vi "ER2007 Get Cell Data.vi"() -> ()   [LabVIEW 2013]
uses:
  <vilib>/Platform/TimedLoop/XDataNode/timing_clust.ctl
  <vilib>/Platform/TimedLoop/XDataNode/nitl_modes.ctl
  <vilib>/Platform/TimedLoop/XDataNode/wakeup.ctl
  Controls/Global ER2007.vi
  <vilib>/platform/TimedLoop/XDataNode/XDataNode.xnode
  <vilib>/Platform/TimedLoop/XDataNode/XDNodeRunTimeDep.lvlib
panel:
  in  "Force Recalc":bool
  out "Last Resistor":T1(ring)
  out "Swch Box":bool[](array[boolean])
  out "NAII Live":bool
  out "HP Live":bool
  out "Cell ID":i32
  out "RS Done":bool
  out "NAI Errcnt":i32
  out "ResistParams":T2 {"R13 (k)" format="%.5f"; "R3G (k)" format="%.5f"; "R23 (k)" format="%.5f"; "R12 (k)" format="%.5f"; "R2P (k)" format="%.5f"}
  out "VI Time":dbl format="%.2f"
  out "B 3":bool
  out "B 2":bool
  out "B 1":bool
  out "Errs":bool[](array[boolean])
  out "SecPh":i32
  out "PriPh":i32
  out "Abort Message":string
  out "Test Info Out":T3 {"Cell Data"."Rw Temp" format="%.2f"; "Cell Data"."Rw" format="%.2f"; "Cell Data"."DAQ Units" items=["Mins", "Hrs"]; "Cell Data"."CurData" format="%.3f"; "Cell Data"."Last Pore Vol" format="%.3f"; "Cell Data"."Amplitude" format="%.3f"; "Cell Data"."ElectSpace" format="%.2f"; "Cell Data"."Permeability" format="%.2f"; "Cell Data"."Porosity" format="%.2f"; "Cell Data"."Diameter" format="%.2f"; "Cell Data"."Length" format="%.2f"}
  in  "Test Info In":T3={"CurCell"=0, "Cell Data"=[{"Cell ID"=1, "Cell Status"=enum."Active", "Project"="Project C1", "Sample #"="Sample C1", "Rock Type"="Rock C1", "Fluid Pair"="Fluid Pair C1", "Rw"=0.0, "Rw Temp"=0.0, "Length"=5.08, "Diameter"=2.54, "Porosity"=1.23, "Permeability"=2.34, "4P"=FALSE, "ElectSpace"=2.54, "Frequency"=1000.0, "Amplitude"=1.0, "DAQ Period"=10, "DAQ Units"=0, "Start Time"=0.0, "Next Time"=0.0, "Datafile"=path "C:/ER2006/Data/Dummy Cell 1 Test.dat", "Last Pore Vol"=9.876, "Last Pore Xdcr"=enum."<none>", "Last Resistor"=enum."<none>", "CurData"=[], "Comment"=""}, {"Cell ID"=2, "Cell Status"=enum."Active", "Project"="Project C2", "Sample #"="Sample C2", "Rock Type"="Rock C2", "Fluid Pair"="Fluid Pair C2", "Rw"=0.0, "Rw Temp"=0.0, "Length"=5.08, "Diameter"=2.54, "Porosity"=2.34, "Permeability"=3.45, "4P"=FALSE, "ElectSpace"=2.54, "Frequency"=1000.0, "Amplitude"=1.0, "DAQ Period"=20, "DAQ Units"=0, "Start Time"=0.0, "Next Time"=0.0, "Datafile"=path "C:/ER2006/Data/Dummy Cell 2 Test.dat", "Last Pore Vol"=8.765, "Last Pore Xdcr"=enum."<none>", "Last Resistor"=enum."<none>", "CurData"=[], "Comment"=""}, {"Cell ID"=3, "Cell Status"=enum."Active", "Project"="Project C3", "Sample #"="Sample C3", "Rock Type"="Rock C3", "Fluid Pair"="Fluid Pair C3", "Rw"=0.0, "Rw Temp"=0.0, "Length"=5.0, "Diameter"=3.7, "Porosity"=3.45, "Permeability"=4.56, "4P"=FALSE, "ElectSpace"=2.54, "Frequency"=20000.0, "Amplitude"=1.0, "DAQ Period"=30, "DAQ Units"=0, "Start Time"=0.0, "Next Time"=0.0, "Datafile"=path "C:/ER2006/Data/Dummy Cell 3 Test.dat", "Last Pore Vol"=7.654, "Last Pore Xdcr"=enum."<none>", "Last Resistor"=enum."Resistor 1", "CurData"=[], "Comment"=""}, {"Cell ID"=4, "Cell Status"=enum."Active", "Project"="Project C4", "Sample #"="Sample C4", "Rock Type"="Rock C4", "Fluid Pair"="Fluid Pair C4", "Rw"=0.0, "Rw Temp"=0.0, "Length"=5.08, "Diameter"=2.54, "Porosity"=4.56, "Permeability"=5.67, "4P"=FALSE, "ElectSpace"=2.54, "Frequency"=1000.0, "Amplitude"=1.0, "DAQ Period"=40, "DAQ Units"=0, "Start Time"=0.0, "Next Time"=0.0, "Datafile"=path "C:/ER2006/Data/Dummy Cell 4 Test.dat", "Last Pore Vol"=6.543, "Last Pore Xdcr"=enum."<none>", "Last Resistor"=enum."<none>", "CurData"=[], "Comment"=""}, {"Cell ID"=5, "Cell Status"=enum."Active", "Project"="Project C5", "Sample #"="Sample C5", "Rock Type"="Rock C5", "Fluid Pair"="Fluid Pair C5", "Rw"=0.0, "Rw Temp"=0.0, "Length"=5.08, "Diameter"=2.54, "Porosity"=5.67, "Permeability"=6.78, "4P"=FALSE, "ElectSpace"=2.54, "Frequency"=1000.0, "Amplitude"=1.0, "DAQ Period"=50, "DAQ Units"=0, "Start Time"=0.0, "Next Time"=0.0, "Datafile"=path "C:/ER2006/Data/Dummy Cell 5 Test.dat", "Last Pore Vol"=5.432, "Last Pore Xdcr"=enum."<none>", "Last Resistor"=enum."Resistor 1", "CurData"=[], "Comment"=""}]} {"Cell Data"."Rw Temp" format="%.2f"; "Cell Data"."Rw" format="%.2f"; "Cell Data"."DAQ Units" items=["Mins", "Hrs"]; "Cell Data"."CurData" format="%.3f"; "Cell Data"."Last Pore Vol" format="%.3f"; "Cell Data"."Amplitude" format="%.3f"; "Cell Data"."ElectSpace" format="%.2f"; "Cell Data"."Permeability" format="%.2f"; "Cell Data"."Porosity" format="%.2f"; "Cell Data"."Diameter" format="%.2f"; "Cell Data"."Length" format="%.2f"}
  in  "DataCell":i32=1 min=1 max=5
  in  "Local Test Resistivity Input Data (sim)":dbl[][][](array[numeric])=[[[1.4142, 0.0], [0.5636, -0.41164], [0.4615, -0.53147], [0.1638, -0.11556]], [[1.4071, 0.0], [1.0986, -3.46], [0.7889, -7.95], [0.4213, -10.11]], [[1.4142, 0.0], [1.0607, 0.0], [0.7071, 0.0], [0.3536, 0.0]], [[1.4142, 0.0], [1.0607, -8.1e-05], [0.7778, -0.000127], [0.4243, -0.000189]], [[1.4142, 0.0], [0.1951, -0.00032], [0.1341, -0.0004], [0.0366, -8e-05]], [[1.4142, 0.0], [0.6923, -1.418851], [0.4974, -1.822365], [0.13, 0.58215]], [[1.4142, 0.0], [0.7408, -0.08646], [0.5387, -0.11405], [0.1347, 0.03607]], [[1.4142, 0.0], [0.6852, -0.060094], [0.4884, -0.071822], [0.1604, -0.002912]]] format="%.5f"
  in  "Use Locals":bool
  out "Resistivity Data":dbl[][](array[numeric]) format="%.5f"
  out "Stored State":T4(ring)
  out "State":T4(ring)
  in  "SimOn":bool
  in  "Stop":bool
  in  "Go":bool
  # "Dev 1 Assignments\n DIO             DigInv\n Chl   Chl Desc  Index\n-----  --------  ------\nP0.0   Shunt 1     0\nP0.1   SCL1        1\nP0.2   SCL2        2\nP0.3   Shunt 2     3\nP0.4   AutoEnb     4\nP0.5   RSCL1       5\nP0.6   Shunt 3     6\nP0.7   RSCL2       7\nP0.8   <spare>     -\nP0.17  <spare>     -\nP0.18  Shunt 4    ??\nP0.21  Shunt 5    ??\nP1.0   RSCL3      16\nP1.1   YCL1       17\nP1.2   YCL2       18\nP1.3   YCL3       19\nP1.4   YCL4       20\nP1.5   <spare>     -\nP1.6   Lockout    21\nP1.7   <spare>     -"
  # "See the Background DAQ vi for A/D\nassignments.  See Frame 0:0 of this\nvi for file and local testing info."
  # "AutoMode   Cell Sel   Resist Sel   Signal Sel"
  # "Dout"
  # "Local Test Controls"
  # "Agilent"
  # "Cell #\n\nVselect\n\nV/Phase"
  # "NAII"
  # "Calc-R"
  # "File I/O"
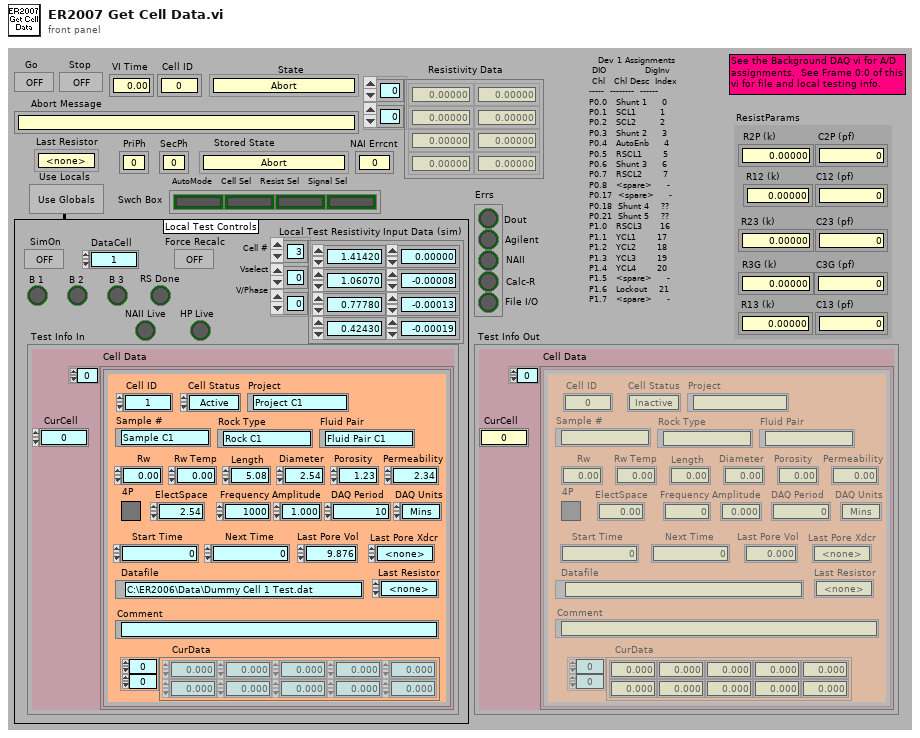
[diagram p1: front panel]
types:
  T1 = enum16{"<none>", "Resistor 1", "Resistor 2", "Resistor 3", "Resistor 4", "Resistor 5", "Resistor 6"}
  T2 = cluster{"R2P (k)":dbl, "C2P (pf)":dbl, "R12 (k)":dbl, "C12 (pf)":dbl, "R23 (k)":dbl, "C23 (pf)":dbl, "R3G (k)":dbl, "C3G (pf)":dbl, "R13 (k)":dbl, "C13 (pf)":dbl}
  T3 = cluster{"CurCell":i32, "Cell Data":cluster{"Cell ID":i32, "Cell Status":enum16{"Inactive", "Setup", "Active", "Done"}, "Project":string, "Sample #":string, "Rock Type":string, "Fluid Pair":string, "Rw":dbl, "Rw Temp":dbl, "Length":dbl, "Diameter":dbl, "Porosity":dbl, "Permeability":dbl, "4P":bool, "ElectSpace":dbl, "Frequency":dbl, "Amplitude":dbl, "DAQ Period":u32, "DAQ Units":u16, "Start Time":dbl, "Next Time":dbl, "Datafile":path, "Last Pore Vol":dbl, "Last Pore Xdcr":enum16{"<none>", "Lo Range", "Hi Range"}, "Last Resistor":enum16{"<none>", "Resistor 1", "Resistor 2", "Resistor 3", "Resistor 4", "Resistor 5", "Resistor 6"}, "CurData":dbl[][], "Comment":string}[]}
  T4 = enum16{"Abort", "Calculate Resistivity Values", "Determine Series Resistor", "Done", "Error Handler", "Final Values", "Generator OFF", "Generator ON", "Get Cell Pressures", "Get Cell Temperatures", "Get Vs & Phase", "Get V1g & Phase", "Get V2g & Phase", "Get V3g & Phase", "Idle", "Initialize", "Main Test Engine", "Reset Auto Mode", "Reset Cell Select Relays", "Reset Resistor Select Relays", "Reset Signal Select Relays", "Set Auto Mode", "Set Cell Select Relays", "Set Freq & Ampltd", "Set Resistor Select Relays", "Set Signal Select Relays", "Stop", "Wait x Secs"}
  T5 = enum16{"<none>", "Signal 1", "Signal 2", "Signal 3"}
  T6 = enum16{"TOTAL", "FUNDAMENTAL", "IN PHASE", "QUADRATURE", "PHASE ANGLE", "THD"}
  T7 = cluster{"Rseries (K)":dbl, "Frequency (Hz)":dbl, "Voltages":dbl[], "Angles":dbl[]}
  T8 = typedef "XDNodeRunTimeDep.lvlib/timing_clust.ctl" = cluster{"Expected End [f-1]":u64, "Actual End [f-1]":u64, "Finished Late? [f-1]":bool, "Expected End [i-1]":u64, "Actual End [i-1]":u64, "Finished Late? [i-1]":bool, "Expected Start [i]":u64, "Actual Start [i]":u64, "Expected Start [f]":u64, "Actual Start [f]":u64, "Source Name":string, "Structure Name":string, "Period":i64, "Deadline":i64, "Offset":i64, "Start":i64, "Priority":i32, "Timeout":i32, "Mode":T9, "Wakeup Reason":T10, "Error":errorcluster, "Source Type":string, "Secondary Source Type":string, "Global End Time":u64, "Global Start Time":u64, "Frame Duration":u64, "Iteration Duration":u64, "Assigned CPU":i32, "I/O Scan Engine Mode":u32}
  T9 = typedef "XDNodeRunTimeDep.lvlib/nitl_modes.ctl" = enum32{"No Change", "Process missed periods, maintain original phase", "Discard missed periods, maintain original phase", "Process missed periods, ignore original phase", "Discard missed periods, ignore original phase"}
  T10 = typedef "XDNodeRunTimeDep.lvlib/wakeup.ctl" = enum32{"Normal", "Aborted", "Asynchronous wakeup", "Timing source error", "Timed loop error", "Timeout"}
  T11 = cluster{"Cell ID":i32, "Cell Status":enum16{"Inactive", "Setup", "Active", "Done"}, "Project":string, "Sample #":string, "Rock Type":string, "Fluid Pair":string, "Rw":dbl, "Rw Temp":dbl, "Length":dbl, "Diameter":dbl, "Porosity":dbl, "Permeability":dbl, "4P":bool, "ElectSpace":dbl, "Frequency":dbl, "Amplitude":dbl, "DAQ Period":u32, "DAQ Units":u16, "Start Time":dbl, "Next Time":dbl, "Datafile":path, "Last Pore Vol":dbl, "Last Pore Xdcr":enum16{"<none>", "Lo Range", "Hi Range"}, "Last Resistor":enum16{"<none>", "Resistor 1", "Resistor 2", "Resistor 3", "Resistor 4", "Resistor 5", "Resistor 6"}, "CurData":dbl[][], "Comment":string}
  T12 = cluster{"Cell ID":i32, "Cell Status":enum16{"Inactive", "Setup", "Active", "Done"}, "Project":string, "Sample #":string, "Rock Type":string, "Fluid Pair":string, "Rw":dbl, "Rw Temp":dbl, "Length":dbl, "Diameter":dbl, "Porosity":dbl, "Permeability":dbl, "4P":bool, "ElectSpace":dbl, "Frequency":dbl, "Amplitude":dbl, "DAQ Period":u32, "DAQ Units":u16, "Start Time":dbl, "Next Time":dbl, "Datafile":path, "Last Pore Vol":dbl, "Last Pore Xdcr":enum16{"<none>", "Lo Range", "Hi Range"}, "Last Resistor":enum16{"<none>", "Resistor 1", "Resistor 2", "Resistor 3", "Resistor 4", "Resistor 5", "Resistor 6"}, "CurData":dbl[][], "Comment":string}[]
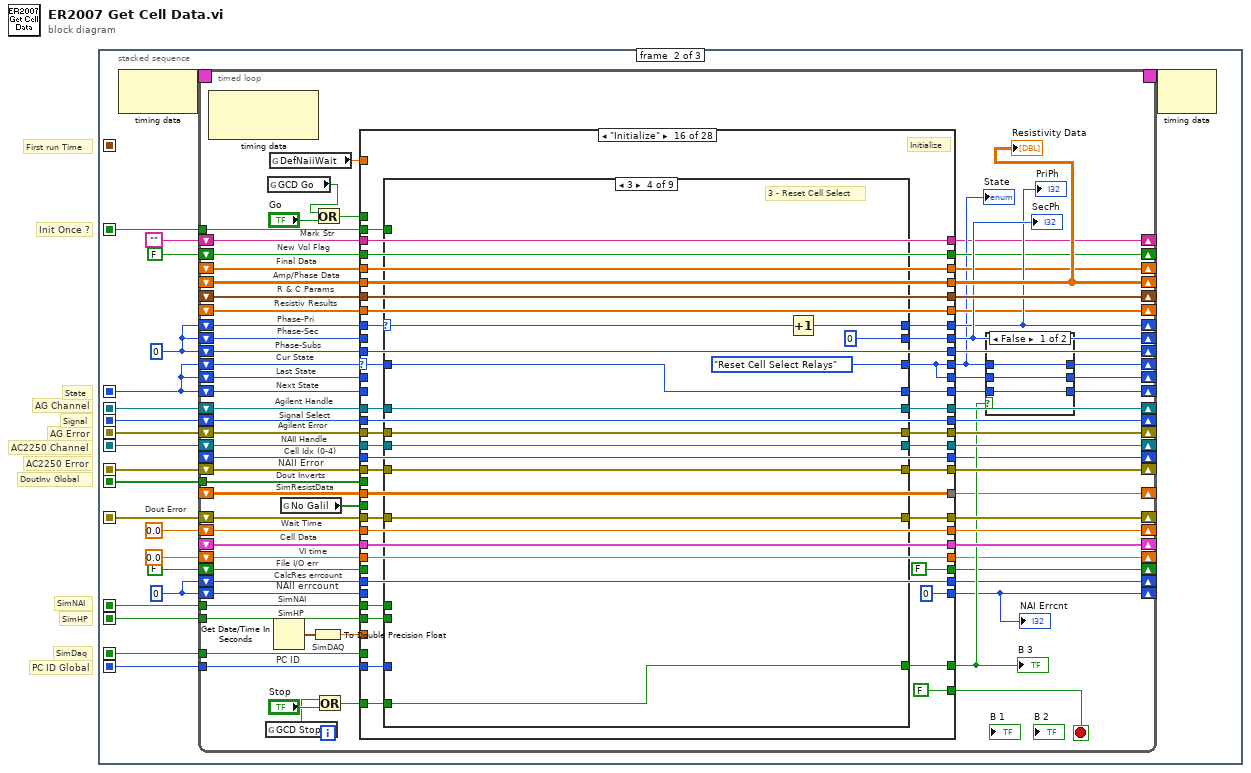
[diagram p0: block diagram]
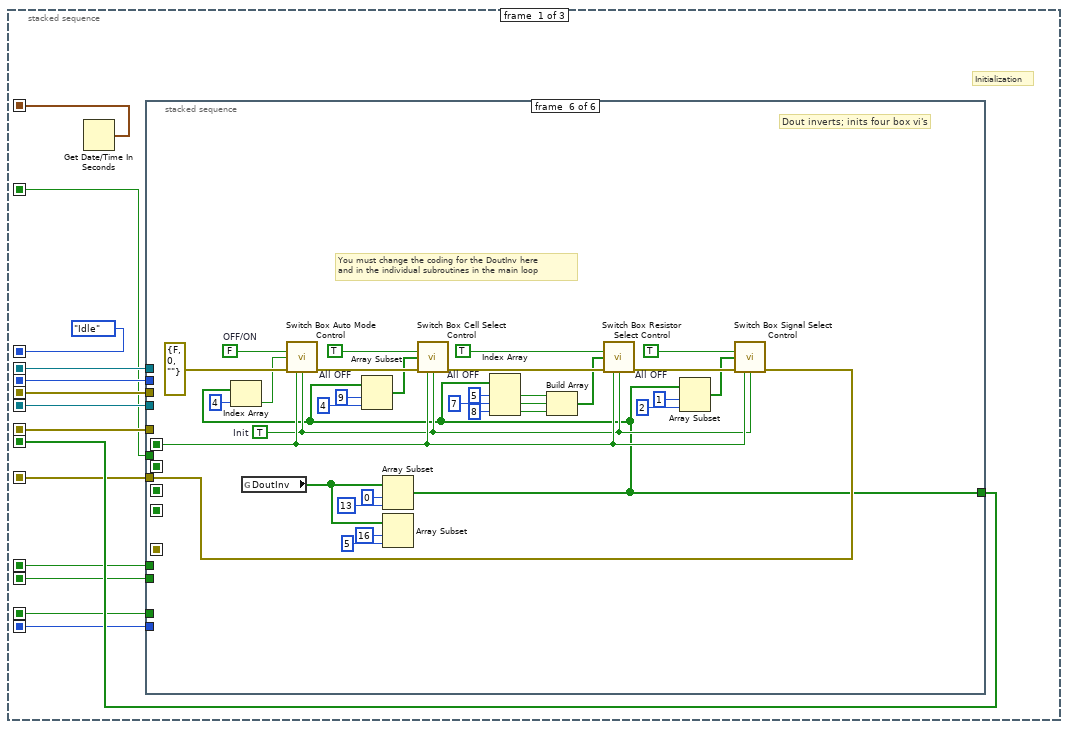
[diagram p2: hidden frame]
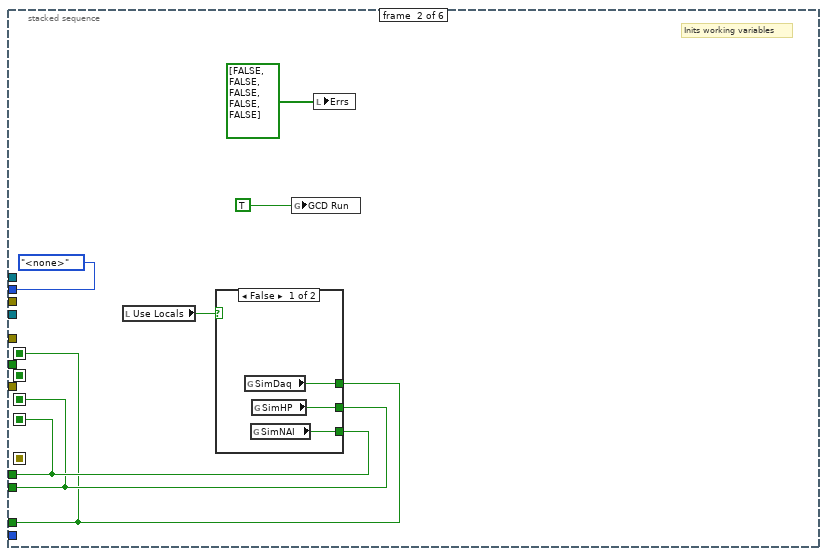
[diagram p4: hidden frame]
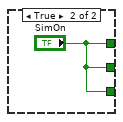
[diagram p5: hidden frame]
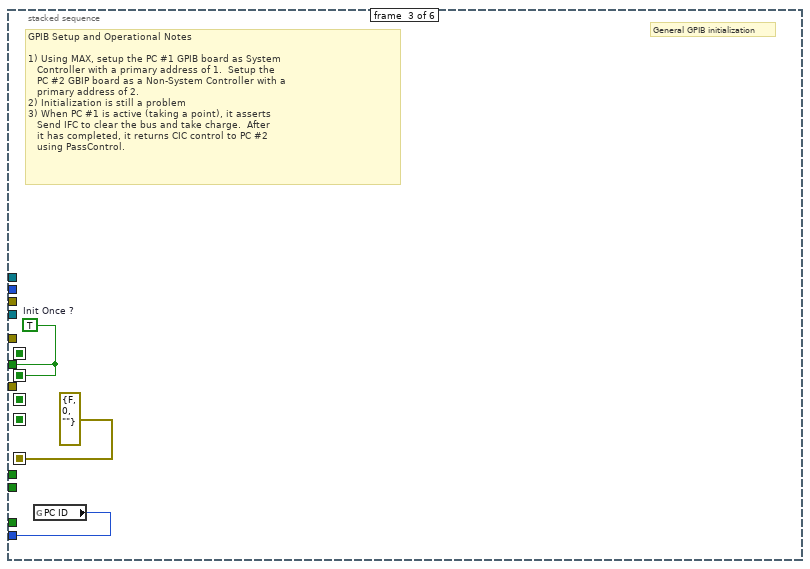
[diagram p6: hidden frame]
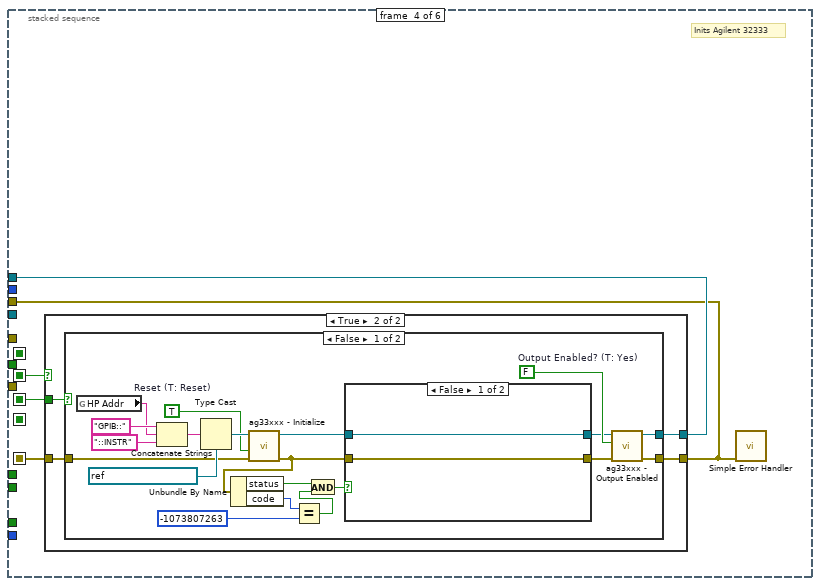
[diagram p7: hidden frame]
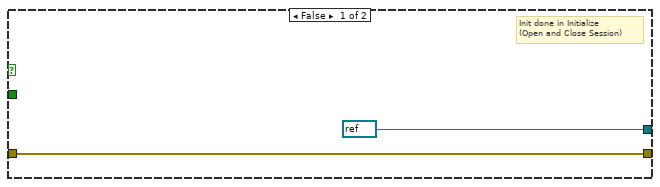
[diagram p8: hidden frame]
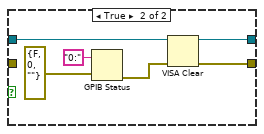
[diagram p9: hidden frame]
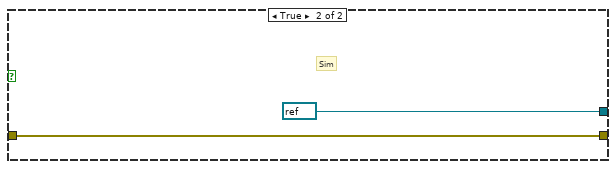
[diagram p10: hidden frame]
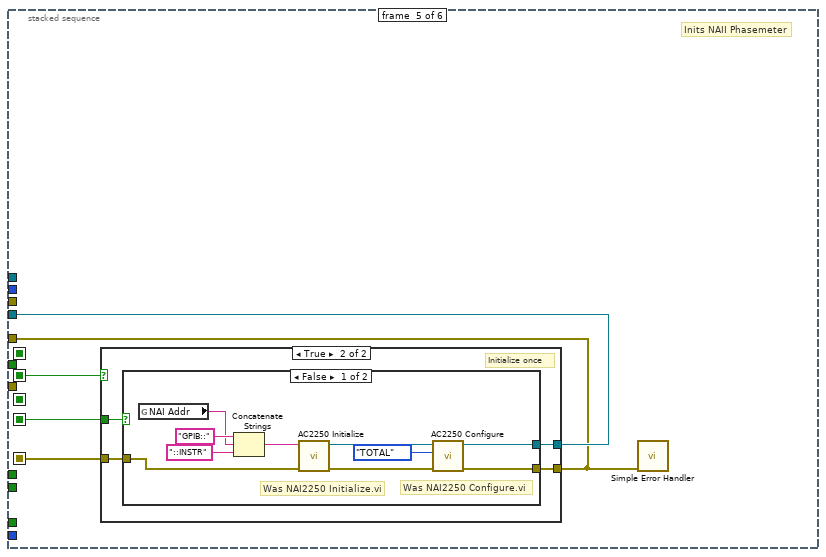
[diagram p11: hidden frame]
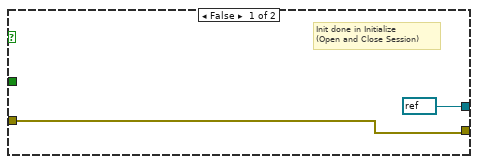
[diagram p12: hidden frame]
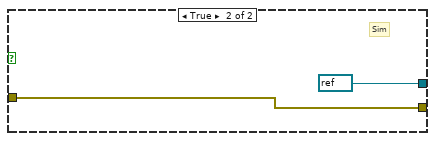
[diagram p13: hidden frame]
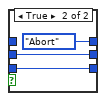
[diagram p14: hidden frame]
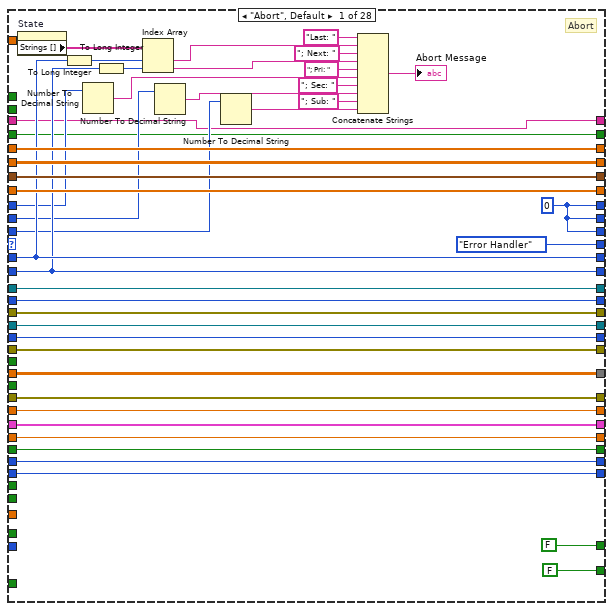
[diagram p15: hidden frame]
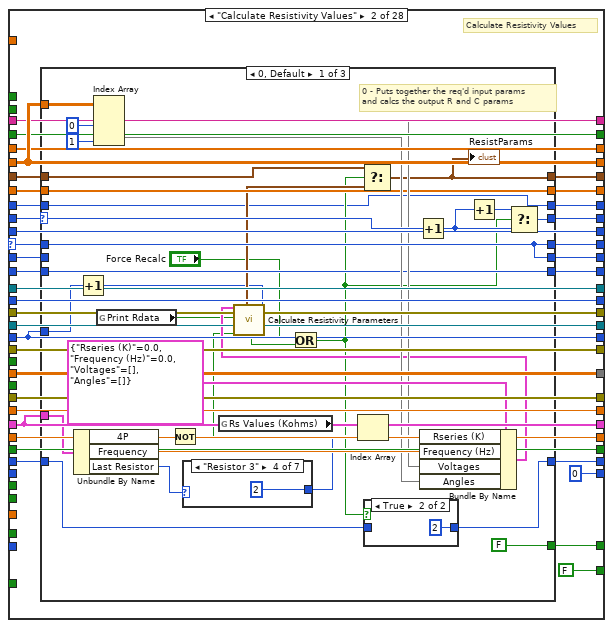
[diagram p16: hidden frame]
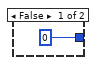
[diagram p17: hidden frame]
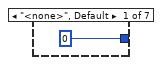
[diagram p18: hidden frame]
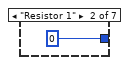
[diagram p19: hidden frame]
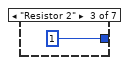
[diagram p20: hidden frame]
diagram:
  # "First run Time"
  # "PC ID Global"
  # "DoutInv Global"
  # "AC2250 Error"
  # "AC2250 Channel"
  # "AG Error"
  # "AG Channel"
  # "Init Once ?"
  # "SimNAI"
  # "SimHP"
  # "SimDaq"
  # "Signal"
  # "State"
  n1 = stacked-sequence {
    seq-local: [w14 _ _] -> [_ w146 _]
    seq-local: [T4."Idle" ("State") _ _] -> [_ w141 _]
    seq-local: [w13 _ _] -> [_ w137 _]
    seq-local: [w12 _ _] -> [_ w144 _]
    seq-local: [w11 _ _] -> [_ w142 w3963]
    seq-local: [w10 _ _] -> [_ _ _]
    seq-local: [w9 _ _] -> [_ w138 w3964]
    seq-local: [w8 _ _] -> [_ w139 _]
    seq-local: [w4 _ _] -> [_ w135 _]
    seq-local: [w5 _ _] -> [_ w136 _]
    seq-local: [w6 _ _] -> [_ w134 _]
    seq-local: [w7 _ _] -> [_ w133 _]
    seq-local: [w2 _ _] -> [_ w130 _]
    seq-local: [w1 _ _] -> [_ w129 _]
    frame #0 {
      # "Initialization"
      n2 = Get Date/Time In Seconds() -> (seconds since 1Jan1904=w10:timestamp)
      n3 = stacked-sequence {
        seq-local: [_ w20 _ _ _ _] -> [_ _ _ _ w73 _]
        seq-local: [_ w19 _ _ _ _] -> [_ _ _ w33 _ _]
        seq-local: [_ w18 _ _ _ _] -> [_ _ _ _ _ w103]
        seq-local: [_ _ errorcluster {"status"=FALSE, "code"=0, "source"=""} ("error out") _ _ _] -> [_ _ _ w30 w71 _]
        seq-local: [_ _ w27 _ _ _] -> [_ _ _ w29 w70 _]
        tunnel: [_ _ _ _ _ w100] -> w14
        tunnel: [_ _ _ w31 _ _] -> w13
        tunnel: [_ T5."<none>" ("Signal") _ _ _ _] -> w12
        tunnel: [_ w20 _ _ _ _] -> w11
        tunnel: [_ w19 _ _ _ _] -> w9
        tunnel: [_ w18 _ _ _ _] -> w8
        tunnel: [_ _ _ w32 _ _] -> w7
        tunnel: [_ _ _ _ w74 _] -> w6
        tunnel: [_ _ _ _ w72 _] -> w5
        tunnel: [_ _ _ _ _ w104] -> w4
        tunnel: [_ _ w27 _ _ _] -> w2
        tunnel: [_ _ w26 _ _ _] -> w1
        frame #0 {
          # "New Data File Format-Data Line\n\n                        Reals\nCol #  Process Variable Col #\n----- ----------------- -----\n  1   Point Flag\n  2   Point Date\n  3   Point Time\n  4   Elapsed Time (hrs)   1\n  5   ER 1-2               2\n  6   ER 1-3               3\n  7   ER 1-4               4\n  8   ER 2-3               5\n  9   F 2-3                6\n 10   T-A                  7\n 11   T-B                  8\n 12   Conf P (ER2005 NOP)  9\n 13   Pore P (ER2005 Pc)  10\n 14   Delta-P             11\n 15   Downstrm P (Pc-d)   12\n 16   Produced Vol        13\n 17   C14                 14\n 18   C23                 15\n 19   Comment"
          # "Simulated Test Data - To use simulated voltage and phase data (Local Test Resistivity Input Data (sim)), press \"Use Locals\"\n                      and the \"SimOn\" buttons, set the \"Data Cell\" index (1 = cell #1), set info in \"Test Info In\", start\n                      the Get Cell Data.vi, and press \"Go\".\n\nCell# Freq Rseries   R12    R23    R3G    C12    C23    C3G    Vs      Ps      V1g    P1g      V2g    P2g      V3g     P3g\n----- ---- ------- ------ ------ ------ ------ ------ ------ ------ -------- ------ -------- ------ -------- ------ --------\n  1   1000    1K   0.1200 0.3500 0.1930   3300   8200   5600 1.4142  0.00000 0.5636 -0.41164 0.4615 -0.53147 0.1638 -0.11556\n  2   1000    1K   1.0050 1.2010 1.4690  10000  22000  47000 1.4071  0.00000 1.0986 -3.46000 0.7889 -7.95000 0.4213 -10.1100\n  3   1000    10   0.0100 0.0100 0.0100      0      0      0 1.4142  0.00000 1.0607  0.00000 0.7071  0.00000 0.3536  0.00000\n  4   1000   100   0.0800 0.1000 0.1200   6800   8200  10000 1.4142  0.00000 1.0607 -0.00008 0.7778 -0.00013 0.4243 -0.00019\n  5   1000    10   0.0005 0.0008 0.0003   1000   2000   1200 1.4142  0.00000 0.1951 -0.00032 0.1341 -0.00040 0.0366 -0.00008\n  6A  1000  100K   27.000 51.000 18.000 180000 220000 120000\n  6B  1000   10K   3.0000 5.0000 2.0000 100000 120000  82000\n  6C  1000   10K   2.7000 4.5000 2.2000  90000 100000  75000"
          # "Old Data File Format - Data Line\n\nCol #  Process Variable\n----- -----------------\n  1   Elapsed Time (hrs)\n  2   ER 1-2\n  3   ER 1-3\n  4   ER 1-4\n  5   ER 2-3\n  6   F 2-3\n  7   T-A\n  8   T-B\n  9   NOP\n 10   Pc\n 11   Displaced Vol\n 12   C14\n 13   C23"
          # "Data File Format - Header\n\n1 - Start Date\n2 - Start Time\n3 - Filename\n4 - Project\n5 - Sample ID\n6 - Rock Type\n7 - Fluid Pair\n8 - Rw\n9 - Rt\n10 - Frequency\n11 - Amplitude\n12 - DAQ Period (mins)\n13 - Length\n14 - Diameter\n15 - Porosity\n16 - Permeability\n17 - Electrode Spacing"
          # "Notes and such"
        }
        frame #1 {
          # "Inits working variables"
          n4 = local read "Use Locals"() -> (w17:bool)
          n5 = case shown="False" w17 {
            tunnel: [w24 "SimOn"] -> w18
            tunnel: [w23 "SimOn"] -> w20
            tunnel: [w22 "SimOn"] -> w19
            frame False {
              n6 = global read "Global ER2007.vi" "SimDaq"() -> (w24:bool)
              n7 = global read "Global ER2007.vi" "SimNAI"() -> (w23:bool)
              n8 = global read "Global ER2007.vi" "SimHP"() -> (w22:bool)
            }
            frame True {
            }
          }
          n9 = global write "Global ER2007.vi" "GCD Run"(TRUE ("GCD Run")) -> ()
          n10 = local write "Errs"(bool[] [FALSE, FALSE, FALSE, FALSE, FALSE] ("Errs")) -> ()
        }
        frame #2 {
          w27 = TRUE  # Init Once ?
          # "General GPIB initialization"
          # "GPIB Setup and Operational Notes\n\n1) Using MAX, setup the PC #1 GPIB board as System\n   Controller with a primary address of 1.  Setup the\n   PC #2 GBIP board as a Non-System Controller with a\n   primary address of 2.\n2) Initialization is still a problem\n3) When PC #1 is active (taking a point), it asserts\n   Send IFC to clear the bus and take charge.  After\n   it has completed, it returns CIC control to PC #2\n   using PassControl."
          n11 = global read "Global ER2007.vi" "PC ID"() -> (w26:i32)
        }
        frame #3 {
          # "Inits Agilent 32333"
          n12 = case shown="True" w29 {
            tunnel: w33 -> [_ w39]
            tunnel: [refnum<visa-resource-name> refnum ("dup VISA session") w38] -> w32
            tunnel: [w34 w37] -> w31
            tunnel: w30 -> [w34 w36]
            frame False {
              # "Init done in Initialize\n(Open and Close Session)"
            }
            frame True {
              n13 = case shown="False" w39 {
                tunnel: [w52 refnum<visa-resource-name> refnum ("dup VISA session")] -> w38
                tunnel: [w51 w68] -> w37
                tunnel: w36 -> [w49 w68]
                frame False {
                  w53 = FALSE  # Output Enabled? (T: Yes)
                  w54 = TRUE  # Reset (T: Reset)
                  n14 = global read "Global ER2007.vi" "HP Addr"() -> (w50:string)
                  n15 = Concatenate Strings("GPIB::" ("string"), w50, "::INSTR" ("string")) -> (w56:string)
                  n16 = Type Cast(type=refnum<visa-resource-name> "GPIB::10::INSTR" ("Instrument Resource Name"), x=w56) -> (*(type *) &x=w55:refnum<visa-resource-name>)
                  n17 = call "ag33xxx - Initialize.vi"("error in (no error)"=w49, "Reset (T: Reset)"=w54, "Instrument Resource Name"=w55) -> ("error out"=w48:errorcluster, "dup VISA session"=w41:refnum<visa-resource-name>)  [unwired: 7 in]
                  n18 = Unbundle By Name(w48) -> ("status"=w44:bool, "code"=w46:i32)
                  n19 = Equal?(x=w46, y=-1073807263) -> (x = y?=w45:bool)
                  n20 = And(x=w44, y=w45) -> (x .and. y?=w43:bool)
                  n21 = case shown="False" w43 {
                    tunnel: w48 -> [w61 _]
                    tunnel: [w61 w65] -> w42
                    tunnel: w41 -> [w60 w62]
                    tunnel: [w60 w64] -> w40
                    frame False {
                    }
                    frame True {
                      n22 = GPIB Status(0:"0:" ("address string"), 1:errorcluster {"status"=FALSE, "code"=0, "source"=""} ("error out")) -> (5:w63:errorcluster)  [unwired: 3 out]
                      n23 = VISA Clear(VISA resource name=w62, error in (no error)=w63) -> (VISA resource name out=w64:refnum<visa-resource-name>, error out=w65:errorcluster)
                    }
                  }
                  n24 = call "ag33xxx - Output Enabled.vi"("error in (no error)"=w42, "Output Enabled? (T: Yes)"=w53, "VISA session"=w40) -> ("error out"=w51:errorcluster, "dup VISA session"=w52:refnum<visa-resource-name>)  [unwired: 7 in]
                }
                frame True {
                  # "Sim"
                }
              }
            }
          }
          n25 = call <vilib>:"Simple Error Handler.vi"("error in (no error)"=w31) -> ()  [unwired: 4 in, 5 out]
        }
        frame #4 {
          # "Inits NAII Phasemeter"
          n26 = case shown="True" w70 {
            tunnel: [refnum<visa-resource-name> refnum ("instrument handle out") w80] -> w74
            tunnel: w73 -> [_ w79]
            tunnel: [w75 w78] -> w72
            tunnel: w71 -> [w75 w77]
            frame False {
              # "Init done in Initialize\n(Open and Close Session)"
            }
            frame True {
              # "Initialize once"
              n27 = case shown="False" w79 {
                tunnel: [w82 refnum<visa-resource-name> refnum ("instrument handle out")] -> w80
                tunnel: [w84 w91] -> w78
                tunnel: w77 -> [w87 w91]
                frame False {
                  # "Was NAI2250 Configure.vi"
                  # "Was NAI2250 Initialize.vi"
                  n28 = global read "Global ER2007.vi" "NAI Addr"() -> (w88:string)
                  n29 = Concatenate Strings("GPIB::" ("string"), w88, "::INSTR" ("string")) -> (w86:string)
                  n30 = call "AC2250 Initialize.vi"("ErrIn"=w87, "VISA Resource Name In"=w86) -> ("ErrOut"=w85:errorcluster, "VISA Resource Name Out"=w83:refnum<visa-resource-name>)  [unwired: 8 in]
                  n31 = call "AC2250 Configure.vi"("ErrIn"=w85, "Measurement Mode"=T6."TOTAL", "VISA Resource Name In"=w83) -> ("ErrOut"=w84:errorcluster, "VISA Resource Name Out"=w82:refnum<visa-resource-name>)  [unwired: 6 in, 1 out]
                }
                frame True {
                  # "Sim"
                }
              }
            }
          }
          n32 = call <vilib>:"Simple Error Handler.vi"("error in (no error)"=w72) -> ()  [unwired: 4 in, 5 out]
        }
        frame #5 {
          w108 = TRUE  # All OFF
          w110 = TRUE  # All OFF
          w113 = TRUE  # All OFF
          w102 = TRUE  # Init
          w118 = FALSE  # OFF/ON
          # "You must change the coding for the DoutInv here\nand in the individual subroutines in the main loop"
          # "Dout inverts; inits four box vi's"
          n33 = global read "Global ER2007.vi" "DoutInv"() -> (w101:bool[])
          n34 = Array Subset(array=w101, index=0, length=13) -> (w100:bool[])
          n35 = Index Array(array=w100, index=4) -> (element=w117:bool)
          n36 = call "Switch Box Auto Mode Control.vi"("OFF/ON"=w118, "Invert"=w117, "ErrIn"=errorcluster {"status"=FALSE, "code"=0, "source"=""}, "SimOn"=w103, "Init"=w102) -> ("ErrOut"=w116:errorcluster)  [unwired: 10 in]
          n37 = Array Subset(array=w100, index=9, length=4) -> (w112:bool[])
          n38 = Array Subset(array=w101, index=16, length=5) -> ()  [unwired: 1 out]
          n39 = call "Switch Box Cell Select Control.vi"("All OFF"=w113, "Dout Inv"=w112, "ErrIn"=w116, "SimOn"=w103, "Init"=w102) -> ("ErrOut"=w111:errorcluster)  [unwired: 10 in]
          n40 = Index Array(array=w100, index #1=5 ("index"), index #2=7 ("index"), index #3=8 ("index")) -> (element #1=w96:bool, element #2=w95:bool, element #3=w94:bool)
          n41 = Build Array(w96, w95, w94) -> (w93:bool[])
          n42 = call "Switch Box Resistor Select Control.vi"("All OFF"=w110, "Dout Inv"=w93, "ErrIn"=w111, "SimOn"=w103, "Init"=w102) -> ("ErrOut"=w109:errorcluster)  [unwired: 10 in]
          n43 = Array Subset(array=w100, index=1, length=2) -> (w105:bool[])
          n44 = call "Switch Box Signal Select Control.vi"("All OFF"=w108, "Dout Inv"=w105, "ErrIn"=w109, "SimOn"=w103, "Init"=w102) -> ("ErrOut"=w104:errorcluster)  [unwired: 10 in]
        }
      }
    }
    frame #1 {
      w127 = 0
      w143 = 0 ("Samps/Chl")
      # "Dout Error"
      n45 = node-c288() -> (w125:T8)  [unwired: 1 in]
      n46 = timed-loop {
        shift-left: "" -> [w148]
        shift-right: [w147] -> _
        tunnel: w129 -> [w149]
        tunnel: w130 -> [w150]
        shift-left: FALSE -> [w156]
        shift-right: [w157] -> _
        shift-left: 0.0 -> [w158]
        shift-right: [w159] -> _
        shift-left: _ -> [w163]
        shift-right: [w162] -> _
        shift-left: _ -> [w160]
        shift-right: [w161] -> _
        tunnel: w138 -> [w166]
        tunnel: w139 -> [w165]
        shift-left: w127 -> [w170]
        shift-right: [w169] -> _
        shift-left: FALSE -> [w168]
        shift-right: [w167] -> _
        shift-left: w127 -> [w171]
        shift-right: [w164] -> _
        tunnel: w142 -> [w175]
        shift-left: _ -> [w180]
        shift-right: [w172] -> _
        shift-left: _ -> [w182]
        shift-right: [w173] -> _
        shift-left: _ -> [w183]
        shift-right: [w184] -> _
        shift-left: _ -> [w185]
        shift-right: [w178] -> _
        shift-left: w143 -> [w187]
        shift-right: [w186] -> _
        shift-left: w144 -> [w191]
        shift-right: [w190] -> _
        shift-left: 0.0 -> [w193]
        shift-right: [w192] -> _
        shift-left: _ -> [w195]
        shift-right: [w194] -> _
        shift-left: w135 -> [w197]
        shift-right: [w196] -> _
        shift-left: w141 -> [w204]
        shift-right: [w201] -> _
        shift-left: w143 -> [w210]
        shift-right: [w176] -> _
        shift-left: w141 -> [w206]
        shift-right: [w203] -> _
        shift-left: w133 -> [w212]
        shift-right: [w211] -> _
        shift-left: w137 -> [w209]
        shift-right: [w213] -> _
        shift-left: w143 -> [w214]
        shift-right: [w177] -> _
        tunnel: w146 -> [w216]
        shift-left: w141 -> [w205]
        shift-right: [w202] -> _
        shift-left: w134 -> [w217]
        shift-right: [w218] -> _
        shift-left: w136 -> [w208]
        shift-right: [w215] -> _
        timing-out: [_] -> w126
        timing: w125 -> [_]
        stop <- w198 stop-if-true
        # "SimResistData"
        # "Mark Str"
        # "PC ID"
        # "New Vol Flag"
        # "VI time"
        # "SimHP"
        # "SimNAI"
        # "CalcRes errcount"
        # "File I/O err"
        # "NAII errcount"
        # "SimDAQ"
        # "Final Data"
        # "Phase-Subs"
        # "Signal Select"
        # "Wait Time"
        # "NAII Error"
        # "Agilent Handle"
        # "Agilent Error"
        # "NAII Handle"
        # "Cell Data"
        # "Cell Idx (0-4)"
        # "Resistiv Results"
        # "R & C Params"
        # "Amp/Phase Data"
        # "Dout Inverts"
        # "Phase-Sec"
        # "Phase-Pri"
        # "Last State"
        # "Next State"
        # "Cur State"
        n47 = node-c288() -> ()  [unwired: 1 in, 2 out]
        n48 = global read "Global ER2007.vi" "GCD Stop"() -> (w152:bool)
        n49 = global read "Global ER2007.vi" "GCD Go"() -> (w154:bool)
        n50 = global read "Global ER2007.vi" "DefNaiiWait"() -> (w153:dbl)
        n51 = Get Date/Time In Seconds() -> (seconds since 1Jan1904=w189:timestamp)
        n52 = global read "Global ER2007.vi" "No Galil"() -> (w151:bool[])
        n53 = To Double Precision Float(number=w189) -> (double precision float=w188:dbl)
        n54 = Or(x=w154, y="Go") -> (x .or. y?=w181:bool)
        n55 = Or(x=w152, y="Stop") -> (x .or. y?=w207:bool)
        n56 = case shown="\"Initialize\"" w206 {
          selector: w206 -> [_ w302 w452 w752 w917 w1177 w1669 w1706 w1741 w1773 w1820 w2006 w2285 w2538 w2794 w2997 w3178 w3439 w3477 w3519 w3557 w3594 w3631 w3662 w3714 w3751 w3779 w3943]
          tunnel: [w267 w293 w445 w748 w915 w1168 w1663 w1700 w1736 w1768 w1811 w1997 w2276 w2529 w2777 w2987 w3193 w3435 w3473 w3515 w3553 w3590 w3627 w3657 w3710 w3747 w3755 w3950] -> w218
          tunnel: w175 -> [_ _ w422 w742 w912 _ _ _ _ _ w1801 w1987 w2266 w2519 _ w2967 _ _ _ _ _ _ _ _ _ _ w3759 _]
          tunnel: w217 -> [w267 w293 w445 w750 w916 w1168 w1663 w1700 w1736 w1768 w1813 w1999 w2278 w2531 w2777 w2988 w3193 w3435 w3473 w3515 w3553 w3590 w3627 w3657 w3710 w3747 w3760 w3950]
          tunnel: w216 -> [_ _ _ _ _ _ _ _ _ _ _ _ _ _ _ _ _ w3432 w3470 w3512 w3550 w3587 w3624 _ w3676 w3744 w3763 _]
          tunnel: w185 -> [w261 w288 w431 w773 w943 w1179 w1656 w1693 w1735 w1767 w1803 w1989 w2268 w2521 w2787 w2980 w3173 w3427 w3464 w3507 w3544 w3582 w3618 w3648 w3704 w3739 w3782 w3935]
          tunnel: [w266 w292 w444 w747 w913 w1167 w1664 w1701 w1744 w1776 w1810 w1996 w2275 w2528 w2774 w2989 w3191 w3434 w3472 w3514 w3552 w3589 w3626 w3656 w3709 w3746 w3772 w3951] -> w215
          tunnel: w214 -> [w242 w305 w455 w768 w940 w1153 w1670 w1707 w1743 w1775 w1825 w2011 w2290 w2543 w2764 _ _ w3440 w3478 w3520 w3558 w3595 w3632 w3649 w3715 w3752 _ w3944]
          tunnel: [w229 w304 w453 w768 w940 w1153 w1670 w1707 w1743 w1775 w1825 w2011 w2290 w2543 w2798 w2991 w3196 w3440 w3478 w3520 w3558 w3595 w3632 w3649 w3715 w3752 w3790 w3944] -> w177
          tunnel: [w268 w294 w446 w744 w909 w1169 w1658 w1695 w1737 w1769 w1814 w2000 w2279 w2532 w2775 w3000 w3192 w3436 w3474 w3516 w3554 w3591 w3628 w3654 w3711 w3748 w3774 w3949] -> w213
          tunnel: w212 -> [w269 w296 w447 w746 w911 w1173 w1660 w1697 w1739 w1771 w1816 w2002 w2281 w2534 w2791 w2985 w3194 w3437 w3475 w3517 w3555 w3592 w3629 w3659 w3712 w3749 w3762 w3948]
          tunnel: [w269 w296 w447 w743 w910 w1173 w1659 w1696 w1739 w1771 w1816 w2002 w2281 w2534 w2791 w2998 w3194 w3437 w3475 w3517 w3555 w3592 w3629 w3658 w3712 w3749 w3756 w3948] -> w211
          tunnel: [w229 w271 w454 w769 w924 w1155 w1671 w1708 w1746 w1779 w1824 w2010 w2289 w2542 w2799 w2992 w3197 w3441 w3479 w3521 w3559 w3596 w3633 w3663 w3716 w3753 w3791 w3945] -> w176
          tunnel: w210 -> [w246 w270 w454 w775 w925 w1154 w1671 w1708 w1746 w1779 w1824 w2010 w2289 w2542 w2796 w3001 w3198 w3441 w3479 w3521 w3559 w3596 w3633 w3663 w3716 w3753 w3792 w3945]
          tunnel: w209 -> [w268 w294 w446 w745 w922 w1169 w1661 w1698 w1737 w1769 w1814 w2000 w2279 w2532 w2775 w2999 w3192 w3436 w3474 w3516 w3554 w3591 w3628 w3660 w3711 w3748 w3774 w3949]
          tunnel: w208 -> [w266 w292 w444 w749 w914 w1167 w1664 w1701 w1744 w1776 w1812 w1998 w2277 w2530 w2774 w2990 w3191 w3434 w3472 w3514 w3552 w3589 w3626 w3656 w3709 w3746 w3772 w3951]
          tunnel: w207 -> [_ _ w438 w754 w919 w1165 _ _ _ _ w1827 w2013 w2292 w2545 w2765 w2994 w3184 _ _ _ _ _ _ _ _ _ _ w3923]
          tunnel: [FALSE w289 w437 w737 FALSE w1164 w1644 w1680 FALSE FALSE w1828 w2014 w2293 w2546 w2766 w2993 w3185 w3410 w3447 w3491 w3527 w3565 w3602 w3635 w3688 w3722 FALSE ("Error") w3922] -> w174
          tunnel: w205 -> [w255 w301 w451 _ w938 w1172 _ _ _ _ w1817 w2003 w2282 w2535 _ _ w3179 _ _ _ _ _ _ _ _ _ _ w3942]
          tunnel: w204 -> [w253 w300 w450 _ w937 w1171 w1668 w1705 w1740 w1772 w1819 w2005 w2284 w2537 _ _ w3180 w3438 w3476 w3518 w3556 w3593 w3630 w3661 w3713 w3750 _ w3924]
          tunnel: [T4."Error Handler" ("State") w297 w449 w753 w918 w1176 w1668 w1705 w1740 w1772 w1822 w2008 w2287 w2540 w2795 w2996 w3183 w3438 w3476 w3518 w3556 w3593 w3630 w3661 w3713 w3750 w3778 w3939] -> w155
          tunnel: [w255 w298 w448 w752 w938 w1175 w1669 w1706 w1741 w1773 w1818 w2004 w2283 w2536 w2793 w2996 w3182 w3439 w3477 w3519 w3557 w3594 w3631 w3662 w3714 w3751 w3776 w3940] -> w199
          tunnel: [w253 w299 w436 w752 w937 w1174 w1668 w1705 w1740 w1772 w1821 w2007 w2286 w2539 w2792 w2995 w3181 w3438 w3476 w3518 w3556 w3593 w3630 w3661 w3713 w3750 w3777 w3941] -> w200
          tunnel: [FALSE FALSE FALSE FALSE ("OK") FALSE w1158 FALSE FALSE FALSE FALSE FALSE FALSE FALSE FALSE w2766 FALSE FALSE FALSE FALSE FALSE FALSE FALSE FALSE FALSE FALSE FALSE w3785 FALSE] -> w198
          tunnel: w197 -> [w265 w291 w443 w751 w923 w1166 w1667 w1704 w1726 w1777 w1809 w1995 w2274 w2527 w2773 w2974 w3190 w3419 w3456 w3499 w3536 w3574 w3609 w3655 w3696 w3729 w3766 w3953]
          tunnel: [w265 w291 w443 w751 w923 w1166 w1667 w1704 w1726 w1777 w1809 w1995 w2274 w2527 w2773 w2973 w3190 w3418 w3455 w3498 w3535 w3573 w3608 w3655 w3695 w3728 w3765 w3953] -> w196
          tunnel: w160 -> [w233 w276 w421 w766 w929 w1147 w1647 w1684 w1721 w1754 w1791 w1972 w2256 w2508 w2776 w2975 w3166 w3413 w3451 w3495 w3531 w3569 w3606 w3639 w3692 w3726 w3773 w3927]
          tunnel: w195 -> [w264 w277 w442 w761 w934 w1161 w1665 w1702 w1720 w1753 w1808 w1994 w2273 w2526 w2771 w2984 w3195 w3431 w3468 w3511 w3548 w3586 w3622 w3653 w3708 w3742 w3770 w3952]
          tunnel: [w264 w277 w439 w761 w934 w1156 w1665 w1702 w1720 w1753 w1807 w1993 w2272 w2525 w2772 w2984 w3187 w3431 w3468 w3511 w3548 w3586 w3622 w3653 w3708 w3742 w3770 w3952] -> w194
          tunnel: w193 -> [w263 w290 w441 w756 w935 w1146 w1666 w1703 w1745 w1778 w1805 w1991 w2270 w2523 w2762 w2983 w3189 w3430 w3467 w3510 w3547 w3585 w3621 w3652 w3707 w3741 w3767 w3947]
          tunnel: [w263 w290 w440 w763 w935 w1145 w1666 w1703 w1745 w1778 w1806 w1992 w2271 w2524 w2761 w2983 w3188 w3430 w3467 w3510 w3547 w3585 w3621 w3652 w3707 w3741 w3769 w3947] -> w192
          tunnel: w191 -> [w262 w295 w434 w767 w936 w1170 w1662 w1699 w1738 w1770 w1815 w2001 w2280 w2533 w2779 w2982 w3175 w3429 w3466 w3509 w3546 w3584 w3620 w3651 w3706 w3731 w3775 w3938]
          tunnel: [w262 w295 w435 w767 w936 w1170 w1662 w1699 w1738 w1770 w1815 w2001 w2280 w2533 w2778 w2982 w3176 w3429 w3466 w3509 w3546 w3584 w3620 w3651 w3706 w3731 w3775 w3938] -> w190
          tunnel: w188 -> [_ _ w433 w764 _ w1157 _ _ _ _ w1804 w1990 w2269 w2522 w2760 _ w3174 _ _ _ _ _ _ _ _ _ w3768 w3937]
          tunnel: w187 -> [w240 w303 w432 w762 w939 w1178 w1657 w1694 w1742 w1774 w1826 w2012 w2291 w2544 w2763 w2981 _ w3428 w3465 w3508 w3545 w3583 w3619 w3650 w3705 w3740 _ w3936]
          tunnel: [w229 w303 w432 w762 w939 w1178 w1657 w1694 w1742 w1774 w1823 w2009 w2288 w2541 w2797 w2981 w3177 w3428 w3465 w3508 w3545 w3583 w3619 w3650 w3705 w3740 w3790 w3936] -> w186
          tunnel: [w261 w288 w431 w773 w943 w1179 w1656 w1693 w1735 w1767 w1802 w1988 w2267 w2520 w2788 w2980 w3173 w3427 w3464 w3507 w3544 w3582 w3618 w3648 w3704 w3739 w3782 w3935] -> w178
          tunnel: [w260 w287 w429 w771 w942 w1159 w1655 w1692 w1748 w1781 w1800 w1986 w2265 w2518 w2786 w2979 w3172 w3426 w3463 w3506 w3543 w3581 w3617 w3647 w3703 w3738 w3781 w3934] -> w184
          tunnel: w183 -> [w260 w286 w429 w771 w942 w1159 w1655 w1692 w1748 w1781 w1800 w1986 w2265 w2518 w2785 w2979 w3172 w3426 w3463 w3506 w3543 w3581 w3617 w3647 w3703 w3738 w3781 w3934]
          tunnel: [w259 w285 w428 w770 w941 w1160 w1654 w1691 w1747 w1780 w1799 w1985 w2264 w2517 w2784 w2978 w3171 w3425 w3462 w3505 w3542 w3580 w3616 w3646 w3702 w3737 w3780 w3933] -> w173
          tunnel: w182 -> [w259 w284 w428 w770 w941 w1160 w1654 w1691 w1747 w1780 w1799 w1985 w2264 w2517 w2783 w2978 w3171 w3425 w3462 w3505 w3542 w3580 w3616 w3646 w3702 w3737 w3780 w3933]
          tunnel: w181 -> [_ _ _ _ _ _ _ _ _ _ _ _ _ _ w2800 _ _ _ _ _ _ _ _ _ _ _ _ _]
          tunnel: w180 -> [w258 w283 w427 w774 w931 w1163 w1653 w1690 w1750 w1784 w1798 w1984 w2263 w2516 w2789 w2977 w3170 w3424 w3461 w3504 w3541 w3579 w3615 w3645 w3701 w3736 w3783 w3932]
          tunnel: [w258 w283 w427 w774 w931 w1162 w1653 w1690 w1751 w1785 w1798 w1984 w2263 w2516 w2790 w2977 w3170 w3424 w3461 w3504 w3541 w3579 w3615 w3645 w3701 w3736 w3783 w3932] -> w172
          tunnel: w171 -> [w234 _ _ w758 _ _ _ _ _ _ w1796 w1980 w2261 w2514 _ _ _ _ _ _ _ _ _ _ _ _ w3789 _]
          tunnel: [w234 0 0 w758 0 0 0 0 0 0 w1795 w1982 w2260 w2513 w2757 0 0 0 0 0 0 0 0 0 0 0 w3789 0] -> w164
          tunnel: w170 -> [w235 w278 w424 w759 w921 w1151 w1650 w1687 w1731 w1764 w1792 w1978 w2257 w2510 _ w2963 w3167 w3421 w3457 w3501 w3538 w3576 w3612 w3642 w3698 w3733 w3788 w3929]
          tunnel: [w235 w280 w424 w759 w921 w1151 w1650 w1687 w1731 w1764 w1792 w1978 w2257 w2510 w2757 w2963 w3167 w3421 w3457 w3501 w3538 w3576 w3612 w3642 w3698 w3733 w3788 w3929] -> w169
          tunnel: w168 -> [w236 w279 w423 w760 w920 w1149 w1649 w1686 w1732 w1763 w1793 w1979 w2258 w2511 _ _ w3168 w3420 w3458 w3500 w3537 w3575 w3611 w3641 w3697 w3732 w3787 w3928]
          tunnel: [w236 w279 w423 w760 w920 w1150 w1649 w1686 w1732 w1763 w1793 w1979 w2258 w2511 w2766 FALSE ("OK") w3168 w3420 w3458 w3500 w3537 w3575 w3611 w3641 w3697 w3732 w3787 w3928] -> w167
          tunnel: w166 -> [_ _ _ w741 w908 _ w1648 w1685 _ _ _ _ _ _ _ w2968 _ _ _ _ _ _ _ w3640 _ _ w3761 _]
          tunnel: w165 -> [_ _ _ _ _ _ _ _ _ _ _ _ _ _ _ _ _ w3417 w3454 w3497 w3534 w3572 w3610 _ w3694 w3730 w3764 _]
          tunnel: w163 -> [w232 w275 w420 w765 w928 w1148 w1646 w1683 w1727 w1762 w1790 w1977 w2255 w2509 w2781 w2971 w3165 w3414 w3450 w3494 w3530 w3568 w3605 w3638 w3691 w3725 w3771 w3926]
          tunnel: [w232 w275 w420 w765 w928 w1148 w1646 w1683 w1727 w1762 w1790 w1977 w2255 w2509 w2782 w2971 w3165 w3414 w3450 w3494 w3530 w3568 w3605 w3638 w3691 w3725 w3771 w3926] -> w162
          tunnel: [w233 w276 w421 w766 w929 w1147 w1647 w1684 w1721 w1754 w1791 w1972 w2256 w2508 w2780 w2975 w3166 w3413 w3451 w3495 w3531 w3569 w3606 w3639 w3692 w3726 w3773 w3927] -> w161
          tunnel: [w231 w274 w419 w755 w927 w1144 w1645 w1682 w1730 w1761 w1789 w1976 w2254 w2507 w2770 w2970 w3164 w3412 w3449 w3493 w3529 w3567 w3604 w3637 w3690 w3724 w3786 w3925] -> w159
          tunnel: w158 -> [w231 w274 w419 w755 w927 w1144 w1645 w1682 w1730 w1761 w1789 w1976 w2254 w2507 w2769 w2970 w3164 w3412 w3449 w3493 w3529 w3567 w3604 w3637 w3690 w3724 w3786 w3925]
          tunnel: [w230 w273 w418 w772 w926 w1143 w1643 w1681 w1729 w1760 w1788 w1975 w2253 w2506 w2768 w2969 w3163 w3411 w3448 w3492 w3528 w3566 w3603 w3636 w3689 w3723 w3758 w3921] -> w157
          tunnel: w156 -> [w230 w273 w418 w772 w926 w1143 w1643 w1681 w1729 w1760 w1788 w1975 w2253 w2506 w2767 w2969 w3163 w3411 w3448 w3492 w3528 w3566 w3603 w3636 w3689 w3723 w3758 w3921]
          tunnel: w153 -> [_ _ _ _ _ _ _ _ _ _ w1787 w1974 w2252 w2505 _ _ _ _ _ _ _ _ _ _ _ _ _ _]
          tunnel: w151 -> [_ _ _ _ _ w1142 _ _ w1723 w1752 _ _ _ _ _ _ _ _ _ _ _ _ _ _ _ _ _ _]
          tunnel: w150 -> [_ _ _ w740 _ _ _ _ _ _ _ _ _ _ _ w2966 _ _ _ _ _ _ _ _ _ _ w3757 _]
          tunnel: w149 -> [_ _ _ w739 _ w1140 _ _ _ _ _ _ _ _ _ w2965 _ _ _ _ _ _ _ _ _ _ _ _]
          tunnel: w148 -> [w227 w272 w417 w738 w906 w1141 w1642 w1679 w1725 w1758 w1786 w1973 w2251 w2504 w2759 w2964 w3162 w3409 w3446 w3490 w3526 w3564 w3601 w3634 w3687 w3721 w3754 w3920]
          tunnel: [w227 w272 w417 w738 w907 w1141 w1642 w1679 w1725 w1758 w1786 w1973 w2251 w2504 w2758 w2964 w3162 w3409 w3446 w3490 w3526 w3564 w3601 w3634 w3687 w3721 w3754 w3920] -> w147
          frame "Abort", Default {
            w229 = 0 ("Samps/Chl")
            # "Abort"
            n57 = property on="State" class="Enum (strict)"() -> ("Strings []"=w256:string[])  [unwired: 2 in, 2 out]
            n58 = To Long Integer(number=w255) -> (32bit integer=w254:i32)
            n59 = Number To Decimal String(number=w246) -> (decimal integer string=w244:string)  [unwired: 1 in]
            n60 = To Long Integer(number=w253) -> (32bit integer=w252:i32)
            n61 = Index Array(array=w256, index #1=w254, index #2=w252) -> (element #1=w251:string, element #2=w247:string)
            n62 = Number To Decimal String(number=w242) -> (decimal integer string=w241:string)  [unwired: 1 in]
            n63 = Number To Decimal String(number=w240) -> (decimal integer string=w238:string)  [unwired: 1 in]
            n64 = Concatenate Strings("Last: " ("string"), w251, "; Next: " ("string"), w247, "; Pri: " ("string"), w244, "; Sec: " ("string"), w241, "; Sub: " ("string"), w238) -> (→"Abort Message":string)
          }
          frame "Calculate Resistivity Values" {
            # "Calculate Resistivity Values"
            n65 = case shown="0, Default" w305 {
              selector: w305 -> [w340 _ _]
              tunnel: [w312 0 w399] -> w304
              tunnel: w302 -> [w339 w368 w401]
              tunnel: w301 -> [_ _ _]
              tunnel: w300 -> [w324 w367 w400]
              tunnel: [w324 w367 w395] -> w299
              tunnel: [w339 w368 w396] -> w298
              tunnel: [w339 w367 w397] -> w297
              tunnel: [FALSE ("ErrOut") FALSE ("ErrOut") FALSE ("ErrOut")] -> w289
              tunnel: w277 -> [w338 w352 _]
              tunnel: w288 -> [w332 _ _]
              tunnel: [w322 w391 w403] -> w287
              tunnel: w286 -> [w326 w391 w403]
              tunnel: [w325 w375 w404] -> w285
              tunnel: w284 -> [w325 _ w402]
              tunnel: w276 -> [w319 _ _]
              tunnel: [w308 w353 w394] -> w280
              tunnel: w278 -> [w309 w353 w392]
              tunnel: [w306 w350 w398] -> w271
              tunnel: w270 -> [w306 w350 _]
              frame 0, Default {
                # "0 - Puts together the req'd input params\nand calcs the output R and C params"
                n66 = Unbundle By Name(w338) -> ("4P"=w317:bool, "Frequency"=w335:dbl, "Last Resistor"=w337:T1)
                n67 = Increment(x=w319) -> (x+1=w318:i32)
                n68 = Index Array(array=w332, index (col) #1=0 ("disabled index (col)"), index (col) #2=1 ("index (col)")) -> (element #1=w329:dbl[], element #2=w328:dbl[])  [unwired: 2 in]
                n69 = global read "Global ER2007.vi" "Print Rdata"() -> (w321:bool)
                n70 = Not(x=w317) -> (.not. x?=w316:bool)
                n71 = case shown="\"Resistor 3\"" w337 {
                  tunnel: [0 ("index") 0 ("index") 1 ("index") 2 ("index") 3 ("index") 4 ("index") 5 ("index")] -> w333
                  frame "<none>", Default {
                  }
                  frame "Resistor 1" {
                  }
                  frame "Resistor 2" {
                  }
                  frame "Resistor 3" {
                  }
                  frame "Resistor 4" {
                  }
                  frame "Resistor 5" {
                  }
                  frame "Resistor 6" {
                  }
                }
                n72 = global read "Global ER2007.vi" "Rs Values (Kohms)"() -> (w320:dbl[])
                n73 = Index Array(array=w320, index=w333) -> (element=w334:dbl)
                n74 = Increment(x=w340) -> (x+1=w311:i32)
                n75 = Bundle By Name(cluster=T7 {"Rseries (K)"=0.0, "Frequency (Hz)"=0.0, "Voltages"=[], "Angles"=[]} ("ResistData"), "Rseries (K)"=w334, "Frequency (Hz)"=w335, "Voltages"=w329, "Angles"=w328) -> (w327:T7)
                n76 = call "Calculate Resistivity Parameters.vi"("ResistData"=w327, "Print"=w321, "2P/4P"=w316, "Cell"=w318) -> ("ResistParams"=w323:T2, "ErrOut"=w315:bool)  [unwired: 1 in, 13 out]
                n77 = Or(x="Force Recalc", y=w315) -> (x .or. y?=w307:bool)
                n78 = Select(t=w326, s=w307, f=w323) -> (s? t:f=w322:T2)
                "ResistParams" <- w322
                n79 = case shown="True" w307 {
                  tunnel: w309 -> [_ _]
                  tunnel: [0 2] -> w308
                  frame False {
                  }
                  frame True {
                  }
                }
                n80 = Increment(x=w311) -> (x+1=w310:i32)
                n81 = Select(t=w310, s=w307, f=w311) -> (s? t:f=w312:i32)
              }
              frame 1 {
                w354 = 1000.0  # To Ohms
                w361 = 100.0  # To Meters
                # "ER 1-3"
                # "ER 2-3"
                # "ER 1-4"
                # "ER 1-2"
                # "dist to encap"
                # "Area"
                # "R = p*L/A\np = R*A/L"
                # "ER 1-2\nER 1-3\nER 1-4\nER 2-3"
                # "1 - computes the resistivity values"
                n82 = Unbundle By Name(w352) -> ("Length"=w365:dbl, "Diameter"=w388:dbl, "ElectSpace"=w362:dbl)
                n83 = Unbundle By Name(w391) -> ("R12 (k)"=w383:dbl, "R13 (k)"=w358:dbl, "R2P (k)"=w356:dbl, "R23 (k)"=w377:dbl)
                n84 = Divide(x=w388, y=w361) -> (x/y=w364:dbl)
                n85 = Divide(x=w362, y=w361) -> (x/y=w363:dbl)
                n86 = Multiply(x=w383, y=w354) -> (x*y=w360:dbl)
                n87 = Divide(x=w365, y=w361) -> (x/y=w366:dbl)
                n88 = Multiply(x=w358, y=w354) -> (x*y=w359:dbl)
                n89 = Multiply(x=w364, y=w364) -> (x*y=w387:dbl)
                n90 = Multiply(x=w356, y=w354) -> (x*y=w357:dbl)
                n91 = Subtract(x=w366, y=w363) -> (x-y=w390:dbl)
                n92 = Multiply(x=w387, y=3.141592653589793) -> (x*y=w385:dbl)
                n93 = Multiply(x=w377, y=w354) -> (x*y=w355:dbl)
                n94 = Divide(x=w390, y=2.0) -> (x/y=w374:dbl)
                n95 = Divide(x=w385, y=4.0) -> (x/y=w371:dbl)
                n96 = Add(x=w374, y=w363) -> (x+y=w370:dbl)
                n97 = Multiply(x=w355, y=w371) -> (x*y=w378:dbl)
                n98 = Multiply(x=w357, y=w371) -> (x*y=w380:dbl)
                n99 = Multiply(x=w359, y=w371) -> (x*y=w373:dbl)
                n100 = Multiply(x=w360, y=w371) -> (x*y=w382:dbl)
                n101 = Divide(x=w378, y=w363) -> (x/y=w376:dbl)
                n102 = Divide(x=w380, y=w366) -> (x/y=w379:dbl)
                n103 = Divide(x=w373, y=w370) -> (x/y=w372:dbl)
                n104 = Divide(x=w382, y=w374) -> (x/y=w381:dbl)
                n105 = Build Array(w381, w372, w379, w376) -> (w375:dbl[])
              }
              frame 2 {
                # "Calculate Resistivity error"
                n106 = case shown="0, Default" w392 {
                  selector: w392 -> [w409 w415]
                  tunnel: w402 -> [w410 _]
                  tunnel: [w410 dbl[] [nan, nan, nan, nan]] -> w404
                  tunnel: [w408 w414] -> w398
                  tunnel: [w406 w412] -> w395
                  tunnel: [w407 w413] -> w396
                  tunnel: [T4."Error Handler" ("State") T4."Error Handler" ("State")] -> w397
                  tunnel: [w408 w414] -> w399
                  tunnel: [w409 w415] -> w394
                  tunnel: w401 -> [w407 w413]
                  tunnel: w400 -> [w406 w412]
                  frame 0, Default {
                    w408 = 0
                    # "Must not be the \"bail\" error count"
                  }
                  frame 2.. {
                    w414 = 0
                    # "Last error count - time to bail"
                  }
                }
              }
            }
          }
          frame "Determine Series Resistor" {
            w430 = 20  # Done
            # "Determine Series Resistor"
            n107 = case shown="2" w455 {
              selector: w455 -> [w467 w475 w488 w504 w512 w522 w530 w540 w549 w557 w562 w586 w612 w620 w628 w636 w646 w654 w664 _ w680 w690 w698 w706 w714 w722 _]
              tunnel: [w466 w476 w487 w505 w513 w523 w531 w541 w550 w558 w565 w581 w613 w621 w629 w637 w647 w655 w665 w672 w681 w691 w699 w707 w715 w723 0] -> w453
              tunnel: w452 -> [w465 w474 w482 w503 w511 w521 w529 w539 w548 w556 w566 w585 w611 w619 w627 w635 w645 w653 w663 w671 w679 w689 w697 w705 w713 w721 w734]
              tunnel: w451 -> [_ _ _ _ _ _ _ _ _ _ _ _ _ _ _ _ _ _ _ _ _ _ _ _ _ _ _]
              tunnel: w450 -> [w468 _ _ _ _ _ _ _ _ _ _ w584 _ _ _ _ _ _ _ w670 _ _ _ _ _ _ w733]
              tunnel: [T4."Generator OFF" ("State") T4."Set Auto Mode" ("State") T4."Set Cell Select Relays" ("State") T4."Set Resistor Select Relays" ("State") T4."Set Signal Select Relays" ("State") T4."Wait x Secs" ("State") T4."Generator ON" ("State") T4."Wait x Secs" ("State") T4."Get Vs & Phase" ("State") T4."Get V1g & Phase" ("State") w566 w585 T4."Generator OFF" ("State") T4."Reset Cell Select Relays" ("State") T4."Set Resistor Select Relays" ("State") T4."Set Cell Select Relays" ("State") T4."Wait x Secs" ("State") T4."Generator ON" ("State") T4."Wait x Secs" ("State") w671 T4."Generator OFF" ("State") T4."Wait x Secs" ("State") T4."Reset Cell Select Relays" ("State") T4."Reset Resistor Select Relays" ("State") T4."Reset Signal Select Relays" ("State") T4."Reset Auto Mode" ("State") w735] -> w449
              tunnel: [w465 w474 w482 w503 w511 w521 w529 w539 w548 w556 w566 w585 w611 w619 w627 w635 w645 w653 w663 w671 w679 w689 w697 w705 w713 w721 w734] -> w448
              tunnel: w442 -> [w462 w472 w483 w501 w509 w520 w527 w538 w543 w554 w576 w590 w609 w617 w625 w633 w644 w651 w662 w667 w677 w688 w695 w703 w711 w719 w725]
              tunnel: w441 -> [w463 w473 w486 w502 w510 _ w528 _ w547 w555 w577 w591 w610 w618 w626 w634 _ w652 _ w668 w678 _ w696 w704 w712 w720 w731]
              tunnel: [w463 w473 w486 w502 w510 w517 w528 w535 w547 w555 w577 w591 w610 w618 w626 w634 w641 w652 w659 w668 w678 w685 w696 w704 w712 w720 w731] -> w440
              tunnel: [w462 w472 w484 w501 w509 w520 w527 w538 w543 w554 w576 w587 w609 w617 w625 w633 w644 w651 w662 w667 w677 w688 w695 w703 w711 w719 w725] -> w439
              tunnel: w438 -> [w461 w471 w485 w500 w508 w519 w526 w537 w546 w553 w575 w582 w608 w616 w624 w632 w643 w650 w661 w666 w676 w687 w694 w702 w710 w718 w730]
              tunnel: [w461 w471 w485 w500 w508 w519 w526 w537 w546 w553 w575 w582 w608 w616 w624 w632 w643 w650 w661 w666 w676 w687 w694 w702 w710 w718 w730] -> w437
              tunnel: [w465 w474 w482 w503 w511 w521 w529 w539 w548 w556 w566 w584 w611 w619 w627 w635 w645 w653 w663 w670 w679 w689 w697 w705 w713 w721 w733] -> w436
              tunnel: [w464 w470 w481 w499 T5."Signal 1" ("Signal") w518 w525 w536 w545 w552 w574 w583 w607 w615 w623 w631 w642 w649 w660 w669 w675 w686 w693 w701 w709 w717 w732] -> w435
              tunnel: w434 -> [w464 w470 w481 w499 _ w518 w525 w536 w545 w552 w574 w583 w607 w615 w623 w631 w642 w649 w660 w669 w675 w686 w693 w701 w709 w717 w732]
              tunnel: w433 -> [_ _ _ _ _ w516 _ w534 _ _ _ _ _ _ _ _ w640 _ w658 _ _ w684 _ _ _ _ _]
              tunnel: w431 -> [_ _ _ _ _ _ _ _ _ _ w573 _ _ _ _ _ _ _ _ _ _ _ _ _ _ _ _]
              tunnel: w430 -> [_ _ _ _ _ _ _ _ _ _ w560 w578 _ _ _ _ _ _ _ _ _ _ _ _ _ _ _]
              tunnel: w422 -> [_ _ w480 _ _ _ _ _ _ _ _ _ _ _ _ _ _ _ _ _ _ _ _ _ _ _ _]
              tunnel: w421 -> [_ _ w478 _ _ _ _ _ _ _ _ _ _ _ _ _ _ _ _ _ _ _ _ _ _ _ _]
              frame 0, Default {
                # "0 - Generator OFF"
                n108 = global read "Global ER2007.vi" "GCD Prog"() -> (w457:bool[])
                n109 = Replace Array Subset(array=w457, new element=TRUE ("new element/subarray"), index=2) -> (w456:bool[])
                n110 = global write "Global ER2007.vi" "GCD Prog"(w456) -> ()
                n111 = Increment(x=w467) -> (x+1=w466:i32)
                "Stored State" <- w468
              }
              frame 1 {
                # "1 - Auto Mode ON"
                n112 = Increment(x=w475) -> (x+1=w476:i32)
              }
              frame 2 {
                # "2 - makes sure a resistor is selected\nand then sets the Cell Select Relays"
                n113 = case shown="True" w480 {
                  tunnel: [T1."Resistor 6" ("Last Resistor") w490] -> w479
                  tunnel: w478 -> [_ w491]
                  frame False {
                  }
                  frame True {
                    n114 = case shown="2" w491 {
                      tunnel: [T1."Resistor 3" ("Last Resistor") T1."Resistor 3" ("Last Resistor") T1."<none>" ("Last Resistor") T1."Resistor 2" ("Last Resistor") T1."<none>" ("Last Resistor") T1."Resistor 4" ("Last Resistor")] -> w490
                      frame 0, Default {
                      }
                      frame 1 {
                      }
                      frame 2 {
                      }
                      frame 3 {
                      }
                      frame 4 {
                      }
                      frame 5..7 {
                      }
                    }
                  }
                }
                n115 = Bundle By Name(cluster=w483, "Last Resistor"=w479) -> (w484:T11)
                n116 = Increment(x=w488) -> (x+1=w487:i32)
              }
              frame 3 {
                # "3 - Sets Resistor Select"
                n117 = Increment(x=w504) -> (x+1=w505:i32)
              }
              frame 4 {
                # "4 - Sets Signal Select"
                n118 = Increment(x=w512) -> (x+1=w513:i32)
              }
              frame 5 {
                w515 = 1.0  # 1-sec
                # "5 - small wait"
                n119 = Add(x=w515, y=w516) -> (x+y=w517:dbl)
                n120 = Increment(x=w522) -> (x+1=w523:i32)
              }
              frame 6 {
                # "6 - Generator ON"
                n121 = Increment(x=w530) -> (x+1=w531:i32)
              }
              frame 7 {
                # "7 - small wait"
                n122 = global read "Global ER2007.vi" "GenOnWait"() -> (w532:dbl)
                n123 = Add(x=w532, y=w534) -> (x+y=w535:dbl)
                n124 = Increment(x=w540) -> (x+1=w541:i32)
              }
              frame 8 {
                # "8 - Get generator voltage (Vs).  Note\nthis phase is a loop back one"
                n125 = Unbundle By Name(w543) -> ("Last Resistor"=w542:T1)
                n126 = local write "Last Resistor"(w542) -> ()
                n127 = Increment(x=w549) -> (x+1=w550:i32)
              }
              frame 9 {
                # "9 - Get signal voltage (V1g)"
                n128 = Increment(x=w557) -> (x+1=w558:i32)
              }
              frame 10 {
                w561 = 0.01  # From %
                w570 = 1  # Row
                w572 = 0  # Row
                w571 = 0  # Col
                # "TRUE if V1g above threshold"
                # "10 - Checks to see if value of V1g is in the\nproper range.  If OK, then done; else goes\nto next phase where the next lower resistor\nvalue is set and the process repeated"
                n129 = global read "Global ER2007.vi" "FindRsLoT/H"() -> (w559:dbl)
                n130 = Index Array(array=w573, index (row) #1=w572, index (col) #1=w571, index (row) #2=w570, index (col) #2=w571) -> (element #1=w569:dbl, element #2=w568:dbl)
                n131 = Compound Arithmetic op=MULTIPLY(w561, w559, w569) -> (w567:dbl)
                n132 = Less?(x=w567, y=w568) -> (x < y?=w564:bool)
                n133 = Increment(x=w562) -> (x+1=w563:i32)
                n134 = Select(t=w560, s=w564, f=w563) -> (s? t:f=w565:i32)
              }
              frame 11 {
                # "11 - Test failed, lower resistor value"
                n135 = Unbundle By Name(w590) -> ("Last Resistor"=w589:T1)
                n136 = case shown="\"Resistor 1\"" w589 {
                  tunnel: [T1."Resistor 6" ("Last Resistor") T1."Resistor 1" ("Last Resistor") T1."Resistor 1" ("Last Resistor") T1."Resistor 2" ("Last Resistor") T1."Resistor 3" ("Last Resistor") T1."Resistor 4" ("Last Resistor") T1."Resistor 5" ("Last Resistor")] -> w588
                  tunnel: [w592 w594 w596 w598 w600 w602 w604] -> w579
                  frame "<none>", Default {
                    w592 = FALSE  # Done
                  }
                  frame "Resistor 1" {
                    w594 = TRUE  # Done
                  }
                  frame "Resistor 2" {
                    w596 = FALSE  # Done
                  }
                  frame "Resistor 3" {
                    w598 = FALSE  # Done
                  }
                  frame "Resistor 4" {
                    w600 = FALSE  # Done
                  }
                  frame "Resistor 5" {
                    w602 = FALSE  # Done
                  }
                  frame "Resistor 6" {
                    w604 = FALSE  # Done
                  }
                }
                n137 = Increment(x=w586) -> (x+1=w580:i32)
                n138 = Bundle By Name(cluster=w590, "Last Resistor"=w588) -> (w587:T11)
                n139 = Select(t=w578, s=w579, f=w580) -> (s? t:f=w581:i32)
              }
              frame 12 {
                # "12 - Generator OFF"
                n140 = Increment(x=w612) -> (x+1=w613:i32)
              }
              frame 13 {
                # "13 - Cell Select Relays OFF"
                n141 = Increment(x=w620) -> (x+1=w621:i32)
              }
              frame 14 {
                # "14 - Sets Resistor Select"
                n142 = Increment(x=w628) -> (x+1=w629:i32)
              }
              frame 15 {
                # "15 - Reselect cell"
                n143 = Increment(x=w636) -> (x+1=w637:i32)
              }
              frame 16 {
                w639 = 1.0  # 1-sec
                # "16 - small wait"
                n144 = Add(x=w639, y=w640) -> (x+y=w641:dbl)
                n145 = Increment(x=w646) -> (x+1=w647:i32)
              }
              frame 17 {
                # "17 - Generator ON"
                n146 = Increment(x=w654) -> (x+1=w655:i32)
              }
              frame 18 {
                # "18 - small wait"
                n147 = global read "Global ER2007.vi" "GenOnWait"() -> (w656:dbl)
                n148 = Add(x=w656, y=w658) -> (x+y=w659:dbl)
                n149 = Increment(x=w664) -> (x+1=w665:i32)
              }
              frame 19 {
                w672 = 8  # Repeat @ this phase
                # "19 - Loops back to try again"
              }
              frame 20 {
                # "20 - Done - turn generator OFF"
                n150 = local write "RS Done"(TRUE ("RS Done")) -> ()
                n151 = Increment(x=w680) -> (x+1=w681:i32)
              }
              frame 21 {
                w683 = 1.0  # 1-sec
                # "21 - small wait"
                n152 = Add(x=w683, y=w684) -> (x+y=w685:dbl)
                n153 = Increment(x=w690) -> (x+1=w691:i32)
              }
              frame 22 {
                # "22 - reset cell select relays"
                n154 = Increment(x=w698) -> (x+1=w699:i32)
              }
              frame 23 {
                # "23 - reset resistor select relays"
                n155 = Increment(x=w706) -> (x+1=w707:i32)
              }
              frame 24 {
                # "24 - reset signal select relays"
                n156 = Increment(x=w714) -> (x+1=w715:i32)
              }
              frame 25 {
                # "25 - Auto Mode OFF"
                n157 = Increment(x=w722) -> (x+1=w723:i32)
              }
              frame 26 {
                # "26 - Done, set final values"
                n158 = global read "Global ER2007.vi" "GCD Prog"() -> (w727:bool[])
                n159 = Unbundle By Name(w725) -> ("Last Resistor"=w724:T1)
                n160 = local write "Last Resistor"(w724) -> ()
                n161 = Replace Array Subset(array=w727, new element=FALSE ("new element/subarray"), index=2) -> (w726:bool[])
                n162 = global write "Global ER2007.vi" "GCD Prog"(w726) -> ()
                n163 = local read "Stored State"() -> (w735:T4)
              }
            }
          }
          frame "Done" {
            # "Init GPIB once?"
            # "Done - sets final flags"
            n164 = case shown="0, Default" w775 {
              selector: w775 -> [w782 w801 w814 w827 w841 w853 w873 _]
              tunnel: [w781 w800 w813 w826 w838 w851 w871 0] -> w769
              tunnel: [w776 w796 w810 w823 w836 w852 w872 w897] -> w753
              tunnel: w764 -> [_ _ _ _ _ _ _ _]
              tunnel: [w788 w799 w812 w825 w840 w850 w870 w902] -> w763
              tunnel: w752 -> [w778 w794 w811 w824 w837 w852 w872 _]
              tunnel: w756 -> [w788 w799 w812 w825 w840 w850 w870 w902]
              tunnel: w755 -> [_ _ _ _ _ _ _ w898]
              tunnel: w754 -> [_ _ _ _ _ _ _ w896]
              tunnel: w751 -> [_ w798 w808 w821 w834 _ _ _]
              tunnel: w750 -> [w787 w791 w804 w817 w830 w849 w867 w892]
              tunnel: w749 -> [w786 w790 w803 w816 w829 _ w866 w891]
              tunnel: [w787 w791 w804 w817 w830 w843 w867 w892] -> w748
              tunnel: [w786 w790 w803 w816 w829 errorcluster {"status"=FALSE, "code"=0, "source"=""} ("error IO") w866 w891] -> w747
              tunnel: w746 -> [w785 w793 w806 w819 w832 w847 w869 w894]
              tunnel: w745 -> [w780 w792 w805 w818 w831 w844 w863 w893]
              tunnel: [w780 w792 w805 w818 w831 w844 errorcluster {"status"=FALSE, "code"=0, "source"=""} ("error out") w893] -> w744
              tunnel: [w785 w793 w806 w819 w832 w847 w861 w894] -> w743
              tunnel: w742 -> [_ _ _ _ _ w846 _ _]
              tunnel: w741 -> [_ _ _ _ _ _ w868 _]
              tunnel: w740 -> [_ _ _ _ _ w845 w864 _]
              tunnel: w739 -> [_ _ _ _ _ _ w862 _]
              tunnel: [FALSE FALSE FALSE FALSE FALSE FALSE FALSE FALSE] -> w737
              frame 0, Default {
                # "Agilent error - don't try\nany more Agilent I/O"
                # "0 - Generator OFF; set New Data flag"
                n165 = Unbundle By Name(w780) -> ("status"=w779:bool)
                n166 = global write "Global ER2007.vi" "New Data"(TRUE ("New Data")) -> ()
                n167 = Increment(x=w782) -> (x+1=w781:i32)
                n168 = Select(t=w778, s=w779, f=T4."Generator OFF" ("State")) -> (s? t:f=w776:T4)
              }
              frame 1 {
                # "1 - Reset Cell Select Relays"
                n169 = Unbundle By Name(w798) -> ("status"=w797:bool)
                n170 = Increment(x=w801) -> (x+1=w800:i32)
                n171 = Select(t=w794, s=w797, f=T4."Reset Cell Select Relays" ("State")) -> (s? t:f=w796:T4)
              }
              frame 2 {
                # "2 - Reset Resistor Select Relays"
                n172 = Unbundle By Name(w808) -> ("status"=w807:bool)
                n173 = Increment(x=w814) -> (x+1=w813:i32)
                n174 = Select(t=w811, s=w807, f=T4."Reset Resistor Select Relays" ("State")) -> (s? t:f=w810:T4)
              }
              frame 3 {
                # "3 - Reset Signal Select Relays"
                n175 = Unbundle By Name(w821) -> ("status"=w820:bool)
                n176 = Increment(x=w827) -> (x+1=w826:i32)
                n177 = Select(t=w824, s=w820, f=T4."Reset Signal Select Relays" ("State")) -> (s? t:f=w823:T4)
              }
              frame 4 {
                # "4 - Reset Auto Mode"
                n178 = Unbundle By Name(w834) -> ("status"=w833:bool)
                n179 = global write "Global ER2007.vi" "GCD Reset"(TRUE ("A/D Stop")) -> ()
                n180 = Increment(x=w841) -> (x+1=w838:i32)
                n181 = Select(t=w837, s=w833, f=T4."Reset Auto Mode" ("State")) -> (s? t:f=w836:T4)
              }
              frame 5 {
                # "Phase 5 - delay to let GCD Reset\npropagate; closes NAII session"
                n182 = case shown="False" w845 {
                  tunnel: w849 -> [w856 w859]
                  tunnel: w846 -> [w855 _]
                  tunnel: [refnum<visa-resource-name> refnum ("instrument handle out") w859] -> w843
                  frame False {
                    # "GPIB session is opened & closed each sample"
                    n183 = case shown="False" w855 {
                      tunnel: w856 -> [w858 _]
                      frame False {
                        n184 = VISA Close(VISA resource name=w858) -> ()  [unwired: 1 in, 1 out]
                        n185 = local write "NAII Live"(FALSE ("NAII Live")) -> ()
                      }
                      frame True {
                        # "Sim"
                      }
                    }
                  }
                  frame True {
                    # "Session remains open so long as\nMain program is running.  Close\nis done in Stop"
                  }
                }
                n186 = Increment(x=w853) -> (x+1=w851:i32)
              }
              frame 6 {
                # "Phase 6 - delay to let GCD Reset\npropagate; closes Agilent session.\nIf PC ID=1, passes control to #2;\nno error trapping."
                n187 = case shown="True" w864 {
                  tunnel: w869 -> [w876 w880]
                  tunnel: w868 -> [w875 w879]
                  tunnel: w863 -> [_ w882]
                  tunnel: w862 -> [_ w881]
                  tunnel: [refnum<visa-resource-name> refnum ("dup VISA session") w880] -> w861
                  frame False {
                    # "GPIB session is opened & closed each sample"
                    n188 = case shown="False" w875 {
                      tunnel: w876 -> [w877 _]
                      frame False {
                        n189 = call "ag33xxx - Close.vi"("VISA session"=w877) -> ()  [unwired: 10 in, 1 out]
                        n190 = local write "HP Live"(FALSE ("HP Live")) -> ()
                      }
                      frame True {
                        # "Sim"
                      }
                    }
                  }
                  frame True {
                    # "Session remains open so long as Main program\nis running.  Close is done in Stop"
                    n191 = case shown="1, Default" w881 {
                      tunnel: w882 -> [w884 _]
                      tunnel: w879 -> [w883 _]
                      frame 1, Default {
                        n192 = case shown="False" w883 {
                          tunnel: w884 -> [w888 w889]
                          tunnel: [w885 w889] -> _
                          frame False {
                            # "IF PC #1, PassControl back to 2"
                            n193 = PassControl(2:w888, 3:i16 2 ("address"), 4:0 ("bus")) -> (0:w885:errorcluster)  [unwired: 1 out]
                          }
                          frame True {
                            # "SimHP"
                          }
                        }
                      }
                      frame 2 {
                      }
                    }
                  }
                }
                n194 = Increment(x=w873) -> (x+1=w871:i32)
              }
              frame 7 {
                # "7 - Done, reset busy flag"
                n195 = Get Date/Time In Seconds() -> (seconds since 1Jan1904=w900:timestamp)
                n196 = To Double Precision Float(number=w900) -> (double precision float=w899:dbl)
                n197 = Subtract(x=w899, y=w898) -> (x-y=→"VI Time":dbl)
                n198 = global write "Global ER2007.vi" "GCD Busy"(FALSE ("A/D Stop")) -> ()
                n199 = case shown="False" w896 {
                  tunnel: [T4."Stop" ("State") T4."Idle" ("State")] -> w897
                  frame True {
                  }
                  frame False {
                  }
                }
              }
            }
          }
          frame "Error Handler" {
            # "Error Handler"
            n200 = case shown="0, Default" w925 {
              selector: w925 -> [w954 w1002 w1037 w1069 w1087 _]
              tunnel: [w953 w1001 w1039 w1068 w1086 0] -> w924
              tunnel: w923 -> [w947 w989 _ _ _ _]
              tunnel: w922 -> [w949 w991 w1035 w1066 w1089 w1134]
              tunnel: w921 -> [w945 w987 _ _ _ _]
              tunnel: w920 -> [w946 w996 _ _ _ _]
              tunnel: w919 -> [_ _ _ _ _ _]
              tunnel: [w950 w1003 w1038 w1070 w1095 T4."Done" ("State")] -> w918
              tunnel: w917 -> [w944 w1003 w1036 w1070 w1095 _]
              tunnel: w916 -> [w952 w1000 w1041 _ w1093 w1137]
              tunnel: [w952 w1000 w1040 w1072 w1093 w1137] -> w915
              tunnel: w914 -> [w948 w990 w1043 _ w1094 w1136]
              tunnel: [w948 w990 w1042 w1073 w1094 w1136] -> w913
              tunnel: w912 -> [_ _ _ w1071 _ _]
              tunnel: w911 -> [w951 w998 w1034 w1067 w1090 w1135]
              tunnel: [w951 w998 w1034 w1067 w1092 w1135] -> w910
              tunnel: [w949 w991 w1033 w1066 w1091 w1134] -> w909
              tunnel: w908 -> [_ _ _ _ w1088 _]
              tunnel: [w956 w988 w1032 w1065 w1085 w1133] -> w907
              tunnel: w906 -> [w955 w988 w1032 w1065 w1085 w1133]
              frame 0, Default {
                # "Handles Calculate Resistivity errrors only"
                n201 = case shown="2.." w945 {
                  tunnel: w954 -> [w961 _ _]
                  tunnel: [w960 0 w982] -> w953
                  tunnel: w944 -> [w958 _ _]
                  tunnel: [w958 T4."Initialize" ("State") T4."Final Values" ("State")] -> w950
                  tunnel: w955 -> [w957 w963 _]
                  tunnel: [w957 w963 "   F   "] -> w956
                  tunnel: w947 -> [_ _ w976]
                  tunnel: w949 -> [_ _ w974]
                  tunnel: w948 -> [_ _ w973]
                  tunnel: w946 -> [_ _ w970]
                  frame 0, Default {
                    # "No Calculate Resistivity error"
                    n202 = Add(x=w961, y=1) -> (x+y=w960:i32)
                  }
                  frame 1 {
                    # "One error - try again"
                  }
                  frame 2.. {
                    w967 = TRUE ("element")
                    w979 = -23039  # Parameter Problem
                    w982 = 2  # Continue "Final Values"
                    # "Calc Resistivity\nParameters error"
                    # "Too many errors - write NaN's"
                    n203 = Unbundle By Name(w973) -> ("status"=w971:bool)
                    n204 = Unbundle By Name(w974) -> ("status"=w972:bool)
                    n205 = Unbundle By Name(w976) -> ("status"=w975:bool)
                    n206 = Build Array(w975, w972, w971, w967, w970) -> (w966:bool[])
                    n207 = global write "Global ER2007.vi" "GCD Err"(w967) -> ()
                    n208 = local write "Errs"(w966) -> ()
                    n209 = Bundle By Name(cluster=errorcluster {"status"=FALSE, "code"=0, "source"=""} ("error out"), "status"=TRUE, "code"=w979, "source"="Calculate Resistivity Parameters.vi") -> (w978:errorcluster)
                    n210 = global read "Global ER2007.vi" "LogGcdErrs"() -> (w965:bool)
                    n211 = case shown="True" w965 {
                      tunnel: w978 -> [w983 w984]
                      tunnel: [w983 w985] -> _
                      frame False {
                      }
                      frame True {
                        n212 = call "Write GCD Error Log File.vi"("Error In"=w984) -> ("Error Out"=w985:errorcluster)  [unwired: 7 in, 3 out]
                      }
                    }
                  }
                }
              }
              frame 1 {
                # "1 - Sets error flag"
                n213 = Unbundle By Name(w989) -> ("status"=w995:bool)
                n214 = Unbundle By Name(w991) -> ("status"=w994:bool)
                n215 = Unbundle By Name(w990) -> ("status"=w993:bool)
                n216 = Greater Than 0?(x=w987) -> (x > 0?=w986:bool)
                n217 = Build Array(w995, w994, w993, w986, w996) -> (w1004:bool[])
                "Errs" <- w1004
                n218 = case shown="False" w996 {
                  tunnel: w995 -> [w1011 _]
                  tunnel: w994 -> [w1010 _]
                  tunnel: w993 -> [w1009 _]
                  tunnel: [w1008 w1027] -> w992
                  tunnel: w991 -> [w1007 _]
                  tunnel: w990 -> [w1006 _]
                  tunnel: w989 -> [w1005 w1028]
                  frame False {
                    n219 = case shown="False" w1011 {
                      tunnel: w1010 -> [w1016 _]
                      tunnel: w1009 -> [w1015 _]
                      tunnel: [w1014 w1023] -> w1008
                      tunnel: w1007 -> [w1013 _]
                      tunnel: w1006 -> [w1012 _]
                      tunnel: w1005 -> [_ w1023]
                      frame False {
                        n220 = case shown="False" w1016 {
                          tunnel: w1015 -> [w1019 _]
                          tunnel: [w1018 w1022] -> w1014
                          tunnel: w1013 -> [_ w1022]
                          tunnel: w1012 -> [w1017 _]
                          frame False {
                            n221 = case shown="False" w1019 {
                              tunnel: [errorcluster {"status"=FALSE, "code"=0, "source"=""} ("Error In") w1021] -> w1018
                              tunnel: w1017 -> [_ w1021]
                              frame False {
                                # "No err"
                              }
                              frame True {
                                # "NAII Error"
                              }
                            }
                          }
                          frame True {
                            # "Agilent error"
                          }
                        }
                      }
                      frame True {
                        # "DOUT\nerror"
                      }
                    }
                  }
                  frame True {
                    w1025 = 6  # Generic File Err
                    # "File I/O"
                    n222 = Bundle By Name(cluster=w1028, "status"=TRUE, "code"=w1025, "source"="Write ER2007 Data File.vi") -> (w1027:errorcluster)
                  }
                }
                n223 = Or Array Elements(Boolean array=w1004) -> (logical OR=w999:bool)
                n224 = global write "Global ER2007.vi" "GCD Err"(w999) -> ()
                n225 = global read "Global ER2007.vi" "LogGcdErrs"() -> (w997:bool)
                n226 = Increment(x=w1002) -> (x+1=w1001:i32)
                n227 = case shown="True" w997 {
                  tunnel: w992 -> [w1029 w1030]
                  tunnel: [w1029 w1031] -> _
                  frame False {
                  }
                  frame True {
                    n228 = call "Write GCD Error Log File.vi"("Error In"=w1030) -> ("Error Out"=w1031:errorcluster)  [unwired: 7 in, 3 out]
                  }
                }
              }
              frame 2 {
                # "2 - Checks for NAII & Agilent Errors"
                n229 = case shown="No Error" w1043 {
                  selector: w1043 -> [w1051 _]
                  tunnel: [w1051 errorcluster {"status"=FALSE, "code"=0, "source"=""} ("error IO")] -> w1042
                  tunnel: w1041 -> [w1050 w1059]
                  tunnel: [w1050 refnum<visa-resource-name> refnum ("instrument handle out")] -> w1040
                  tunnel: [w1048 w1060] -> w1039
                  tunnel: [w1047 w1063] -> w1038
                  tunnel: w1037 -> [w1044 w1064]
                  tunnel: w1036 -> [w1046 w1063]
                  tunnel: w1035 -> [w1045 w1058]
                  tunnel: [w1045 w1058] -> w1033
                  frame No Error {
                    n230 = Unbundle By Name(w1045) -> ("status"=w1049:bool)
                    n231 = case shown="True" w1049 {
                      tunnel: [0 w1056] -> w1048
                      tunnel: [T4."Done" ("State") w1057] -> w1047
                      tunnel: w1046 -> [_ w1057]
                      tunnel: w1044 -> [_ w1055]
                      frame False {
                        # "No Agilent Error"
                      }
                      frame True {
                        # "Agilent Error"
                        n232 = Add(x=w1055, y=2) -> (x+y=w1056:i32)
                      }
                    }
                  }
                  frame Error {
                    # "NAII error"
                    n233 = VISA Close(VISA resource name=w1059) -> ()  [unwired: 1 in, 1 out]
                    n234 = Increment(x=w1064) -> (x+1=w1060:i32)
                  }
                }
              }
              frame 3 {
                # "3 - Restarts the NAII"
                n235 = case shown="False" w1071 {
                  tunnel: [w1077 refnum<visa-resource-name> refnum ("instrument handle out")] -> w1072
                  tunnel: [w1075 errorcluster {"status"=FALSE, "code"=0, "source"=""} ("error out")] -> w1073
                  frame False {
                    # "Was NAI2250 Configure.vi"
                    # "Was NAI2250 Initialize.vi"
                    n236 = global read "Global ER2007.vi" "NAI Addr"() -> (w1080:string)
                    n237 = Concatenate Strings("GPIB::" ("string"), w1080, "::INSTR" ("string")) -> (w1079:string)
                    n238 = call "AC2250 Initialize.vi"("VISA Resource Name In"=w1079) -> ("ErrOut"=w1076:errorcluster, "VISA Resource Name Out"=w1078:refnum<visa-resource-name>)  [unwired: 9 in]
                    n239 = call "AC2250 Configure.vi"("ErrIn"=w1076, "Measurement Mode"=T6."TOTAL", "VISA Resource Name In"=w1078) -> ("ErrOut"=w1075:errorcluster, "VISA Resource Name Out"=w1077:refnum<visa-resource-name>)  [unwired: 6 in, 1 out]
                  }
                  frame True {
                    # "Sim"
                  }
                }
                n240 = Increment(x=w1069) -> (x+1=w1068:i32)
              }
              frame 4 {
                # "4 - Tries to re-init Agilent if error"
                n241 = case shown="Error" w1089 {
                  selector: w1089 -> [w1098 w1103]
                  tunnel: [w1099 w1106] -> w1092
                  tunnel: [w1098 w1105] -> w1091
                  tunnel: w1090 -> [w1099 w1104]
                  tunnel: w1088 -> [_ w1102]
                  tunnel: w1087 -> [w1097 w1101]
                  tunnel: [w1096 w1100] -> w1086
                  frame No Error {
                    n242 = Increment(x=w1097) -> (x+1=w1096:i32)
                  }
                  frame Error {
                    n243 = case shown="False" w1102 {
                      tunnel: [w1107 refnum<visa-resource-name> refnum ("dup VISA session")] -> w1106
                      tunnel: [w1108 w1131] -> w1105
                      tunnel: w1103 -> [_ w1131]
                      tunnel: w1104 -> [_ _]
                      frame False {
                        w1117 = TRUE  # Reset (T: Reset)
                        n244 = global read "Global ER2007.vi" "HP Addr"() -> (w1116:string)
                        n245 = Concatenate Strings("GPIB::" ("string"), w1116, "::INSTR" ("string")) -> (w1119:string)
                        n246 = Type Cast(type=refnum<visa-resource-name> "GPIB::10::INSTR" ("Instrument Resource Name"), x=w1119) -> (*(type *) &x=w1118:refnum<visa-resource-name>)
                        n247 = call "ag33xxx - Initialize.vi"("Reset (T: Reset)"=w1117, "Instrument Resource Name"=w1118) -> ("error out"=w1115:errorcluster, "dup VISA session"=w1109:refnum<visa-resource-name>)  [unwired: 8 in]
                        n248 = Unbundle By Name(w1115) -> ("status"=w1111:bool, "code"=w1113:i32)
                        n249 = Equal?(x=w1113, y=-1073807263) -> (x = y?=w1112:bool)
                        n250 = And(x=w1111, y=w1112) -> (x .and. y?=w1110:bool)
                        n251 = case shown="False" w1110 {
                          tunnel: w1115 -> [w1124 _]
                          tunnel: [w1124 w1128] -> w1108
                          tunnel: w1109 -> [w1123 w1125]
                          tunnel: [w1123 w1127] -> w1107
                          frame False {
                          }
                          frame True {
                            n252 = GPIB Status(0:"0:" ("address string"), 1:errorcluster {"status"=FALSE, "code"=0, "source"=""} ("error out")) -> (5:w1126:errorcluster)  [unwired: 3 out]
                            n253 = VISA Clear(VISA resource name=w1125, error in (no error)=w1126) -> (VISA resource name out=w1127:refnum<visa-resource-name>, error out=w1128:errorcluster)
                          }
                        }
                      }
                      frame True {
                        # "Sim"
                      }
                    }
                    n254 = Increment(x=w1101) -> (x+1=w1100:i32)
                  }
                }
              }
              frame 5 {
                # "5 - go to Done"
              }
            }
          }
          frame "Final Values" {
            # "Final Values"
            n255 = case shown="9" w1154 {
              selector: w1154 -> [w1193 w1205 w1216 w1228 w1256 w1268 w1281 w1304 w1315 w1331 w1619 _]
              tunnel: [w1192 w1204 w1215 w1226 w1255 w1266 w1280 w1302 w1314 w1335 w1618 0 ("Samps/Chl")] -> w1155
              tunnel: w1177 -> [w1191 w1200 w1217 w1227 w1257 w1267 w1282 w1303 w1323 w1337 w1617 w1640]
              tunnel: [w1191 T4."Calculate Resistivity Values" ("State") w1217 T4."Get Cell Temperatures" ("State") w1257 T4."Get Cell Pressures" ("State") w1282 w1303 w1323 w1337 w1617 T4."Done" ("State")] -> w1176
              tunnel: [w1191 w1200 w1217 w1227 w1257 w1267 w1282 w1303 w1323 w1337 w1617 w1640] -> w1175
              tunnel: [w1191 w1200 w1217 w1227 w1257 w1267 w1282 w1303 w1323 w1337 w1617 w1640] -> w1174
              tunnel: w1172 -> [_ _ _ _ _ _ _ _ _ _ _ _]
              tunnel: w1171 -> [_ _ _ _ _ _ _ _ _ _ _ _]
              tunnel: w1165 -> [w1190 w1202 w1218 w1225 w1258 w1265 w1283 w1301 w1322 _ _ _]
              tunnel: [w1190 w1202 w1218 w1225 w1258 w1265 w1283 w1301 w1322 w1333 FALSE ("OK") w1637] -> w1164
              tunnel: w1163 -> [w1196 w1206 w1213 w1224 w1250 w1264 w1285 w1310 w1317 w1334 w1620 w1641]
              tunnel: [w1195 w1206 w1214 w1224 w1254 w1264 w1284 w1311 w1317 w1334 w1620 w1641] -> w1162
              tunnel: w1161 -> [w1183 w1203 w1209 w1222 w1240 w1262 w1274 w1299 w1320 w1329 w1616 w1639]
              tunnel: w1160 -> [_ _ w1212 _ w1252 _ _ _ _ _ _ _]
              tunnel: w1159 -> [_ _ _ _ _ _ _ w1309 _ _ _ _]
              tunnel: [FALSE FALSE FALSE FALSE FALSE FALSE FALSE FALSE FALSE FALSE FALSE w1637] -> w1158
              tunnel: w1157 -> [w1184 _ _ _ _ _ _ _ _ _ _ _]
              tunnel: [w1183 w1203 w1209 w1222 w1240 w1262 w1276 w1299 w1319 w1328 w1616 w1639] -> w1156
              tunnel: [w1182 w1199 w1208 w1221 w1234 w1261 w1277 w1298 w1313 w1333 w1615 w1638] -> w1150
              tunnel: w1149 -> [w1182 w1199 w1208 w1221 w1234 w1261 w1277 w1298 w1313 _ w1615 w1638]
              tunnel: w1147 -> [_ _ _ _ _ _ w1271 _ _ w1326 w1621 _]
              tunnel: w1146 -> [w1181 w1198 w1207 w1220 w1233 w1260 w1273 w1297 w1312 w1332 w1612 w1635]
              tunnel: [w1181 w1198 w1207 w1220 w1233 w1260 w1273 w1297 w1312 w1332 w1612 w1635] -> w1145
              tunnel: w1143 -> [_ _ _ _ _ _ _ _ _ w1330 _ _]
              tunnel: w1142 -> [_ _ _ _ _ _ w1272 _ _ w1325 _ _]
              tunnel: w1141 -> [_ _ _ _ _ _ _ _ _ w1327 _ _]
              tunnel: w1140 -> [_ _ _ _ _ _ _ _ _ w1324 _ _]
              frame 0, Default {
                w1187 = 3600.0  # Secs to Hrs
                w1194 = 0  # Col 1
                # "0 - stores Elapsed Time"
                n256 = Unbundle By Name(w1183) -> ("Start Time"=w1189:dbl)
                n257 = Subtract(x=w1184, y=w1189) -> (x-y=w1188:dbl)
                n258 = Divide(x=w1188, y=w1187) -> (x/y=w1186:dbl)
                n259 = global write "Global ER2007.vi" "GCD Prog"(bool[] [FALSE, FALSE, FALSE, TRUE, FALSE, FALSE] ("GCD Prog")) -> ()
                n260 = Replace Array Subset(array=w1196, new element=w1186, index=w1194) -> (w1195:dbl[])
                n261 = Increment(x=w1193) -> (x+1=w1192:i32)
              }
              frame 1 {
                # "1 - calculates resistivity results"
                n262 = Increment(x=w1205) -> (x+1=w1204:i32)
              }
              frame 2 {
                w1211 = 1  # ER's
                # "2 - stores the four resistivity values"
                n263 = Replace Array Subset(array=w1213, new element=w1212, index=w1211) -> (w1214:dbl[])
                n264 = Increment(x=w1216) -> (x+1=w1215:i32)
              }
              frame 3 {
                # "3 - Get Cell Temperatures ( inserted into\nthe Final Data automatically by subroutine)"
                n265 = Increment(x=w1228) -> (x+1=w1226:i32)
              }
              frame 4 {
                w1230 = 2  # 2P=ER 1-4
                w1246 = 21.5 ("y")
                w1231 = 3  # 4P=ER 2-3
                w1253 = 5  # F 2-3
                # "Denominator"
                # "Numerator"
                # "T- A"
                # "F 2-3 = (ER 2-3)/[ {Rw * (RwTemp + 21.5)}/{T-A + 21.5} ]"
                # "4 - Calculates & stores the\nformation factor F 2-3"
                n266 = Unbundle By Name(w1240) -> ("4P"=w1232:bool, "Rw"=w1239:dbl, "Rw Temp"=w1248:dbl)
                n267 = Select(t=w1231, s=w1232, f=w1230) -> (s? t:f=w1229:i32)
                n268 = Index Array(array=w1250, index=7) -> (element=w1247:dbl)
                n269 = Index Array(array=w1252, index=w1229) -> (element=w1251:dbl)
                n270 = Add(x=w1248, y=w1246) -> (x+y=w1244:dbl)
                n271 = Add(x=w1247, y=w1246) -> (x+y=w1245:dbl)
                n272 = Divide(x=w1244, y=w1245) -> (x/y=w1243:dbl)
                n273 = Multiply(x=w1243, y=w1239) -> (x*y=w1242:dbl)
                n274 = Not Equal To 0?(x=w1239) -> (x != 0?=w1238:bool)
                n275 = Divide(x=w1251, y=w1242) -> (x/y=w1237:dbl)
                n276 = Select(t=w1237, s=w1238, f=0.0) -> (s? t:f=w1236:dbl)
                n277 = Replace Array Subset(array=w1250, new element=w1236, index=w1253) -> (w1254:dbl[])
                n278 = Increment(x=w1256) -> (x+1=w1255:i32)
              }
              frame 5 {
                # "5 - Get Cell Pressures ( inserted into\nthe Final Data automatically by subroutine)"
                n279 = Increment(x=w1268) -> (x+1=w1266:i32)
              }
              frame 6 {
                w1279 = 12  # Pore Vol
                # "6 - Stuffs latest Pore Volume"
                n280 = Increment(x=w1271) -> (x+1=w1270:i32)
                n281 = Index Array(array=w1272, index=w1270) -> (element=w1269:bool)
                n282 = case shown="False" w1269 {
                  tunnel: w1271 -> [w1289 _]
                  tunnel: [w1286 w1295] -> w1275
                  tunnel: w1274 -> [_ w1296]
                  frame False {
                    n283 = case shown="4" w1289 {
                      tunnel: [w1290 w1291 w1292 w1293 w1294] -> w1287
                      frame 0, Default {
                        w1290 = 36  # Pvol1
                      }
                      frame 1 {
                        w1291 = 38  # Pvol2
                      }
                      frame 2 {
                        w1292 = 40  # Pvol3
                      }
                      frame 3 {
                        w1293 = 42  # Pvol4
                      }
                      frame 4 {
                        w1294 = 44  # Pvol5
                      }
                    }
                    n284 = global read "Global ER2007.vi" "A/D EUs"() -> (w1288:dbl[])
                    n285 = Index Array(array=w1288, index=w1287) -> (element=w1286:dbl)
                  }
                  frame True {
                    # "No Galil"
                    n286 = Unbundle By Name(w1296) -> ("Last Pore Vol"=w1295:dbl)
                  }
                }
                n287 = Bundle By Name(cluster=w1274, "Last Pore Vol"=w1275) -> (w1276:T11)
                n288 = Replace Array Subset(array=w1285, new element=w1275, index=w1279) -> (w1284:dbl[])
                n289 = Increment(x=w1281) -> (x+1=w1280:i32)
              }
              frame 7 {
                w1305 = 13  # C14 & C23
                # "New Data File Format-Data Line\n\n                        Reals\nCol #  Process Variable Col #\n----- ----------------- -----\n  1   Point Flag\n  2   Point Date\n  3   Point Time\n  4   Elapsed Time (hrs)  1\n  5   ER 1-2              2\n  6   ER 1-3              3\n  7   ER 1-4              4\n  8   ER 2-3              5\n  9   F 2-3               6\n 10   T-A                 7\n 11   T-B                 8\n 12   NOP                 9\n 13   Pc                 10\n 14   Delta-P            11\n 15   Pc-d               12\n 16   Displaced Vol      13\n 17   C14                14\n 18   C23                15\n 19   Comment"
                # "7 - adds C14 and C23 to final data"
                n290 = Unbundle By Name(w1309) -> ("C2P (pf)"=w1307:dbl, "C23 (pf)"=w1308:dbl)
                n291 = Build Array(w1307, w1308) -> (w1306:dbl[])
                n292 = Replace Array Subset(array=w1310, new element=w1306, index=w1305) -> (w1311:dbl[])
                n293 = Increment(x=w1304) -> (x+1=w1302:i32)
              }
              frame 8 {
                # "8 - Stuff in Cell cluster"
                n294 = Unbundle By Name(w1320) -> ("CurData"=w1318:dbl[][])
                n295 = Build Array (concatenate)(w1318, w1317) -> (w1316:dbl[][])
                n296 = Bundle By Name(cluster=w1320, "CurData"=w1316) -> (w1319:T11)
                n297 = Increment(x=w1315) -> (x+1=w1314:i32)
              }
              frame 9 {
                # "9 - Write the data to file"
                n298 = stacked-sequence {
                  seq-local: [w1345 _ _ _] -> [_ w1357 w1555 w1575]
                  seq-local: [w1344 _ _ _] -> [_ _ _ w1578]
                  seq-local: [_ w1356 _ _] -> [_ _ _ w1577]
                  seq-local: [w1341 _ _ _] -> [_ w1355 _ w1576]
                  seq-local: [w1340 _ _ _] -> [_ _ _ w1573]
                  seq-local: [w1339 _ _ _] -> [_ _ _ w1572]
                  seq-local: [_ _ w1551 _] -> [_ _ _ w1568]
                  tunnel: [_ _ _ w1570] -> w1335
                  tunnel: w1334 -> [_ _ w1552 _]
                  tunnel: [_ _ _ w1574] -> w1333
                  tunnel: w1331 -> [_ _ _ w1571]
                  tunnel: w1330 -> [_ _ _ w1569]
                  tunnel: w1329 -> [w1338 w1351 w1554 w1566]
                  tunnel: [_ _ w1553 _] -> w1328
                  tunnel: w1327 -> [_ _ _ w1567]
                  tunnel: w1326 -> [_ w1354 _ _]
                  tunnel: w1325 -> [_ w1353 _ _]
                  tunnel: w1324 -> [_ w1352 _ _]
                  frame #0 {
                    w1342 = TRUE  # Auto Append
                    # "TRUE if file open error"
                    # "TRUE if cell is not active"
                    # "Force error"
                    # "TRUE if error or cell not active"
                    # "TRUE if file is new"
                    # "Checks to see if the file already exists"
                    n299 = Unbundle By Name(w1338) -> ("Datafile"=w1348:path, "Cell Status"=w1343:enum16{"Inactive", "Setup", "Active", "Done"})
                    n300 = case shown="\"Active\"" w1343 {
                      tunnel: [TRUE FALSE] -> w1340
                      frame "Inactive", Default {
                      }
                      frame "Active" {
                      }
                    }
                    n301 = Strip Path(path=w1348) -> (stripped path=w1347:path, name=w1346:string)
                    n302 = call "File Open Logic.vi"("PathIn"=w1347, "Filename"=w1346, "Auto Append"=w1342) -> ("FullPathOut"=w1344:path, "NewOut"=w1345:bool, "ErrOut"=w1339:bool)  [unwired: 11 in, 3 out]
                    n303 = Or(x=w1339, y=w1340) -> (x .or. y?=w1341:bool)
                  }
                  frame #1 {
                    # "Does Header if req'd"
                    n304 = case shown="False" w1355 {
                      tunnel: w1357 -> [w1363 _]
                      tunnel: w1351 -> [w1362 _]
                      tunnel: [w1361 string[] []] -> w1356
                      tunnel: w1354 -> [w1360 _]
                      tunnel: w1353 -> [w1359 _]
                      tunnel: w1352 -> [w1358 _]
                      frame False {
                        # "No error so far"
                        n305 = case shown="True" w1363 {
                          tunnel: w1362 -> [_ w1371]
                          tunnel: [string[] [] w1370] -> w1361
                          tunnel: w1360 -> [_ w1368]
                          tunnel: w1359 -> [_ w1367]
                          tunnel: w1358 -> [_ w1365]
                          frame False {
                            # "File already exists - no header"
                          }
                          frame True {
                            w1369 = "\t"  # Tab
                            # "File is new - do header"
                            n306 = Increment(x=w1368) -> (x+1=w1366:i32)
                            n307 = Initialize Array("") -> (w1373:string[])  [unwired: 1 in]
                            n308 = for {
                              N: 19 -> [_]
                              shift-right: [w1380] -> w1370
                              shift-left: w1373 -> [w1379]
                              tunnel: w1371 -> [w1381]
                              tunnel: w1369 -> [w1378]
                              tunnel: w1366 -> [w1377]
                              tunnel: w1367 -> [w1376]
                              tunnel: w1365 -> [w1375]
                              i -> [w1382]
                              n309 = case shown="17" w1382 {
                                tunnel: w1381 -> [_ _ w1398 w1405 w1412 w1419 w1426 w1435 w1444 w1453 w1462 w1472 w1485 w1494 w1503 w1512 w1522 _ _]
                                tunnel: [w1388 w1394 w1402 w1409 w1416 w1423 w1430 w1439 w1448 w1457 w1466 w1476 w1489 w1498 w1507 w1516 w1525 w1533 w1548] -> w1380
                                tunnel: w1379 -> [w1387 w1393 w1401 w1408 w1415 w1422 w1429 w1438 w1447 w1456 w1465 w1475 w1488 w1497 w1506 w1515 w1524 w1534 w1549]
                                tunnel: w1378 -> [w1383 w1389 w1395 w1403 w1410 w1417 w1424 w1431 w1440 w1449 w1458 w1467 w1481 w1490 w1499 w1508 w1517 w1531 w1546]
                                tunnel: w1377 -> [_ _ _ _ _ _ _ _ _ _ _ _ _ _ _ _ _ w1528 w1543]
                                tunnel: w1376 -> [_ _ _ _ _ _ _ _ _ _ _ _ _ _ _ _ _ _ w1544]
                                tunnel: w1375 -> [_ _ _ _ _ _ _ _ _ _ _ _ _ _ _ _ _ w1529 _]
                                frame 0, Default {
                                # "Date"
                                n310 = Get Date/Time String() -> (date string=w1384:string)  [unwired: 3 in, 1 out]
                                n311 = Concatenate Strings("Date: " ("string"), w1383, w1384) -> (w1385:string)
                                n312 = Build Array (concatenate)(w1387, w1385) -> (w1388:string[])
                                }
                                frame 1 {
                                # "Time"
                                n313 = Get Date/Time String() -> (time string=w1390:string)  [unwired: 3 in, 1 out]
                                n314 = Concatenate Strings("Time: " ("string"), w1389, w1390) -> (w1391:string)
                                n315 = Build Array (concatenate)(w1393, w1391) -> (w1394:string[])
                                }
                                frame 2 {
                                # "Filename"
                                n316 = Unbundle By Name(w1398) -> ("Datafile"=w1397:path)
                                n317 = Path To String(path=w1397) -> (string=w1396:string)
                                n318 = Concatenate Strings("Filename: " ("string"), w1395, w1396) -> (w1399:string)
                                n319 = Build Array (concatenate)(w1401, w1399) -> (w1402:string[])
                                }
                                frame 3 {
                                # "Project"
                                n320 = Unbundle By Name(w1405) -> ("Project"=w1404:string)
                                n321 = Concatenate Strings("Project: " ("string"), w1403, w1404) -> (w1406:string)
                                n322 = Build Array (concatenate)(w1408, w1406) -> (w1409:string[])
                                }
                                frame 4 {
                                # "Sample ID"
                                n323 = Unbundle By Name(w1412) -> ("Sample #"=w1411:string)
                                n324 = Concatenate Strings("Sample ID: " ("string"), w1410, w1411) -> (w1413:string)
                                n325 = Build Array (concatenate)(w1415, w1413) -> (w1416:string[])
                                }
                                frame 5 {
                                # "Rock Type"
                                n326 = Unbundle By Name(w1419) -> ("Rock Type"=w1418:string)
                                n327 = Concatenate Strings("Rock Type: " ("string"), w1417, w1418) -> (w1420:string)
                                n328 = Build Array (concatenate)(w1422, w1420) -> (w1423:string[])
                                }
                                frame 6 {
                                # "Fluid Pair"
                                n329 = Unbundle By Name(w1426) -> ("Fluid Pair"=w1425:string)
                                n330 = Concatenate Strings("Fluid Pair: " ("string"), w1424, w1425) -> (w1427:string)
                                n331 = Build Array (concatenate)(w1429, w1427) -> (w1430:string[])
                                }
                                frame 7 {
                                # "RW"
                                n332 = Unbundle By Name(w1435) -> ("Rw"=w1434:dbl)
                                n333 = Number To Fractional String(number=w1434, precision (6)=i16 3) -> (F-format string=w1432:string)  [unwired: 2 in]
                                n334 = Concatenate Strings("RW: " ("string"), w1431, w1432) -> (w1436:string)
                                n335 = Build Array (concatenate)(w1438, w1436) -> (w1439:string[])
                                }
                                frame 8 {
                                # "RW Temp"
                                n336 = Unbundle By Name(w1444) -> ("Rw Temp"=w1443:dbl)
                                n337 = Number To Fractional String(number=w1443, precision (6)=i16 1) -> (F-format string=w1441:string)  [unwired: 2 in]
                                n338 = Concatenate Strings("RW Temp: " ("string"), w1440, w1441) -> (w1445:string)
                                n339 = Build Array (concatenate)(w1447, w1445) -> (w1448:string[])
                                }
                                frame 9 {
                                # "Frequency"
                                n340 = Unbundle By Name(w1453) -> ("Frequency"=w1452:dbl)
                                n341 = Number To Fractional String(number=w1452, precision (6)=i16 0) -> (F-format string=w1450:string)  [unwired: 2 in]
                                n342 = Concatenate Strings("Frequency: " ("string"), w1449, w1450) -> (w1454:string)
                                n343 = Build Array (concatenate)(w1456, w1454) -> (w1457:string[])
                                }
                                frame 10 {
                                # "Amplitude"
                                n344 = Unbundle By Name(w1462) -> ("Amplitude"=w1461:dbl)
                                n345 = Number To Fractional String(number=w1461, precision (6)=i16 0) -> (F-format string=w1459:string)  [unwired: 2 in]
                                n346 = Concatenate Strings("Amplitude: " ("string"), w1458, w1459) -> (w1463:string)
                                n347 = Build Array (concatenate)(w1465, w1463) -> (w1466:string[])
                                }
                                frame 11 {
                                # "DAQ Period"
                                n348 = Unbundle By Name(w1472) -> ("DAQ Period"=w1469:u32, "DAQ Units"=w1470:u16)
                                n349 = case shown="1" w1470 {
                                tunnel: w1469 -> [w1477 w1480]
                                tunnel: [w1477 w1479] -> w1468
                                frame 0, Default {
                                }
                                frame 1 {
                                # "Hours"
                                n350 = Multiply(x=w1480, y=u32 60) -> (x*y=w1479:u32)
                                }
                                }
                                n351 = Number To Decimal String(number=w1468) -> (decimal integer string=w1471:string)  [unwired: 1 in]
                                n352 = Concatenate Strings("DAQ Period (mins): " ("string"), w1467, w1471) -> (w1473:string)
                                n353 = Build Array (concatenate)(w1475, w1473) -> (w1476:string[])
                                }
                                frame 12 {
                                # "Length"
                                n354 = Unbundle By Name(w1485) -> ("Length"=w1484:dbl)
                                n355 = Number To Fractional String(number=w1484, precision (6)=i16 4) -> (F-format string=w1482:string)  [unwired: 2 in]
                                n356 = Concatenate Strings("Length: " ("string"), w1481, w1482) -> (w1486:string)
                                n357 = Build Array (concatenate)(w1488, w1486) -> (w1489:string[])
                                }
                                frame 13 {
                                # "Diameter"
                                n358 = Unbundle By Name(w1494) -> ("Diameter"=w1493:dbl)
                                n359 = Number To Fractional String(number=w1493, precision (6)=i16 4) -> (F-format string=w1491:string)  [unwired: 2 in]
                                n360 = Concatenate Strings("Diameter: " ("string"), w1490, w1491) -> (w1495:string)
                                n361 = Build Array (concatenate)(w1497, w1495) -> (w1498:string[])
                                }
                                frame 14 {
                                # "Porosity"
                                n362 = Unbundle By Name(w1503) -> ("Porosity"=w1502:dbl)
                                n363 = Number To Fractional String(number=w1502, precision (6)=i16 2) -> (F-format string=w1500:string)  [unwired: 2 in]
                                n364 = Concatenate Strings("Porosity: " ("string"), w1499, w1500) -> (w1504:string)
                                n365 = Build Array (concatenate)(w1506, w1504) -> (w1507:string[])
                                }
                                frame 15 {
                                # "Permeability"
                                n366 = Unbundle By Name(w1512) -> ("Permeability"=w1511:dbl)
                                n367 = Number To Fractional String(number=w1511, precision (6)=i16 2) -> (F-format string=w1509:string)  [unwired: 2 in]
                                n368 = Concatenate Strings("Permeability: " ("string"), w1508, w1509) -> (w1513:string)
                                n369 = Build Array (concatenate)(w1515, w1513) -> (w1516:string[])
                                }
                                frame 16 {
                                # "Spacing"
                                n370 = Unbundle By Name(w1522) -> ("ElectSpace"=w1521:dbl)
                                n371 = Number To Fractional String(number=w1521, precision (6)=i16 2) -> (F-format string=w1519:string)  [unwired: 2 in]
                                n372 = Concatenate Strings("Elect Spacing: " ("string"), w1517, w1519) -> (w1518:string)
                                n373 = Build Array (concatenate)(w1524, w1518) -> (w1525:string[])
                                }
                                frame 17 {
                                # "Cell #"
                                n374 = case shown="2" w1529 {
                                tunnel: w1528 -> [w1535 w1538]
                                tunnel: [w1535 w1537] -> w1527
                                frame 1, Default {
                                }
                                frame 2 {
                                n375 = Add(x=w1538, y=5) -> (x+y=w1537:i32)
                                }
                                }
                                n376 = Number To Decimal String(number=w1527) -> (decimal integer string=w1526:string)  [unwired: 1 in]
                                n377 = Concatenate Strings("Cell No: " ("string"), w1531, w1526) -> (w1530:string)
                                n378 = Build Array (concatenate)(w1534, w1530) -> (w1533:string[])
                                }
                                frame 18 {
                                # "Galil mode"
                                n379 = Index Array(array=w1544, index=w1543) -> (element=w1542:bool)
                                n380 = Select(t="Manual", s=w1542, f="VPA") -> (s? t:f=w1539:string)
                                n381 = Concatenate Strings("Prod Vol Meas: " ("string"), w1546, w1539) -> (w1545:string)
                                n382 = Build Array (concatenate)(w1549, w1545) -> (w1548:string[])
                                }
                              }
                            }
                          }
                        }
                      }
                      frame True {
                        # "Previous error or inactive cell"
                      }
                    }
                  }
                  frame #2 {
                    # "Fixes start and elapsed times if new"
                    n383 = case shown="True" w1555 {
                      tunnel: w1554 -> [w1557 w1565]
                      tunnel: [w1557 w1564] -> w1553
                      tunnel: w1552 -> [w1556 w1561]
                      tunnel: [w1556 w1558] -> w1551
                      frame False {
                        # "File is not new"
                      }
                      frame True {
                        w1560 = 0  # Col 1
                        # "New file - redo start\nand elapsed times"
                        n384 = Get Date/Time In Seconds() -> (seconds since 1Jan1904=w1563:timestamp)
                        n385 = Replace Array Subset(array=w1561, new element=0.0, index=w1560) -> (w1558:dbl[])
                        n386 = To Double Precision Float(number=w1563) -> (double precision float=w1562:dbl)
                        n387 = Bundle By Name(cluster=w1565, "Start Time"=w1562) -> (w1564:T11)
                      }
                    }
                  }
                  frame #3 {
                    # "Writes the file"
                    n388 = case shown="False" w1576 {
                      tunnel: w1578 -> [w1596 _]
                      tunnel: w1577 -> [w1593 _]
                      tunnel: w1568 -> [w1592 _]
                      tunnel: w1575 -> [w1591 _]
                      tunnel: [w1587 w1611] -> w1574
                      tunnel: w1573 -> [_ w1610]
                      tunnel: w1572 -> [_ w1609]
                      tunnel: w1569 -> [w1581 _]
                      tunnel: w1567 -> [w1579 _]
                      tunnel: w1566 -> [w1585 _]
                      frame False {
                        w1583 = "   F   "  # ResCalcFail
                        # "No errors"
                        n389 = Strip Path(path=w1596) -> (stripped path=w1595:path, name=w1594:string)
                        n390 = Unbundle By Name(w1585) -> ("Comment"=w1584:string)
                        n391 = Equal?(x=w1579, y=w1583) -> (x = y?=w1582:bool)
                        n392 = global read "Global ER2007.vi" "No File"() -> (w1586:bool)
                        n393 = Select(t=enum16{"Do Nothing", "Header", "Data"}."Header" ("Function"), s=w1591, f=enum16{"Do Nothing", "Header", "Data"}."Data" ("Function")) -> (s? t:f=w1588:enum16{"Do Nothing", "Header", "Data"})
                        n394 = Or(x=w1581, y=w1582) -> (x .or. y?=w1580:bool)
                        n395 = case shown="False" w1586 {
                          tunnel: w1595 -> [w1606 _]
                          tunnel: w1594 -> [w1605 _]
                          tunnel: w1593 -> [w1604 _]
                          tunnel: w1592 -> [w1603 _]
                          tunnel: w1588 -> [w1602 _]
                          tunnel: [w1600 FALSE ("OK")] -> w1587
                          tunnel: w1580 -> [w1599 _]
                          tunnel: w1579 -> [w1598 _]
                          tunnel: w1584 -> [w1597 _]
                          frame False {
                            n396 = call "Write ER2007 Data File.vi"("PathIn"=w1606, "Filename"=w1605, "Header"=w1604, "DataIn"=w1603, "Comment"=w1597, "Function"=w1602, "Mark Line"=w1599, "Mark String"=w1598) -> ("OK"=w1601:bool)  [unwired: 10 in, 1 out]
                            n397 = Not(x=w1601) -> (.not. x?=w1600:bool)
                          }
                          frame True {
                          }
                        }
                      }
                      frame True {
                        # "TRUE if cell is active and a file open error"
                        # "Previous error or\ninactive cell"
                        n398 = Not(x=w1610) -> (.not. x?=w1608:bool)
                        n399 = And(x=w1608, y=w1609) -> (x .and. y?=w1611:bool)
                      }
                    }
                    n400 = Increment(x=w1571) -> (x+1=w1570:i32)
                  }
                }
              }
              frame 10 {
                # "10 - Updates the Cell data"
                n401 = stacked-sequence {
                  tunnel: w1616 -> [w1623 _ _]
                  tunnel: w1621 -> [w1626 _ _]
                  frame #0 {
                    # "Updates the TestInfo cluster; clears Comment"
                    n402 = global read "Global ER2007.vi" "Test Info"() -> (w1628:T3)
                    n403 = Increment(x=w1626) -> (x+1=w1625:i32)
                    n404 = Bundle By Name(cluster=w1623, "Comment"="") -> (w1622:T11)
                    n405 = global write "Global ER2007.vi" "GCDStatusCell"(w1625) -> ()
                    n406 = Unbundle By Name(w1628) -> ("Cell Data"=w1631:T12)
                    n407 = Replace Array Subset(array=w1631, new element=w1622, index=w1626) -> (w1630:T12)
                    n408 = Bundle By Name(cluster=w1628, "Cell Data"=w1630) -> (w1627:T3)
                    "Test Info Out" <- w1627
                    n409 = global write "Global ER2007.vi" "Test Info"(w1627) -> ()
                    n410 = local write "Errs"(bool[] [FALSE, FALSE, FALSE, FALSE, FALSE] ("Errs")) -> ()
                  }
                  frame #1 {
                    n411 = Wait (ms)(milliseconds to wait=u32 1000) -> ()  [unwired: 1 out]
                  }
                  frame #2 {
                    n412 = global write "Global ER2007.vi" "New GCD Status"(TRUE ("New GCD Status")) -> ()
                  }
                }
                n413 = Increment(x=w1619) -> (x+1=w1618:i32)
              }
              frame 11 {
                w1637 = FALSE ("OK")
                # "11 - go to Done"
              }
            }
          }
          frame "Generator OFF" {
            # "Turns Generator OFF"
            n414 = case shown="False" w1648 {
              tunnel: w1661 -> [w1676 w1677]
              tunnel: w1660 -> [w1675 w1678]
              tunnel: [w1674 w1678] -> w1659
              tunnel: [w1672 w1677] -> w1658
              frame False {
                w1673 = FALSE  # OFF
                n415 = call "ag33xxx - Output Enabled.vi"("error in (no error)"=w1676, "Output Enabled? (T: Yes)"=w1673, "VISA session"=w1675) -> ("error out"=w1672:errorcluster, "dup VISA session"=w1674:refnum<visa-resource-name>)  [unwired: 7 in]
              }
              frame True {
                # "Sim"
              }
            }
            n416 = Unbundle By Name(w1658) -> ("status"=w1644:bool)
          }
          frame "Generator ON" {
            # "Turns Generator ON"
            n417 = case shown="False" w1685 {
              tunnel: w1698 -> [w1713 w1714]
              tunnel: w1697 -> [w1712 w1715]
              tunnel: [w1711 w1715] -> w1696
              tunnel: [w1709 w1714] -> w1695
              frame False {
                w1710 = TRUE  # ON
                n418 = call "ag33xxx - Output Enabled.vi"("error in (no error)"=w1713, "Output Enabled? (T: Yes)"=w1710, "VISA session"=w1712) -> ("error out"=w1709:errorcluster, "dup VISA session"=w1711:refnum<visa-resource-name>)  [unwired: 7 in]
              }
              frame True {
                # "Sim"
              }
            }
            n419 = Unbundle By Name(w1695) -> ("status"=w1680:bool)
          }
          frame "Get Cell Pressures" {
            w1749 = 8  # Conf & Pore & Pdp & Pdn
            # "Get Cell Pressures"
            n420 = global read "Global ER2007.vi" "A/D EUs"() -> (w1722:dbl[])
            n421 = call "Get Cell Pressures and Temperatures.vi"("EUs"=w1722, "Cell #"=w1721, "Cell x Data"=w1720, "No Galil"=w1723) -> ("NOP"=w1719:dbl, "Pc"=w1718:dbl, "Delta-P"=w1717:dbl, "DwnStrm-P"=w1716:dbl)  [unwired: 10 in, 2 out]
            n422 = Build Array(w1719, w1718, w1717, w1716) -> (w1724:dbl[])
            n423 = Replace Array Subset(array=w1750, new element=w1724, index=w1749) -> (w1751:dbl[])
          }
          frame "Get Cell Temperatures" {
            w1782 = 6  # Two Temperatures
            # "Get Cell Temperatures"
            n424 = global read "Global ER2007.vi" "A/D EUs"() -> (w1757:dbl[])
            n425 = call "Get Cell Pressures and Temperatures.vi"("EUs"=w1757, "Cell #"=w1754, "Cell x Data"=w1753, "No Galil"=w1752) -> ("T-A"=w1756:dbl, "T-B"=w1755:dbl)  [unwired: 10 in, 4 out]
            n426 = Build Array(w1756, w1755) -> (w1783:dbl[])
            n427 = Replace Array Subset(array=w1784, new element=w1783, index=w1782) -> (w1785:dbl[])
          }
          frame "Get Vs & Phase" {
            # "Get Vs and Phase"
            n428 = case shown="0, Default" w1826 {
              selector: w1826 -> [w1846 w1866 w1883 w1935]
              tunnel: [w1844 w1867 w1882 w1934] -> w1823
              tunnel: [w1843 w1861 w1881 w1933] -> w1822
              tunnel: [w1845 w1860 w1887 w1931] -> w1821
              tunnel: w1820 -> [w1843 w1861 w1881 w1929]
              tunnel: w1819 -> [w1845 w1860 w1887 w1930]
              tunnel: [w1843 w1861 w1881 w1932] -> w1818
              tunnel: w1817 -> [_ _ _ _]
              tunnel: w1813 -> [w1841 w1868 w1899 w1928]
              tunnel: w1812 -> [w1842 w1869 w1900 w1921]
              tunnel: [w1839 w1868 w1898 w1928] -> w1811
              tunnel: [w1840 w1869 w1884 w1925] -> w1810
              tunnel: w1808 -> [w1838 w1870 w1878 w1926]
              tunnel: [w1838 w1870 w1878 w1926] -> w1807
              tunnel: [w1837 w1863 w1894 w1927] -> w1806
              tunnel: w1805 -> [_ w1863 w1894 w1927]
              tunnel: w1804 -> [w1836 w1864 _ _]
              tunnel: w1803 -> [w1835 w1859 w1885 w1937]
              tunnel: [w1835 w1859 w1891 w1937] -> w1802
              tunnel: w1801 -> [w1834 _ w1886 _]
              tunnel: w1796 -> [w1831 w1858 w1880 w1922]
              tunnel: [w1831 w1858 w1880 w1923] -> w1795
              tunnel: [FALSE FALSE w1875 w1920] -> w1794
              tunnel: w1790 -> [_ _ w1879 _]
              tunnel: w1787 -> [w1829 _ _ _]
              frame 0, Default {
                # "0 - Requests Reference voltage"
                n429 = case shown="False" w1834 {
                  tunnel: w1842 -> [w1850 w1855]
                  tunnel: w1841 -> [w1849 w1856]
                  tunnel: [w1853 w1855] -> w1840
                  tunnel: [w1852 w1856] -> w1839
                  frame False {
                    w1854 = TRUE  # Ref
                    n430 = call "AC2250 Measurement Mode.vi"("ErrIn"=w1850, "Measurement Mode"=T6."TOTAL", "VISA Resource Name In"=w1849) -> ("ErrOut"=w1847:errorcluster, "VISA Resource Name Out"=w1848:refnum<visa-resource-name>)  [unwired: 6 in, 1 out]
                    n431 = call "AC2250 Measurement Channel.vi"("ErrIn"=w1847, "Reference"=w1854, "VISA Resource Name In"=w1848) -> ("ErrOut"=w1853:errorcluster, "VISA Resource Name Out"=w1852:refnum<visa-resource-name>)  [unwired: 6 in, 1 out]
                  }
                  frame True {
                    # "Sim"
                  }
                }
                n432 = Multiply(x=1.0, y=w1829) -> (x*y=w1830:dbl)
                n433 = Increment(x=w1846) -> (x+1=w1844:i32)
                n434 = Add(x=w1830, y=w1836) -> (x+y=w1837:dbl)
              }
              frame 1 {
                # "1 - Waits awhile"
                n435 = Greater Or Equal?(x=w1864, y=w1863) -> (x >= y?=w1862:bool)
                n436 = Increment(x=w1866) -> (x+1=w1865:i32)
                n437 = Select(t=w1865, s=w1862, f=w1866) -> (s? t:f=w1867:i32)
              }
              frame 2 {
                w1888 = 0.0  # Phase
                w1893 = 1.41421  # To peak V
                w1871 = TRUE  # Vs check enabled = T
                w1890 = 0  # Row
                w1889 = 1  # Col
                w1896 = 0  # Row
                w1897 = 0  # Col
                # "2 - Gets reference voltage and saves it"
                n438 = case shown="False" w1886 {
                  tunnel: w1900 -> [w1903 w1918]
                  tunnel: w1899 -> [w1905 w1919]
                  tunnel: [w1904 w1919] -> w1898
                  tunnel: [w1902 w1918] -> w1884
                  tunnel: [w1901 w1910] -> w1873
                  tunnel: w1879 -> [_ w1913]
                  frame False {
                    n439 = call "AC2250 Measure (Main).vi"("ErrIn"=w1903, "VISA Resource Name In"=w1905) -> ("ErrOut"=w1902:errorcluster, "Value"=w1901:dbl, "VISA Resource Name Out"=w1904:refnum<visa-resource-name>)  [unwired: 5 in, 2 out]
                  }
                  frame True {
                    w1906 = 0.0  # NoNoise
                    w1914 = 1.41421  # From peak V
                    w1917 = 0  # Row
                    w1916 = 0  # Col
                    # "Sim"
                    n440 = Index Array(array=w1913, index (row)=w1917, index (col)=w1916) -> (element=w1915:dbl)
                    n441 = Random Number (0-1)() -> (number: 0 to 1=w1912:dbl)
                    n442 = Divide(x=w1915, y=w1914) -> (x/y=w1909:dbl)
                    n443 = Subtract(x=w1912, y=0.5) -> (x-y=w1908:dbl)
                    n444 = Multiply(x=w1908, y=0.01) -> ()  [unwired: 1 out]
                    n445 = Add(x=w1906, y=w1909) -> (x+y=w1910:dbl)
                  }
                }
                n446 = Unbundle By Name(w1878) -> ("Amplitude"=w1877:dbl)
                n447 = Multiply(x=w1893, y=w1873) -> (x*y=w1895:dbl)
                n448 = Divide(x=w1877, y=2.0) -> (x/y=w1874:dbl)
                n449 = Replace Array Subset(array=w1885, new element=w1895, index (row)=w1896, index (col)=w1897) -> (w1892:dbl[][])
                n450 = Less?(x=w1873, y=w1874) -> (x < y?=w1872:bool)
                n451 = Replace Array Subset(array=w1892, new element=w1888, index (row)=w1890, index (col)=w1889) -> (w1891:dbl[][])
                n452 = Increment(x=w1883) -> (x+1=w1882:i32)
                n453 = And(x=w1872, y=w1871) -> (x .and. y?=w1875:bool)
              }
              frame 3 {
                # "3 - Checks for errors and repeats as req'd"
                n454 = Unbundle By Name(w1921) -> ("status"=w1936:bool, "code"=w1924:i32)
                n455 = case shown="True" w1936 {
                  tunnel: w1935 -> [_ _]
                  tunnel: [0 ("Samps/Chl") w1952] -> w1934
                  tunnel: [w1943 w1950] -> w1933
                  tunnel: [w1941 w1949] -> w1932
                  tunnel: [w1943 w1948] -> w1931
                  tunnel: w1930 -> [w1943 w1947]
                  tunnel: w1929 -> [w1941 w1951]
                  tunnel: [errorcluster {"status"=FALSE, "code"=0, "source"=""} ("error out") w1953] -> w1925
                  tunnel: w1924 -> [_ w1958]
                  tunnel: [0 w1954] -> w1923
                  tunnel: w1922 -> [_ w1946]
                  tunnel: w1921 -> [_ w1945]
                  tunnel: [FALSE w1944] -> w1920
                  frame False {
                    # "No error - done"
                  }
                  frame True {
                    w1956 = 3  # Max Tries
                    w1957 = -1074118636  # Out-of-lock freq cond.
                    # "Error - is error a T/O"
                    n456 = Greater Or Equal?(x=w1946, y=w1956) -> (x >= y?=w1955:bool)
                    n457 = Equal?(x=w1957, y=w1958) -> ()  [unwired: 1 out]
                    n458 = case shown="False" w1955 {
                      tunnel: [w1960 0] -> w1954
                      tunnel: [errorcluster {"status"=FALSE, "code"=0, "source"=""} ("error out") w1966] -> w1953
                      tunnel: [0 ("Samps/Chl") 0 ("Samps/Chl")] -> w1952
                      tunnel: w1951 -> [w1963 w1968]
                      tunnel: [w1963 w1968] -> w1950
                      tunnel: [w1963 w1968] -> w1949
                      tunnel: [w1962 w1967] -> w1948
                      tunnel: w1947 -> [w1962 w1967]
                      tunnel: w1946 -> [w1961 _]
                      tunnel: w1945 -> [_ w1966]
                      tunnel: [FALSE TRUE] -> w1944
                      frame False {
                        # "Clears error and tries againg"
                        n459 = Increment(x=w1961) -> (x+1=w1960:i32)
                      }
                      frame True {
                        # "Time to give up - too many errors"
                      }
                    }
                  }
                }
              }
            }
            n460 = Or(x=w1794, y=w1827) -> (x .or. y?=w1828:bool)
          }
          frame "Get V1g & Phase" {
            # "Get V1g and Phase"
            n461 = case shown="2" w2012 {
              selector: w2012 -> [w2030 w2050 w2072 w2136 w2156 _ _]
              tunnel: [w2028 w2051 w2071 w2134 w2157 0 ("Samps/Chl") w2216] -> w2009
              tunnel: [w2027 w2045 w2070 w2133 w2151 w2167 w2214] -> w2008
              tunnel: [w2029 w2044 w2069 w2135 w2150 w2167 w2212] -> w2007
              tunnel: w2006 -> [w2027 w2045 w2070 w2133 w2151 w2180 w2211]
              tunnel: w2005 -> [w2029 w2044 w2069 w2135 w2150 w2167 w2210]
              tunnel: [w2027 w2045 w2070 w2133 w2151 w2180 w2213] -> w2004
              tunnel: w2003 -> [_ _ _ _ _ _ _]
              tunnel: w1999 -> [w2019 w2052 w2075 w2125 w2158 w2171 w2208]
              tunnel: w1998 -> [w2022 w2053 w2076 w2128 w2159 w2173 w2201]
              tunnel: [w2020 w2052 w2074 w2127 w2158 w2170 w2208] -> w1997
              tunnel: [w2021 w2053 w2073 w2126 w2159 w2172 w2209] -> w1996
              tunnel: w1994 -> [w2026 w2054 w2056 w2132 w2160 w2175 w2204]
              tunnel: [w2026 w2054 w2056 w2132 w2160 w2175 w2204] -> w1993
              tunnel: [w2025 w2047 w2065 w2131 w2153 w2176 w2205] -> w1992
              tunnel: w1991 -> [_ w2047 w2065 _ w2153 w2176 w2205]
              tunnel: w1990 -> [w2024 w2048 _ w2130 w2154 _ _]
              tunnel: w1989 -> [w2023 w2043 w2060 w2129 w2149 w2165 w2215]
              tunnel: [w2023 w2043 w2063 w2129 w2149 w2174 w2215] -> w1988
              tunnel: w1974 -> [w2015 _ _ w2121 _ _ _]
              tunnel: w1987 -> [w2018 _ w2061 w2124 _ w2166 _]
              tunnel: [w2017 w2042 w2059 w2123 w2148 w2163 w2207] -> w1982
              tunnel: [FALSE FALSE FALSE FALSE FALSE FALSE w2206] -> w1981
              tunnel: w1980 -> [w2017 w2042 w2059 w2123 w2148 w2163 w2200]
              tunnel: w1977 -> [_ _ w2057 _ _ w2161 _]
              tunnel: w1972 -> [_ _ w2055 _ _ _ _]
              frame 0, Default {
                # "0 - Requests Signal voltage"
                n462 = case shown="False" w2018 {
                  tunnel: w2022 -> [w2033 w2039]
                  tunnel: [w2037 w2039] -> w2021
                  tunnel: [w2038 w2040] -> w2020
                  tunnel: w2019 -> [w2034 w2040]
                  frame False {
                    w2036 = FALSE  # Ref
                    n463 = call "AC2250 Measurement Mode.vi"("ErrIn"=w2033, "Measurement Mode"=T6."TOTAL", "VISA Resource Name In"=w2034) -> ("ErrOut"=w2031:errorcluster, "VISA Resource Name Out"=w2032:refnum<visa-resource-name>)  [unwired: 6 in, 1 out]
                    n464 = call "AC2250 Measurement Channel.vi"("ErrIn"=w2031, "Reference"=w2036, "VISA Resource Name In"=w2032) -> ("ErrOut"=w2037:errorcluster, "VISA Resource Name Out"=w2038:refnum<visa-resource-name>)  [unwired: 6 in, 1 out]
                  }
                  frame True {
                    # "Sim"
                  }
                }
                n465 = Increment(x=w2030) -> (x+1=w2028:i32)
                n466 = Add(x=w2015, y=w2024) -> (x+y=w2025:dbl)
              }
              frame 1 {
                # "1 - Waits awhile"
                n467 = Greater Or Equal?(x=w2048, y=w2047) -> (x >= y?=w2046:bool)
                n468 = Increment(x=w2050) -> (x+1=w2049:i32)
                n469 = Select(t=w2049, s=w2046, f=w2050) -> (s? t:f=w2051:i32)
              }
              frame 2 {
                w2064 = 1.41421  # To peak V
                w2067 = 1  # Row
                w2068 = 0  # Col
                # "2 - Gets signal voltage and saves it"
                n470 = case shown="False" w2061 {
                  tunnel: w2076 -> [w2080 w2095]
                  tunnel: w2075 -> [w2081 w2096]
                  tunnel: [w2078 w2096] -> w2074
                  tunnel: [w2077 w2095] -> w2073
                  tunnel: [w2079 w2089] -> w2062
                  tunnel: w2057 -> [_ w2094]
                  tunnel: w2056 -> [_ w2086]
                  tunnel: w2055 -> [_ w2087]
                  frame False {
                    n471 = call "AC2250 Measure (Main).vi"("ErrIn"=w2080, "VISA Resource Name In"=w2081) -> ("ErrOut"=w2077:errorcluster, "Value"=w2079:dbl, "VISA Resource Name Out"=w2078:refnum<visa-resource-name>)  [unwired: 5 in, 2 out]
                  }
                  frame True {
                    w2088 = 0.0  # NoNoise
                    w2097 = 1.41421  # From peak V
                    w2100 = 1  # Row
                    w2099 = 0  # Col
                    # "Sim"
                    n472 = case shown="3" w2087 {
                      tunnel: w2086 -> [w2104 w2108 w2112 w2116 w2120]
                      tunnel: [w2101 w2105 w2109 w2113 w2117] -> w2082
                      frame 0, Default {
                        # "Cell 1 Sim"
                        n473 = Unbundle By Name(w2104) -> ("Last Resistor"=w2102:T1)
                        n474 = Equal?(x=T1."Resistor 3" ("Last Resistor"), y=w2102) -> (x = y?=w2101:bool)
                      }
                      frame 1 {
                        # "Cell 2 Sim"
                        n475 = Unbundle By Name(w2108) -> ("Last Resistor"=w2106:T1)
                        n476 = Equal?(x=T1."Resistor 3" ("Last Resistor"), y=w2106) -> (x = y?=w2105:bool)
                      }
                      frame 2 {
                        # "Cell 3 Sim"
                        n477 = Unbundle By Name(w2112) -> ("Last Resistor"=w2110:T1)
                        n478 = Equal?(x=T1."Resistor 1" ("Last Resistor"), y=w2110) -> (x = y?=w2109:bool)
                      }
                      frame 3 {
                        # "Cell 4 Sim"
                        n479 = Unbundle By Name(w2116) -> ("Last Resistor"=w2114:T1)
                        n480 = Equal?(x=T1."Resistor 2" ("Last Resistor"), y=w2114) -> (x = y?=w2113:bool)
                      }
                      frame 4 {
                        # "Cell 5 Sim"
                        n481 = Unbundle By Name(w2120) -> ("Last Resistor"=w2118:T1)
                        n482 = Equal?(x=T1."Resistor 1" ("Last Resistor"), y=w2118) -> (x = y?=w2117:bool)
                      }
                    }
                    n483 = Index Array(array=w2094, index (row)=w2100, index (col)=w2099) -> (element=w2098:dbl)
                    n484 = Random Number (0-1)() -> (number: 0 to 1=w2093:dbl)
                    n485 = Divide(x=w2098, y=w2097) -> (x/y=w2085:dbl)
                    n486 = Subtract(x=w2093, y=0.5) -> (x-y=w2091:dbl)
                    n487 = Multiply(x=w2091, y=0.01) -> ()  [unwired: 1 out]
                    n488 = Select(t=w2085, s=w2082, f=0.75) -> (s? t:f=w2084:dbl)
                    n489 = Add(x=w2088, y=w2084) -> (x+y=w2089:dbl)
                  }
                }
                n490 = Multiply(x=w2064, y=w2062) -> (x*y=w2066:dbl)
                n491 = Replace Array Subset(array=w2060, new element=w2066, index (row)=w2067, index (col)=w2068) -> (w2063:dbl[][])
                n492 = Increment(x=w2072) -> (x+1=w2071:i32)
              }
              frame 3 {
                # "3 - Requests Signal phase angle"
                n493 = case shown="False" w2124 {
                  tunnel: w2128 -> [w2139 w2145]
                  tunnel: [w2142 w2146] -> w2127
                  tunnel: [w2144 w2145] -> w2126
                  tunnel: w2125 -> [w2140 w2146]
                  frame False {
                    w2143 = FALSE  # Ref
                    n494 = call "AC2250 Measurement Mode.vi"("ErrIn"=w2139, "Measurement Mode"=T6."PHASE ANGLE", "VISA Resource Name In"=w2140) -> ("ErrOut"=w2137:errorcluster, "VISA Resource Name Out"=w2138:refnum<visa-resource-name>)  [unwired: 6 in, 1 out]
                    n495 = call "AC2250 Measurement Channel.vi"("ErrIn"=w2137, "Reference"=w2143, "VISA Resource Name In"=w2138) -> ("ErrOut"=w2144:errorcluster, "VISA Resource Name Out"=w2142:refnum<visa-resource-name>)  [unwired: 6 in, 1 out]
                  }
                  frame True {
                    # "Sim"
                  }
                }
                n496 = Increment(x=w2136) -> (x+1=w2134:i32)
                n497 = Add(x=w2121, y=w2130) -> (x+y=w2131:dbl)
              }
              frame 4 {
                # "4 - Waits awhile"
                n498 = Greater Or Equal?(x=w2154, y=w2153) -> (x >= y?=w2152:bool)
                n499 = Increment(x=w2156) -> (x+1=w2155:i32)
                n500 = Select(t=w2155, s=w2152, f=w2156) -> (s? t:f=w2157:i32)
              }
              frame 5 {
                w2169 = 360.0  # Minus
                w2178 = 1  # Row
                w2179 = 1  # Col
                # "5 - Gets phase angle and saves it"
                n501 = case shown="False" w2166 {
                  tunnel: w2173 -> [w2184 w2195]
                  tunnel: [w2181 w2195] -> w2172
                  tunnel: w2171 -> [w2185 w2194]
                  tunnel: [w2183 w2194] -> w2170
                  tunnel: [w2182 w2192] -> w2164
                  tunnel: w2161 -> [_ w2193]
                  frame False {
                    n502 = call "AC2250 Measure (Main).vi"("ErrIn"=w2184, "VISA Resource Name In"=w2185) -> ("ErrOut"=w2181:errorcluster, "Value"=w2182:dbl, "VISA Resource Name Out"=w2183:refnum<visa-resource-name>)  [unwired: 5 in, 2 out]
                  }
                  frame True {
                    w2186 = 0.0  # NoNoise
                    w2196 = 360.0  # Plus
                    w2199 = 1  # Row
                    w2198 = 1  # Col
                    # "Sim"
                    n503 = Index Array(array=w2193, index (row)=w2199, index (col)=w2198) -> (element=w2197:dbl)
                    n504 = Random Number (0-1)() -> (number: 0 to 1=w2187:dbl)
                    n505 = Add(x=w2197, y=w2196) -> (x+y=w2191:dbl)
                    n506 = Subtract(x=w2187, y=0.5) -> (x-y=w2189:dbl)
                    n507 = Multiply(x=w2189, y=0.01) -> ()  [unwired: 1 out]
                    n508 = Add(x=w2186, y=w2191) -> (x+y=w2192:dbl)
                  }
                }
                n509 = Subtract(x=w2164, y=w2169) -> (x-y=w2177:dbl)
                n510 = Replace Array Subset(array=w2165, new element=w2177, index (row)=w2178, index (col)=w2179) -> (w2174:dbl[][])
              }
              frame 6 {
                # "6 - Checks for errors and repeats as req'd"
                n511 = Unbundle By Name(w2201) -> ("status"=w2203:bool, "code"=w2202:i32)
                n512 = case shown="True" w2203 {
                  tunnel: [0 ("Samps/Chl") w2231] -> w2216
                  tunnel: [w2222 w2229] -> w2214
                  tunnel: [w2220 w2228] -> w2213
                  tunnel: [w2222 w2227] -> w2212
                  tunnel: w2210 -> [w2222 w2226]
                  tunnel: w2211 -> [w2220 w2230]
                  tunnel: [errorcluster {"status"=FALSE, "code"=0, "source"=""} ("error out") w2232] -> w2209
                  tunnel: w2202 -> [_ w2237]
                  tunnel: [0 w2233] -> w2207
                  tunnel: w2200 -> [_ w2225]
                  tunnel: w2201 -> [_ w2224]
                  tunnel: [FALSE w2223] -> w2206
                  frame False {
                    # "No error - done"
                  }
                  frame True {
                    w2235 = 3  # Max Tries
                    w2236 = -1074118636  # Out-of-lock freq cond.
                    # "Error - is error a T/O"
                    n513 = Greater Or Equal?(x=w2225, y=w2235) -> (x >= y?=w2234:bool)
                    n514 = Equal?(x=w2236, y=w2237) -> ()  [unwired: 1 out]
                    n515 = case shown="True" w2234 {
                      tunnel: [w2239 w2245] -> w2233
                      tunnel: [errorcluster {"status"=FALSE, "code"=0, "source"=""} ("error out") w2246] -> w2232
                      tunnel: [0 ("Samps/Chl") 0 ("Samps/Chl")] -> w2231
                      tunnel: w2230 -> [w2242 w2248]
                      tunnel: [w2242 w2248] -> w2229
                      tunnel: [w2242 w2248] -> w2228
                      tunnel: [w2241 w2247] -> w2227
                      tunnel: w2226 -> [w2241 w2247]
                      tunnel: w2225 -> [w2240 w2245]
                      tunnel: w2224 -> [_ w2246]
                      tunnel: [FALSE TRUE] -> w2223
                      frame False {
                        # "Clears error and tries againg"
                        n516 = Increment(x=w2240) -> (x+1=w2239:i32)
                      }
                      frame True {
                        # "Time to give up - too many errors"
                      }
                    }
                  }
                }
              }
            }
            n517 = Or(x=w1981, y=w2013) -> (x .or. y?=w2014:bool)
          }
          frame "Get V2g & Phase" {
            # "Get V2g and Phase"
            n518 = case shown="5" w2291 {
              selector: w2291 -> [w2309 w2329 w2350 w2389 w2409 _ _]
              tunnel: [w2307 w2330 w2349 w2387 w2410 0 ("Samps/Chl") w2466] -> w2288
              tunnel: [w2306 w2324 w2348 w2386 w2404 w2420 w2465] -> w2287
              tunnel: [w2308 w2323 w2347 w2388 w2403 w2420 w2463] -> w2286
              tunnel: w2285 -> [w2306 w2324 w2348 w2386 w2404 w2433 w2462]
              tunnel: w2284 -> [w2308 w2323 w2347 w2388 w2403 w2420 w2461]
              tunnel: [w2306 w2324 w2348 w2386 w2404 w2433 w2464] -> w2283
              tunnel: w2282 -> [_ _ _ _ _ _ _]
              tunnel: w2278 -> [w2298 w2331 w2353 w2377 w2411 w2424 w2468]
              tunnel: w2277 -> [w2301 w2332 w2354 w2381 w2412 w2426 w2455]
              tunnel: [w2299 w2331 w2352 w2380 w2411 w2423 w2468] -> w2276
              tunnel: [w2300 w2332 w2351 w2379 w2412 w2425 w2469] -> w2275
              tunnel: w2273 -> [w2305 w2333 w2342 w2385 w2413 w2428 w2460]
              tunnel: [w2305 w2333 w2342 w2385 w2413 w2428 w2460] -> w2272
              tunnel: [w2304 w2326 w2343 w2384 w2406 w2429 w2459] -> w2271
              tunnel: w2270 -> [_ w2326 w2343 _ w2406 w2429 w2459]
              tunnel: w2269 -> [w2303 w2327 _ w2383 w2407 _ _]
              tunnel: w2268 -> [w2302 w2322 w2339 w2382 w2402 w2418 w2467]
              tunnel: [w2302 w2322 w2340 w2382 w2402 w2427 w2467] -> w2267
              tunnel: w2252 -> [w2294 _ _ w2374 _ _ _]
              tunnel: w2266 -> [w2297 _ w2338 w2378 _ w2419 _]
              tunnel: w2261 -> [w2296 w2321 w2336 w2376 w2401 w2416 w2458]
              tunnel: [w2296 w2321 w2336 w2376 w2401 w2416 w2457] -> w2260
              tunnel: [FALSE FALSE FALSE FALSE FALSE FALSE w2456] -> w2259
              tunnel: w2255 -> [_ _ w2334 _ _ w2414 _]
              frame 0, Default {
                # "0 - Requests Signal voltage"
                n519 = case shown="False" w2297 {
                  tunnel: w2301 -> [w2312 w2318]
                  tunnel: [w2316 w2318] -> w2300
                  tunnel: [w2317 w2319] -> w2299
                  tunnel: w2298 -> [w2313 w2319]
                  frame False {
                    w2315 = FALSE  # Ref
                    n520 = call "AC2250 Measurement Mode.vi"("ErrIn"=w2312, "Measurement Mode"=T6."TOTAL", "VISA Resource Name In"=w2313) -> ("ErrOut"=w2310:errorcluster, "VISA Resource Name Out"=w2311:refnum<visa-resource-name>)  [unwired: 6 in, 1 out]
                    n521 = call "AC2250 Measurement Channel.vi"("ErrIn"=w2310, "Reference"=w2315, "VISA Resource Name In"=w2311) -> ("ErrOut"=w2316:errorcluster, "VISA Resource Name Out"=w2317:refnum<visa-resource-name>)  [unwired: 6 in, 1 out]
                  }
                  frame True {
                    # "Sim"
                  }
                }
                n522 = Increment(x=w2309) -> (x+1=w2307:i32)
                n523 = Add(x=w2294, y=w2303) -> (x+y=w2304:dbl)
              }
              frame 1 {
                # "1 - Waits awhile"
                n524 = Greater Or Equal?(x=w2327, y=w2326) -> (x >= y?=w2325:bool)
                n525 = Increment(x=w2329) -> (x+1=w2328:i32)
                n526 = Select(t=w2328, s=w2325, f=w2329) -> (s? t:f=w2330:i32)
              }
              frame 2 {
                w2341 = 1.41421  # To peak V
                w2345 = 2  # Row
                w2346 = 0  # Col
                # "2 - Gets signal voltage and saves it"
                n527 = case shown="False" w2338 {
                  tunnel: w2354 -> [w2357 w2369]
                  tunnel: w2353 -> [w2359 w2362]
                  tunnel: [w2358 w2362] -> w2352
                  tunnel: [w2355 w2369] -> w2351
                  tunnel: [w2356 w2367] -> w2337
                  tunnel: w2334 -> [_ w2368]
                  frame False {
                    n528 = call "AC2250 Measure (Main).vi"("ErrIn"=w2357, "VISA Resource Name In"=w2359) -> ("ErrOut"=w2355:errorcluster, "Value"=w2356:dbl, "VISA Resource Name Out"=w2358:refnum<visa-resource-name>)  [unwired: 5 in, 2 out]
                  }
                  frame True {
                    w2360 = 0.0  # NoNoise
                    w2370 = 1.41421  # From peak V
                    w2373 = 2  # Row
                    w2372 = 0  # Col
                    # "Sim"
                    n529 = Index Array(array=w2368, index (row)=w2373, index (col)=w2372) -> (element=w2371:dbl)
                    n530 = Random Number (0-1)() -> (number: 0 to 1=w2363:dbl)
                    n531 = Divide(x=w2371, y=w2370) -> (x/y=w2361:dbl)
                    n532 = Subtract(x=w2363, y=0.5) -> (x-y=w2365:dbl)
                    n533 = Multiply(x=w2365, y=0.01) -> ()  [unwired: 1 out]
                    n534 = Add(x=w2360, y=w2361) -> (x+y=w2367:dbl)
                  }
                }
                n535 = Multiply(x=w2341, y=w2337) -> (x*y=w2344:dbl)
                n536 = Replace Array Subset(array=w2339, new element=w2344, index (row)=w2345, index (col)=w2346) -> (w2340:dbl[][])
                n537 = Increment(x=w2350) -> (x+1=w2349:i32)
              }
              frame 3 {
                # "3 - Requests Signal phase angle"
                n538 = case shown="False" w2378 {
                  tunnel: w2381 -> [w2395 w2398]
                  tunnel: [w2394 w2399] -> w2380
                  tunnel: [w2393 w2398] -> w2379
                  tunnel: w2377 -> [w2396 w2399]
                  frame False {
                    w2390 = FALSE  # Ref
                    n539 = call "AC2250 Measurement Mode.vi"("ErrIn"=w2395, "Measurement Mode"=T6."PHASE ANGLE", "VISA Resource Name In"=w2396) -> ("ErrOut"=w2391:errorcluster, "VISA Resource Name Out"=w2392:refnum<visa-resource-name>)  [unwired: 6 in, 1 out]
                    n540 = call "AC2250 Measurement Channel.vi"("ErrIn"=w2391, "Reference"=w2390, "VISA Resource Name In"=w2392) -> ("ErrOut"=w2393:errorcluster, "VISA Resource Name Out"=w2394:refnum<visa-resource-name>)  [unwired: 6 in, 1 out]
                  }
                  frame True {
                    # "Sim"
                  }
                }
                n541 = Increment(x=w2389) -> (x+1=w2387:i32)
                n542 = Add(x=w2374, y=w2383) -> (x+y=w2384:dbl)
              }
              frame 4 {
                # "4 - Waits awhile"
                n543 = Greater Or Equal?(x=w2407, y=w2406) -> (x >= y?=w2405:bool)
                n544 = Increment(x=w2409) -> (x+1=w2408:i32)
                n545 = Select(t=w2408, s=w2405, f=w2409) -> (s? t:f=w2410:i32)
              }
              frame 5 {
                w2422 = 360.0  # Minus
                w2431 = 2  # Row
                w2432 = 1  # Col
                # "5 - Gets phase angle and saves it"
                n546 = case shown="False" w2419 {
                  tunnel: w2426 -> [w2437 w2448]
                  tunnel: [w2436 w2448] -> w2425
                  tunnel: w2424 -> [w2438 w2447]
                  tunnel: [w2434 w2447] -> w2423
                  tunnel: [w2435 w2445] -> w2417
                  tunnel: w2414 -> [_ w2446]
                  frame False {
                    n547 = call "AC2250 Measure (Main).vi"("ErrIn"=w2437, "VISA Resource Name In"=w2438) -> ("ErrOut"=w2436:errorcluster, "Value"=w2435:dbl, "VISA Resource Name Out"=w2434:refnum<visa-resource-name>)  [unwired: 5 in, 2 out]
                  }
                  frame True {
                    w2439 = 0.0  # NoNoise
                    w2449 = 360.0  # Plus
                    w2452 = 2  # Row
                    w2451 = 1  # Col
                    # "Sim"
                    n548 = Index Array(array=w2446, index (row)=w2452, index (col)=w2451) -> (element=w2450:dbl)
                    n549 = Random Number (0-1)() -> (number: 0 to 1=w2443:dbl)
                    n550 = Add(x=w2450, y=w2449) -> (x+y=w2444:dbl)
                    n551 = Subtract(x=w2443, y=0.5) -> (x-y=w2441:dbl)
                    n552 = Multiply(x=w2441, y=0.01) -> ()  [unwired: 1 out]
                    n553 = Add(x=w2439, y=w2444) -> (x+y=w2445:dbl)
                  }
                }
                n554 = Subtract(x=w2417, y=w2422) -> (x-y=w2430:dbl)
                n555 = Replace Array Subset(array=w2418, new element=w2430, index (row)=w2431, index (col)=w2432) -> (w2427:dbl[][])
              }
              frame 6 {
                # "6 - Checks for errors and repeats as req'd"
                n556 = Unbundle By Name(w2455) -> ("status"=w2454:bool, "code"=w2453:i32)
                n557 = case shown="False" w2454 {
                  tunnel: [0 ("Samps/Chl") w2484] -> w2466
                  tunnel: [w2475 w2482] -> w2465
                  tunnel: [w2473 w2481] -> w2464
                  tunnel: [w2475 w2480] -> w2463
                  tunnel: w2461 -> [w2475 w2479]
                  tunnel: w2462 -> [w2473 w2483]
                  tunnel: [errorcluster {"status"=FALSE, "code"=0, "source"=""} ("error out") w2485] -> w2469
                  tunnel: w2453 -> [_ w2490]
                  tunnel: [0 w2486] -> w2457
                  tunnel: w2458 -> [_ w2478]
                  tunnel: w2455 -> [_ w2477]
                  tunnel: [FALSE w2476] -> w2456
                  frame False {
                    # "No error - done"
                  }
                  frame True {
                    w2488 = 3  # Max Tries
                    w2489 = -1074118636  # Out-of-lock freq cond.
                    # "Error - is error a T/O"
                    n558 = Greater Or Equal?(x=w2478, y=w2488) -> (x >= y?=w2487:bool)
                    n559 = Equal?(x=w2489, y=w2490) -> ()  [unwired: 1 out]
                    n560 = case shown="True" w2487 {
                      tunnel: [w2492 0] -> w2486
                      tunnel: [errorcluster {"status"=FALSE, "code"=0, "source"=""} ("error out") w2498] -> w2485
                      tunnel: [0 ("Samps/Chl") 0 ("Samps/Chl")] -> w2484
                      tunnel: w2483 -> [w2495 w2500]
                      tunnel: [w2495 w2500] -> w2482
                      tunnel: [w2495 w2500] -> w2481
                      tunnel: [w2494 w2499] -> w2480
                      tunnel: w2479 -> [w2494 w2499]
                      tunnel: w2478 -> [w2493 _]
                      tunnel: w2477 -> [_ w2498]
                      tunnel: [FALSE TRUE] -> w2476
                      frame False {
                        # "Clears error and tries againg"
                        n561 = Increment(x=w2493) -> (x+1=w2492:i32)
                      }
                      frame True {
                        # "Time to give up - too many errors"
                      }
                    }
                  }
                }
              }
            }
            n562 = Or(x=w2259, y=w2292) -> (x .or. y?=w2293:bool)
          }
          frame "Get V3g & Phase" {
            # "Get V3g and Phase"
            n563 = case shown="0, Default" w2544 {
              selector: w2544 -> [w2562 w2582 w2603 w2642 w2662 _ _]
              tunnel: [w2560 w2583 w2602 w2640 w2663 0 ("Samps/Chl") w2718] -> w2541
              tunnel: [w2559 w2577 w2601 w2639 w2657 w2673 w2717] -> w2540
              tunnel: [w2561 w2576 w2600 w2641 w2656 w2673 w2721] -> w2539
              tunnel: w2538 -> [w2559 w2577 w2601 w2639 w2657 w2686 w2720]
              tunnel: w2537 -> [w2561 w2576 w2600 w2641 w2656 w2673 w2719]
              tunnel: [w2559 w2577 w2601 w2639 w2657 w2686 w2716] -> w2536
              tunnel: w2535 -> [_ _ _ _ _ _ _]
              tunnel: w2531 -> [w2551 w2584 w2606 w2630 w2664 w2677 w2715]
              tunnel: w2530 -> [w2554 w2585 w2607 w2634 w2665 w2679 w2708]
              tunnel: [w2552 w2584 w2605 w2633 w2664 w2676 w2715] -> w2529
              tunnel: [w2553 w2585 w2604 w2632 w2665 w2678 w2722] -> w2528
              tunnel: w2526 -> [w2558 w2586 w2595 w2638 w2666 w2681 w2713]
              tunnel: [w2558 w2586 w2595 w2638 w2666 w2681 w2713] -> w2525
              tunnel: [w2557 w2579 w2596 w2637 w2659 w2682 w2714] -> w2524
              tunnel: w2523 -> [_ w2579 w2596 _ w2659 w2682 w2714]
              tunnel: w2522 -> [w2556 w2580 _ w2636 w2660 _ _]
              tunnel: w2521 -> [w2555 w2575 w2592 w2635 w2655 w2671 w2712]
              tunnel: [w2555 w2575 w2593 w2635 w2655 w2680 w2712] -> w2520
              tunnel: w2505 -> [w2547 _ _ w2627 _ _ _]
              tunnel: w2519 -> [w2550 _ w2591 w2631 _ w2672 _]
              tunnel: w2514 -> [w2549 w2574 w2589 w2629 w2654 w2669 w2711]
              tunnel: [w2549 w2574 w2589 w2629 w2654 w2669 w2710] -> w2513
              tunnel: [FALSE FALSE FALSE FALSE FALSE FALSE w2709] -> w2512
              tunnel: w2509 -> [_ _ w2587 _ _ w2667 _]
              frame 0, Default {
                # "0 - Requests Signal voltage"
                n564 = case shown="False" w2550 {
                  tunnel: w2554 -> [w2568 w2571]
                  tunnel: [w2566 w2571] -> w2553
                  tunnel: [w2567 w2572] -> w2552
                  tunnel: w2551 -> [w2569 w2572]
                  frame False {
                    w2565 = FALSE  # Ref
                    n565 = call "AC2250 Measurement Mode.vi"("ErrIn"=w2568, "Measurement Mode"=T6."TOTAL", "VISA Resource Name In"=w2569) -> ("ErrOut"=w2564:errorcluster, "VISA Resource Name Out"=w2563:refnum<visa-resource-name>)  [unwired: 6 in, 1 out]
                    n566 = call "AC2250 Measurement Channel.vi"("ErrIn"=w2564, "Reference"=w2565, "VISA Resource Name In"=w2563) -> ("ErrOut"=w2566:errorcluster, "VISA Resource Name Out"=w2567:refnum<visa-resource-name>)  [unwired: 6 in, 1 out]
                  }
                  frame True {
                    # "Sim"
                  }
                }
                n567 = Add(x=w2547, y=w2556) -> (x+y=w2557:dbl)
                n568 = Increment(x=w2562) -> (x+1=w2560:i32)
              }
              frame 1 {
                # "1 - Waits awhile"
                n569 = Greater Or Equal?(x=w2580, y=w2579) -> (x >= y?=w2578:bool)
                n570 = Increment(x=w2582) -> (x+1=w2581:i32)
                n571 = Select(t=w2581, s=w2578, f=w2582) -> (s? t:f=w2583:i32)
              }
              frame 2 {
                w2594 = 1.41421  # To peak V
                w2598 = 3  # Row
                w2599 = 0  # Col
                # "2 - Gets signal voltage and saves it"
                n572 = case shown="False" w2591 {
                  tunnel: w2607 -> [w2611 w2622]
                  tunnel: w2606 -> [w2612 w2621]
                  tunnel: [w2610 w2621] -> w2605
                  tunnel: [w2608 w2622] -> w2604
                  tunnel: [w2609 w2619] -> w2590
                  tunnel: w2587 -> [_ w2620]
                  frame False {
                    n573 = call "AC2250 Measure (Main).vi"("ErrIn"=w2611, "VISA Resource Name In"=w2612) -> ("ErrOut"=w2608:errorcluster, "Value"=w2609:dbl, "VISA Resource Name Out"=w2610:refnum<visa-resource-name>)  [unwired: 5 in, 2 out]
                  }
                  frame True {
                    w2613 = 0.0  # NoNoise
                    w2623 = 1.41421  # From peak V
                    w2626 = 3  # Row
                    w2625 = 0  # Col
                    # "Sim"
                    n574 = Index Array(array=w2620, index (row)=w2626, index (col)=w2625) -> (element=w2624:dbl)
                    n575 = Random Number (0-1)() -> (number: 0 to 1=w2617:dbl)
                    n576 = Divide(x=w2624, y=w2623) -> (x/y=w2618:dbl)
                    n577 = Subtract(x=w2617, y=0.5) -> (x-y=w2615:dbl)
                    n578 = Multiply(x=w2615, y=0.01) -> ()  [unwired: 1 out]
                    n579 = Add(x=w2613, y=w2618) -> (x+y=w2619:dbl)
                  }
                }
                n580 = Multiply(x=w2594, y=w2590) -> (x*y=w2597:dbl)
                n581 = Replace Array Subset(array=w2592, new element=w2597, index (row)=w2598, index (col)=w2599) -> (w2593:dbl[][])
                n582 = Increment(x=w2603) -> (x+1=w2602:i32)
              }
              frame 3 {
                # "3 - Requests Signal phase angle"
                n583 = case shown="False" w2631 {
                  tunnel: w2634 -> [w2648 w2651]
                  tunnel: [w2647 w2652] -> w2633
                  tunnel: [w2646 w2651] -> w2632
                  tunnel: w2630 -> [w2649 w2652]
                  frame False {
                    w2643 = FALSE  # Ref
                    n584 = call "AC2250 Measurement Mode.vi"("ErrIn"=w2648, "Measurement Mode"=T6."PHASE ANGLE", "VISA Resource Name In"=w2649) -> ("ErrOut"=w2644:errorcluster, "VISA Resource Name Out"=w2645:refnum<visa-resource-name>)  [unwired: 6 in, 1 out]
                    n585 = call "AC2250 Measurement Channel.vi"("ErrIn"=w2644, "Reference"=w2643, "VISA Resource Name In"=w2645) -> ("ErrOut"=w2646:errorcluster, "VISA Resource Name Out"=w2647:refnum<visa-resource-name>)  [unwired: 6 in, 1 out]
                  }
                  frame True {
                    # "Sim"
                  }
                }
                n586 = Increment(x=w2642) -> (x+1=w2640:i32)
                n587 = Add(x=w2627, y=w2636) -> (x+y=w2637:dbl)
              }
              frame 4 {
                # "4 - Waits awhile"
                n588 = Greater Or Equal?(x=w2660, y=w2659) -> (x >= y?=w2658:bool)
                n589 = Increment(x=w2662) -> (x+1=w2661:i32)
                n590 = Select(t=w2661, s=w2658, f=w2662) -> (s? t:f=w2663:i32)
              }
              frame 5 {
                w2675 = 360.0  # Minus
                w2684 = 3  # Row
                w2685 = 1  # Col
                # "5 - Gets phase angle and saves it"
                n591 = case shown="False" w2672 {
                  tunnel: w2679 -> [w2687 w2701]
                  tunnel: [w2688 w2701] -> w2678
                  tunnel: w2677 -> [w2691 w2700]
                  tunnel: [w2690 w2700] -> w2676
                  tunnel: [w2689 w2698] -> w2670
                  tunnel: w2667 -> [_ w2699]
                  frame False {
                    n592 = call "AC2250 Measure (Main).vi"("ErrIn"=w2687, "VISA Resource Name In"=w2691) -> ("ErrOut"=w2688:errorcluster, "Value"=w2689:dbl, "VISA Resource Name Out"=w2690:refnum<visa-resource-name>)  [unwired: 5 in, 2 out]
                  }
                  frame True {
                    w2692 = 0.0  # NoNoise
                    w2702 = 360.0  # Plus
                    w2705 = 3  # Row
                    w2704 = 1  # Col
                    # "Sim"
                    n593 = Index Array(array=w2699, index (row)=w2705, index (col)=w2704) -> (element=w2703:dbl)
                    n594 = Random Number (0-1)() -> (number: 0 to 1=w2696:dbl)
                    n595 = Add(x=w2703, y=w2702) -> (x+y=w2697:dbl)
                    n596 = Subtract(x=w2696, y=0.5) -> (x-y=w2694:dbl)
                    n597 = Multiply(x=w2694, y=0.01) -> ()  [unwired: 1 out]
                    n598 = Add(x=w2692, y=w2697) -> (x+y=w2698:dbl)
                  }
                }
                n599 = Subtract(x=w2670, y=w2675) -> (x-y=w2683:dbl)
                n600 = Replace Array Subset(array=w2671, new element=w2683, index (row)=w2684, index (col)=w2685) -> (w2680:dbl[][])
              }
              frame 6 {
                # "6 - Checks for errors and repeats as req'd"
                n601 = Unbundle By Name(w2708) -> ("status"=w2707:bool, "code"=w2706:i32)
                n602 = case shown="False" w2707 {
                  tunnel: [0 ("Samps/Chl") w2737] -> w2718
                  tunnel: [w2728 w2735] -> w2717
                  tunnel: [w2726 w2734] -> w2716
                  tunnel: [w2728 w2733] -> w2721
                  tunnel: w2719 -> [w2728 w2732]
                  tunnel: w2720 -> [w2726 w2736]
                  tunnel: [errorcluster {"status"=FALSE, "code"=0, "source"=""} ("error out") w2738] -> w2722
                  tunnel: w2706 -> [_ w2743]
                  tunnel: [0 w2739] -> w2710
                  tunnel: w2711 -> [_ w2731]
                  tunnel: w2708 -> [_ w2730]
                  tunnel: [FALSE w2729] -> w2709
                  frame False {
                    # "No error - done"
                  }
                  frame True {
                    w2741 = 3  # Max Tries
                    w2742 = -1074118636  # Out-of-lock freq cond.
                    # "Error - is error a T/O"
                    n603 = Greater Or Equal?(x=w2731, y=w2741) -> (x >= y?=w2740:bool)
                    n604 = Equal?(x=w2742, y=w2743) -> ()  [unwired: 1 out]
                    n605 = case shown="True" w2740 {
                      tunnel: [w2745 0] -> w2739
                      tunnel: [errorcluster {"status"=FALSE, "code"=0, "source"=""} ("error out") w2751] -> w2738
                      tunnel: [0 ("Samps/Chl") 0 ("Samps/Chl")] -> w2737
                      tunnel: w2736 -> [w2748 w2753]
                      tunnel: [w2748 w2753] -> w2735
                      tunnel: [w2748 w2753] -> w2734
                      tunnel: [w2747 w2752] -> w2733
                      tunnel: w2732 -> [w2747 w2752]
                      tunnel: w2731 -> [w2746 _]
                      tunnel: w2730 -> [_ w2751]
                      tunnel: [FALSE TRUE] -> w2729
                      frame False {
                        # "Clears error and tries againg"
                        n606 = Increment(x=w2746) -> (x+1=w2745:i32)
                      }
                      frame True {
                        # "Time to give up - too many errors"
                      }
                    }
                  }
                }
              }
            }
            n607 = Or(x=w2512, y=w2545) -> (x .or. y?=w2546:bool)
          }
          frame "Idle" {
            w2757 = 0
            w2766 = FALSE
            # "Idle - waits for a GO"
            n608 = case shown="5" w2796 {
              selector: w2796 -> [w2811 w2841 w2899 w2918 w2931 _]
              tunnel: w2800 -> [_ w2843 _ _ _ _]
              tunnel: [w2810 w2842 w2898 w2917 w2930 w2958] -> w2799
              tunnel: [w2815 w2829 w2897 w2916 w2943 w2958] -> w2798
              tunnel: [w2815 w2828 w2897 w2916 w2943 w2958] -> w2797
              tunnel: [w2809 w2827 w2896 w2915 T4."Wait x Secs" ("State") w2950] -> w2795
              tunnel: w2794 -> [w2809 w2830 w2896 w2915 w2932 w2957]
              tunnel: [w2809 w2827 w2896 w2915 w2932 w2957] -> w2793
              tunnel: [w2809 w2827 w2896 w2915 w2932 w2950] -> w2792
              tunnel: [w2816 w2840 w2894 w2919 w2947 w2962] -> w2790
              tunnel: w2789 -> [w2816 w2840 w2894 _ w2947 w2962]
              tunnel: [w2814 w2839 w2893 w2921 w2946 w2961] -> w2788
              tunnel: w2787 -> [w2814 w2839 w2893 _ w2946 w2961]
              tunnel: [w2813 w2838 w2895 w2920 w2945 w2960] -> w2786
              tunnel: w2785 -> [w2813 w2838 w2895 _ w2945 w2960]
              tunnel: [w2812 w2837 w2892 w2922 w2944 w2959] -> w2784
              tunnel: w2783 -> [w2812 w2837 w2892 _ w2944 w2959]
              tunnel: [w2806 w2818 w2884 w2912 w2940 w2954] -> w2782
              tunnel: w2781 -> [w2806 w2819 w2884 w2912 w2940 w2954]
              tunnel: [w2807 w2822 w2883 w2913 w2941 w2955] -> w2780
              tunnel: w2779 -> [w2808 w2836 w2891 _ w2942 w2956]
              tunnel: [w2808 w2836 w2891 T5."<none>" ("Signal") w2942 w2956] -> w2778
              tunnel: w2776 -> [w2807 w2823 w2883 w2913 w2941 w2955]
              tunnel: [w2805 w2820 w2881 w2911 w2939 w2953] -> w2772
              tunnel: w2771 -> [w2805 w2821 w2881 w2911 w2939 w2953]
              tunnel: [w2804 w2834 w2890 w2910 w2938 w2952] -> w2770
              tunnel: w2769 -> [w2804 w2835 w2890 w2910 w2938 w2952]
              tunnel: [w2817 w2832 w2888 w2909 w2937 w2951] -> w2768
              tunnel: w2767 -> [w2817 w2833 w2888 w2909 w2937 w2951]
              tunnel: w2765 -> [_ w2831 _ _ _ _]
              tunnel: w2764 -> [_ w2829 _ _ _ _]
              tunnel: w2763 -> [_ w2828 _ _ _ _]
              tunnel: w2762 -> [w2802 w2826 w2886 w2908 _ w2949]
              tunnel: [w2802 w2826 w2886 w2908 w2935 w2949] -> w2761
              tunnel: w2760 -> [_ _ _ _ w2934 _]
              tunnel: w2759 -> [w2801 w2824 w2885 w2907 w2929 w2948]
              tunnel: [w2801 w2825 w2885 w2907 w2929 w2948] -> w2758
              frame 0, Default {
                w2815 = 0
                # "0 - resets things as req'd"
                n609 = global write "Global ER2007.vi" "GCD Prog"(bool[] [FALSE, FALSE, FALSE, FALSE, FALSE, FALSE] ("GCD Prog")) -> ()
                n610 = Increment(x=w2811) -> (x+1=w2810:i32)
              }
              frame 1 {
                # "1 - waiting for a GO or STOP"
                n611 = case shown="True" w2843 {
                  tunnel: [w2848 w2872] -> w2842
                  tunnel: w2841 -> [w2848 w2873]
                  tunnel: w2835 -> [w2854 _]
                  tunnel: [w2854 w2870] -> w2834
                  tunnel: w2833 -> [w2853 _]
                  tunnel: [w2853 w2864] -> w2832
                  tunnel: [w2850 w2869] -> w2827
                  tunnel: w2830 -> [w2851 w2869]
                  tunnel: w2831 -> [w2852 _]
                  tunnel: [w2847 w2866] -> w2825
                  tunnel: w2824 -> [w2847 _]
                  tunnel: w2823 -> [w2845 _]
                  tunnel: [w2845 w2855] -> w2822
                  tunnel: w2821 -> [w2844 w2861]
                  tunnel: [w2844 w2860] -> w2820
                  tunnel: w2819 -> [w2846 _]
                  tunnel: [w2846 w2856] -> w2818
                  frame False {
                    n612 = Select(t=T4."Stop" ("State"), s=w2852, f=w2851) -> (s? t:f=w2850:T4)
                  }
                  frame True {
                    # "GO - grabs input vars"
                    # "Grabs current\n\"New Vol\" flag"
                    n613 = global read "Global ER2007.vi" "New Vol"() -> (w2865:bool[])
                    n614 = case shown="False" "Use Locals" {
                      tunnel: [w2875 "DataCell"] -> w2862
                      tunnel: w2861 -> [_ _]
                      tunnel: [w2874 w2876] -> w2859
                      frame False {
                        n615 = global read "Global ER2007.vi" "Test Info"() -> (w2874:T3)
                        n616 = global read "Global ER2007.vi" "DataCell"() -> (w2875:i32)
                        n617 = local write "Test Info In"(w2874) -> ()
                      }
                      frame True {
                        n618 = local read "Test Info In"() -> (w2876:T3)
                      }
                    }
                    "Cell ID" <- w2862
                    n619 = global write "Global ER2007.vi" "GCD Err"(FALSE ("GCD Err")) -> ()
                    n620 = global read "Global ER2007.vi" "Mark String"() -> (w2867:string[])
                    n621 = Unbundle By Name(w2859) -> ("Cell Data"=w2858:T12)
                    n622 = Decrement(x=w2862) -> (x-1=w2855:i32)
                    n623 = Index Array(array=w2865, index=w2855) -> (element=w2864:bool)
                    n624 = Get Date/Time In Seconds() -> (seconds since 1Jan1904=w2871:timestamp)
                    n625 = Index Array(array=w2858, index=w2855) -> (element=w2860:T11)
                    n626 = To Double Precision Float(number=w2871) -> (double precision float=w2870:dbl)
                    n627 = Index Array(array=w2867, index=w2855) -> (element=w2866:string)
                    n628 = Index Array(array="Local Test Resistivity Input Data (sim)", index (dim 0)=w2855) -> (element=w2856:dbl[][])  [unwired: 2 in]
                    n629 = Increment(x=w2873) -> (x+1=w2872:i32)
                  }
                }
              }
              frame 2 {
                w2897 = 0
                # "2 - gets input data; resets flags"
                n630 = case shown="True" w2888 {
                  tunnel: w2883 -> [_ w2906]
                  frame False {
                  }
                  frame True {
                    # "Reset flags"
                    n631 = global read "Global ER2007.vi" "Mark String"() -> (w2905:string[])
                    n632 = global read "Global ER2007.vi" "New Vol"() -> (w2902:bool[])
                    n633 = Replace Array Subset(array=w2905, new element="", index=w2906) -> (w2903:string[])
                    n634 = Replace Array Subset(array=w2902, new element=FALSE ("New Vol"), index=w2906) -> (w2900:bool[])
                    n635 = global write "Global ER2007.vi" "Mark String"(w2903) -> ()
                    n636 = global write "Global ER2007.vi" "New Vol"(w2900) -> ()
                  }
                }
                n637 = local write "Abort Message"("") -> ()
                n638 = Unbundle By Name(w2881) -> ("Last Resistor"=→"Last Resistor":T1)
                n639 = local write "Errs"(bool[] [FALSE, FALSE, FALSE, FALSE, FALSE] ("Errs")) -> ()
                n640 = global write "Global ER2007.vi" "GCD Go"(FALSE ("GCD Go")) -> ()
                n641 = Increment(x=w2899) -> (x+1=w2898:i32)
                "RS Done" <- FALSE ("RS Done")
                "Swch Box" <- bool[] [FALSE, FALSE, FALSE, FALSE] ("Swch Box")
              }
              frame 3 {
                w2916 = 0
                w2920 = T2 {"R2P (k)"=0.0, "C2P (pf)"=0.0, "R12 (k)"=0.0, "C12 (pf)"=0.0, "R23 (k)"=0.0, "C23 (pf)"=0.0, "R3G (k)"=0.0, "C3G (pf)"=0.0, "R13 (k)"=0.0, "C13 (pf)"=0.0}  # ResistParams
                w2924 = 2  # Cols
                w2925 = 4  # Rows
                w2927 = 15  # Must set to exact size
                # "3 - inits things"
                n642 = Initialize Array(0.0 ("element"), w2925, w2924) -> (w2921:dbl[][])
                n643 = Initialize Array(0.0 ("element")) -> (w2922:dbl[])  [unwired: 1 in]
                n644 = Initialize Array(0.0 ("element"), w2927) -> (w2919:dbl[])
                n645 = Increment(x=w2918) -> (x+1=w2917:i32)
              }
              frame 4 {
                w2943 = 0
                # "4 - small wait for GPIB"
                n646 = Add(x=1.0, y=w2934) -> (x+y=w2935:dbl)
                n647 = Increment(x=w2931) -> (x+1=w2930:i32)
              }
              frame 5 {
                w2950 = T4."Initialize" ("State")
                w2958 = 0
                # "5 - start at Initialize"
              }
            }
          }
          frame "Initialize" {
            # "Initialize"
            n648 = case shown="3" w3001 {
              selector: w3001 -> [w3020 w3072 w3100 w3111 w3122 w3133 w3144 _ _]
              tunnel: [w3010 w3067 w3095 w3106 w3117 w3128 w3139 w3149 w3159] -> w3000
              tunnel: w2999 -> [w3002 w3067 w3095 w3106 w3117 w3128 w3139 w3149 w3159]
              tunnel: [w3012 w3068 w3096 w3107 w3118 w3129 w3140 w3150 w3160] -> w2998
              tunnel: [w3019 w3071 w3099 w3110 w3121 w3132 w3143 9 w3161] -> w2992
              tunnel: [0 ("Samps/Chl") 0 ("Samps/Chl") 0 ("Samps/Chl") 0 ("Samps/Chl") 0 ("Samps/Chl") 0 ("Samps/Chl") 0 ("Samps/Chl") 0 ("Samps/Chl") w3161] -> w2991
              tunnel: [T4."Generator OFF" ("State") w3069 T4."Reset Auto Mode" ("State") T4."Reset Cell Select Relays" ("State") T4."Reset Resistor Select Relays" ("State") T4."Reset Signal Select Relays" ("State") T4."Set Freq & Ampltd" ("State") w3151 w3154] -> w2996
              tunnel: w2997 -> [w3017 w3069 w3097 w3108 w3119 w3130 w3141 w3151 _]
              tunnel: [w3017 w3069 w3097 w3108 w3119 w3130 w3141 w3151 w3154] -> w2995
              tunnel: w2994 -> [w3008 w3061 w3092 w3103 w3114 w3125 w3136 w3146 w3156]
              tunnel: [w3009 w3062 w3092 w3103 w3114 w3125 w3136 w3146 w3156] -> w2993
              tunnel: w2990 -> [w3016 w3055 w3093 w3104 w3115 w3126 w3137 w3147 w3157]
              tunnel: [w3016 w3060 w3093 w3104 w3115 w3126 w3137 w3147 w3157] -> w2989
              tunnel: w2988 -> [w3015 w3056 w3094 w3105 w3116 w3127 w3138 w3148 w3158]
              tunnel: [w3015 w3064 w3094 w3105 w3116 w3127 w3138 w3148 w3158] -> w2987
              tunnel: w2985 -> [w3005 w3068 w3096 w3107 w3118 w3129 w3140 w3150 w3160]
              tunnel: w2974 -> [w3014 w3066 _ w3102 w3113 w3124 w3135 w3145 w3155]
              tunnel: [w3014 w3066 errorcluster {"status"=FALSE, "code"=0, "source"=""} ("error out") w3102 w3113 w3124 w3135 w3145 w3155] -> w2973
              tunnel: w2968 -> [w3011 _ _ _ _ _ _ _ _]
              tunnel: w2967 -> [_ w3063 _ _ _ _ _ _ _]
              tunnel: w2966 -> [w3006 w3057 _ _ _ _ _ _ _]
              tunnel: w2965 -> [w3003 _ _ _ _ _ _ _ _]
              frame 0, Default {
                # "0 - Inits Agilent 32333 & turns it OFF.\nIF PC ID=1, asserts IFC to get control"
                n649 = case shown="False" w3006 {
                  tunnel: [w3026 w3046] -> w3012
                  tunnel: w3011 -> [w3025 w3042]
                  tunnel: [w3024 w3044] -> w3004
                  tunnel: w3002 -> [_ w3045]
                  tunnel: w3005 -> [_ w3046]
                  tunnel: w3003 -> [_ w3043]
                  frame False {
                    n650 = case shown="False" w3025 {
                      tunnel: [w3030 refnum<visa-resource-name> refnum ("dup VISA session")] -> w3026
                      tunnel: [w3029 errorcluster {"status"=FALSE, "code"=0, "source"=""} ("error out")] -> w3024
                      frame False {
                        w3031 = FALSE  # Output Enabled? (T: Yes)
                        w3034 = TRUE  # Reset (T: Reset)
                        n651 = global read "Global ER2007.vi" "HP Addr"() -> (w3028:string)
                        n652 = Concatenate Strings("GPIB::" ("string"), w3028, "::INSTR" ("string")) -> (w3036:string)
                        n653 = Type Cast(type=refnum<visa-resource-name> "GPIB::10::INSTR" ("Instrument Resource Name"), x=w3036) -> (*(type *) &x=w3035:refnum<visa-resource-name>)
                        n654 = call "ag33xxx - Initialize.vi"("Reset (T: Reset)"=w3034, "Instrument Resource Name"=w3035) -> ("error out"=w3033:errorcluster, "dup VISA session"=w3032:refnum<visa-resource-name>)  [unwired: 8 in]
                        n655 = call "ag33xxx - Output Enabled.vi"("error in (no error)"=w3033, "Output Enabled? (T: Yes)"=w3031, "VISA session"=w3032) -> ("error out"=w3029:errorcluster, "dup VISA session"=w3030:refnum<visa-resource-name>)  [unwired: 7 in]
                        "HP Live" <- TRUE ("HP Live")
                      }
                      frame True {
                        # "Sim"
                      }
                    }
                  }
                  frame True {
                    # "Init once in effect.  If PC #1\nassert IFC to gain CIC control"
                    n656 = case shown="2" w3043 {
                      tunnel: w3045 -> [w3049 w3054]
                      tunnel: [w3048 w3054] -> w3044
                      tunnel: w3042 -> [w3047 _]
                      frame 1, Default {
                        n657 = case shown="False" w3047 {
                          tunnel: w3049 -> [w3052 w3053]
                          tunnel: [w3051 w3053] -> w3048
                          frame False {
                            n658 = SendIFC(2:w3052, 3:0 ("bus")) -> (0:w3051:errorcluster)  [unwired: 1 out]
                          }
                          frame True {
                            # "SimHP"
                          }
                        }
                      }
                      frame 2 {
                      }
                    }
                  }
                }
                n659 = case shown="Error" w3002 {
                  tunnel: [w3022 w3023] -> w3010
                  tunnel: w3004 -> [w3021 w3023]
                  frame No Error {
                    n660 = call <vilib>:"Simple Error Handler.vi"("error in (no error)"=w3021) -> ("error out"=w3022:errorcluster)  [unwired: 4 in, 4 out]
                  }
                  frame Error {
                  }
                }
                n661 = Unbundle By Name(w3004) -> ("status"=w3007:bool)
                n662 = Increment(x=w3020) -> (x+1=w3019:i32)
                n663 = Or(x=w3007, y=w3008) -> (x .or. y?=w3009:bool)
              }
              frame 1 {
                # "1 - Inits NAII Phasemeter"
                n664 = case shown="False" w3057 {
                  tunnel: [w3075 w3088] -> w3064
                  tunnel: w3063 -> [w3074 _]
                  tunnel: [w3073 w3089] -> w3059
                  tunnel: w3056 -> [_ w3088]
                  tunnel: w3055 -> [_ w3089]
                  frame False {
                    n665 = case shown="False" w3074 {
                      tunnel: [w3080 refnum<visa-resource-name> refnum ("instrument handle out")] -> w3075
                      tunnel: [w3078 errorcluster {"status"=FALSE, "code"=0, "source"=""} ("error out")] -> w3073
                      frame False {
                        # "Was NAI2250 Configure.vi"
                        # "Was NAI2250 Initialize.vi"
                        n666 = global read "Global ER2007.vi" "NAI Addr"() -> (w3083:string)
                        n667 = Concatenate Strings("GPIB::" ("string"), w3083, "::INSTR" ("string")) -> (w3081:string)
                        n668 = call "AC2250 Initialize.vi"("VISA Resource Name In"=w3081) -> ("ErrOut"=w3077:errorcluster, "VISA Resource Name Out"=w3079:refnum<visa-resource-name>)  [unwired: 9 in]
                        n669 = call "AC2250 Configure.vi"("ErrIn"=w3077, "Measurement Mode"=T6."TOTAL", "VISA Resource Name In"=w3079) -> ("ErrOut"=w3078:errorcluster, "VISA Resource Name Out"=w3080:refnum<visa-resource-name>)  [unwired: 6 in, 1 out]
                        "NAII Live" <- TRUE ("NAII Live")
                      }
                      frame True {
                        # "Sim"
                      }
                    }
                  }
                  frame True {
                    # "Init once in effect"
                  }
                }
                n670 = global write "Global ER2007.vi" "GCD Prog"(bool[] [TRUE, FALSE, FALSE, FALSE, FALSE, FALSE] ("GCD Prog")) -> ()
                n671 = Unbundle By Name(w3059) -> ("status"=w3058:bool)
                n672 = Increment(x=w3072) -> (x+1=w3071:i32)
                n673 = call <vilib>:"Simple Error Handler.vi"("error in (no error)"=w3059) -> ("error out"=w3060:errorcluster)  [unwired: 4 in, 4 out]
                n674 = Or(x=w3058, y=w3061) -> (x .or. y?=w3062:bool)
              }
              frame 2 {
                # "2 - Turn Auto Mode Off"
                n675 = Increment(x=w3100) -> (x+1=w3099:i32)
              }
              frame 3 {
                # "3 - Reset Cell Select"
                n676 = Increment(x=w3111) -> (x+1=w3110:i32)
              }
              frame 4 {
                # "4 - Reset Resistor Select"
                n677 = Increment(x=w3122) -> (x+1=w3121:i32)
              }
              frame 5 {
                # "5 - Reset Signal Select"
                n678 = Increment(x=w3133) -> (x+1=w3132:i32)
              }
              frame 6 {
                # "6 - Sets generator amplitude and frequency"
                n679 = Increment(x=w3144) -> (x+1=w3143:i32)
              }
              frame 7 {
                # "Spare Phase"
              }
              frame 9 {
                w3154 = T4."Main Test Engine" ("State")
                w3161 = 0
                # "9 - End of initialize"
              }
            }
          }
          frame "Main Test Engine" {
            # "Main Test Engine"
            n680 = case shown="0, Default" w3198 {
              selector: w3198 -> [w3215 w3227 w3236 w3245 w3254 w3265 w3274 w3285 w3294 w3303 w3320 w3348 w3359 w3368 w3377 w3388 w3397 _]
              tunnel: [w3214 w3226 w3235 w3244 w3253 w3264 w3273 w3284 w3293 w3302 w3322 w3347 w3358 w3367 w3376 w3387 w3396 w3404] -> w3197
              tunnel: [w3201 w3225 w3234 w3243 w3252 w3263 w3272 w3283 w3292 w3301 w3335 w3346 w3357 w3366 w3375 w3386 w3395 w3404] -> w3196
              tunnel: w3195 -> [w3211 w3222 w3231 w3240 w3249 w3261 w3270 w3281 w3290 w3299 w3311 w3343 w3355 w3362 w3371 w3384 w3391 w3401]
              tunnel: w3189 -> [w3213 w3223 w3232 w3241 w3250 _ w3267 _ w3287 w3296 w3332 w3344 _ w3363 w3372 _ w3392 w3402]
              tunnel: [w3213 w3223 w3232 w3241 w3250 w3258 w3267 w3278 w3287 w3296 w3332 w3344 w3352 w3363 w3372 w3381 w3392 w3402] -> w3188
              tunnel: [w3211 w3222 w3231 w3240 w3249 w3261 w3270 w3281 w3290 w3299 w3311 w3343 w3355 w3362 w3371 w3384 w3391 w3401] -> w3187
              tunnel: [w3212 w3221 w3230 w3239 w3248 w3260 w3269 w3280 w3289 w3298 w3334 w3342 w3354 w3361 w3370 w3383 w3390 w3400] -> w3185
              tunnel: w3184 -> [w3212 w3221 w3230 w3239 w3248 w3260 w3269 w3280 w3289 w3298 w3334 w3342 w3354 w3361 w3370 w3383 w3390 w3400]
              tunnel: [w3203 T4."Set Auto Mode" ("State") T4."Set Resistor Select Relays" ("State") T4."Set Signal Select Relays" ("State") T4."Set Cell Select Relays" ("State") T4."Wait x Secs" ("State") T4."Generator ON" ("State") T4."Wait x Secs" ("State") T4."Get Vs & Phase" ("State") T4."Get V1g & Phase" ("State") w3327 T4."Set Signal Select Relays" ("State") T4."Wait x Secs" ("State") T4."Get V2g & Phase" ("State") T4."Set Signal Select Relays" ("State") T4."Wait x Secs" ("State") T4."Get V3g & Phase" ("State") w3398] -> w3183
              tunnel: [w3202 w3224 w3233 w3242 w3251 w3262 w3271 w3282 w3291 w3300 w3323 w3341 w3356 w3365 w3374 w3385 w3394 w3399] -> w3182
              tunnel: [w3204 w3224 w3233 w3242 w3251 w3262 w3271 w3282 w3291 w3300 w3323 w3341 w3356 w3365 w3374 w3385 w3394 w3398] -> w3181
              tunnel: w3180 -> [w3205 _ _ _ _ _ _ _ _ _ _ _ _ _ _ _ _ _]
              tunnel: w3179 -> [w3206 _ _ _ _ _ _ _ _ _ _ _ _ _ _ _ _ _]
              tunnel: w3178 -> [w3207 w3224 w3233 w3242 w3251 w3262 w3271 w3282 w3291 w3300 w3323 w3341 w3356 w3365 w3374 w3385 w3394 w3399]
              tunnel: [w3201 w3225 w3234 w3243 w3252 w3263 w3272 w3283 w3292 w3301 w3335 w3346 w3357 w3366 w3375 w3386 w3395 w3404] -> w3177
              tunnel: [w3200 w3220 w3229 T5."Signal 1" ("Signal") w3247 w3259 w3268 w3279 w3288 w3297 w3333 T5."Signal 2" ("Signal") w3353 w3364 T5."Signal 3" ("Signal") w3382 w3393 w3403] -> w3176
              tunnel: w3175 -> [w3200 w3220 w3229 _ w3247 w3259 w3268 w3279 w3288 w3297 w3333 _ w3353 w3364 _ w3382 w3393 w3403]
              tunnel: w3174 -> [_ _ _ _ _ w3257 _ w3277 _ _ _ _ w3351 _ _ w3380 _ _]
              tunnel: w3173 -> [_ _ _ _ _ _ _ _ _ _ w3328 _ _ _ _ _ _ _]
              frame 0, Default {
                w3201 = 0 ("Samps/Chl")
                # "0 - determines if resistor needs\nto be selected"
                n681 = Unbundle By Name(w3211) -> ("Last Resistor"=w3210:T1)
                n682 = Equal?(x=w3210, y=T1."<none>" ("Last Resistor")) -> (x = y?=w3208:bool)
                n683 = global write "Global ER2007.vi" "GCD Prog"(bool[] [FALSE, TRUE, FALSE, FALSE, FALSE, FALSE] ("GCD Prog")) -> ()
                n684 = case shown="True" w3208 {
                  tunnel: w3207 -> [w3216 w3218]
                  tunnel: w3206 -> [_ _]
                  tunnel: w3205 -> [_ _]
                  tunnel: [w3216 w3218] -> w3204
                  tunnel: [w3216 T4."Determine Series Resistor" ("State")] -> w3203
                  tunnel: [w3216 w3218] -> w3202
                  frame False {
                  }
                  frame True {
                  }
                }
                n685 = Increment(x=w3215) -> (x+1=w3214:i32)
              }
              frame 1 {
                w3225 = 0 ("Samps/Chl")
                # "1 - Auto Mode ON"
                n686 = Increment(x=w3227) -> (x+1=w3226:i32)
              }
              frame 2 {
                w3234 = 0 ("Samps/Chl")
                # "2 - set Resistor Select Relays"
                n687 = Increment(x=w3236) -> (x+1=w3235:i32)
              }
              frame 3 {
                w3243 = 0 ("Samps/Chl")
                # "3 - set Signal Select Relays"
                n688 = Increment(x=w3245) -> (x+1=w3244:i32)
              }
              frame 4 {
                w3252 = 0 ("Samps/Chl")
                # "4 - set Cell Select Relays"
                n689 = Increment(x=w3254) -> (x+1=w3253:i32)
              }
              frame 5 {
                w3256 = 1.0  # 1-sec
                w3263 = 0 ("Samps/Chl")
                # "5 - small wait"
                n690 = Increment(x=w3265) -> (x+1=w3264:i32)
                n691 = Add(x=w3256, y=w3257) -> (x+y=w3258:dbl)
              }
              frame 6 {
                w3272 = 0 ("Samps/Chl")
                # "6 - Generator ON"
                n692 = Increment(x=w3274) -> (x+1=w3273:i32)
              }
              frame 7 {
                w3283 = 0 ("Samps/Chl")
                # "7 - small wait"
                n693 = global read "Global ER2007.vi" "GenOnWait"() -> (w3275:dbl)
                n694 = Increment(x=w3285) -> (x+1=w3284:i32)
                n695 = Add(x=w3275, y=w3277) -> (x+y=w3278:dbl)
              }
              frame 8 {
                w3292 = 0 ("Samps/Chl")
                # "8 - get Vs and phase"
                n696 = Increment(x=w3294) -> (x+1=w3293:i32)
              }
              frame 9 {
                w3301 = 0 ("Samps/Chl")
                # "9 - get V1g and phase"
                n697 = Increment(x=w3303) -> (x+1=w3302:i32)
              }
              frame 10 {
                w3318 = 9  # Jump back & try again
                w3325 = 0.01  # From %
                w3329 = 1  # Row
                w3331 = 0  # Row
                w3330 = 0  # Col
                w3335 = 0 ("Samps/Chl")
                # "TRUE if V1g\nlevel OK"
                # "10 - checks to see if signals are\nin a reasonable range"
                n698 = global read "Global ER2007.vi" "DftRsLoT/H"() -> (w3304:dbl)
                n699 = global read "Global ER2007.vi" "DftRsHiT/H"() -> (w3305:dbl)
                n700 = Unbundle By Name(w3311) -> ("Last Resistor"=w3310:T1)
                n701 = Index Array(array=w3328, index (row) #1=w3331, index (col) #1=w3330, index (row) #2=w3329, index (col) #2=w3330) -> (element #1=w3326:dbl, element #2=w3306:dbl)
                n702 = Equal?(x=T1."Resistor 1" ("Last Resistor"), y=w3310) -> (x = y?=w3307:bool)
                n703 = Compound Arithmetic op=MULTIPLY(w3325, w3305, w3326) -> (w3324:dbl)
                n704 = Compound Arithmetic op=MULTIPLY(w3325, w3304, w3326) -> (w3312:dbl)
                n705 = local read "RS Done"() -> (w3315:bool)
                n706 = Less?(x=w3306, y=w3312) -> (x < y?=w3308:bool)
                n707 = In Range and Coerce(upper limit=w3324, x=w3306, lower limit=w3312) -> (In Range?=w3316:bool)  [unwired: 1 out]
                n708 = Or(x=w3315, y=w3316) -> (x .or. y?=w3314:bool)
                n709 = case shown="False" w3314 {
                  selector: w3314 -> [_ w3339]
                  tunnel: [w3336 w3339] -> w3313
                  tunnel: w3308 -> [w3338 _]
                  tunnel: w3307 -> [w3337 _]
                  frame False {
                    n710 = And(x=w3338, y=w3337) -> (x .and. y?=w3336:bool)
                  }
                  frame True {
                  }
                }
                n711 = Increment(x=w3320) -> (x+1=w3321:i32)
                n712 = Subtract(x=w3320, y=w3318) -> (x-y=w3319:i32)
                n713 = Select(t=w3321, s=w3313, f=w3319) -> (s? t:f=w3322:i32)
                n714 = Select(t=w3323, s=w3313, f=T4."Determine Series Resistor" ("State")) -> (s? t:f=w3327:T4)
              }
              frame 11 {
                w3346 = 0 ("Samps/Chl")
                # "11 - Set Signal Select Relays"
                n715 = Increment(x=w3348) -> (x+1=w3347:i32)
              }
              frame 12 {
                w3350 = 1.0  # 1-sec
                w3357 = 0 ("Samps/Chl")
                # "12 - small wait"
                n716 = Increment(x=w3359) -> (x+1=w3358:i32)
                n717 = Add(x=w3350, y=w3351) -> (x+y=w3352:dbl)
              }
              frame 13 {
                w3366 = 0 ("Samps/Chl")
                # "13 - Get V2g and phase"
                n718 = Increment(x=w3368) -> (x+1=w3367:i32)
              }
              frame 14 {
                w3375 = 0 ("Samps/Chl")
                # "14 - Set Signal Select Relays"
                n719 = Increment(x=w3377) -> (x+1=w3376:i32)
              }
              frame 15 {
                w3379 = 1.0  # 1-sec
                w3386 = 0 ("Samps/Chl")
                # "15 - small wait"
                n720 = Increment(x=w3388) -> (x+1=w3387:i32)
                n721 = Add(x=w3379, y=w3380) -> (x+y=w3381:dbl)
              }
              frame 16 {
                w3395 = 0 ("Samps/Chl")
                # "16 - Get V3g and phase"
                n722 = Increment(x=w3397) -> (x+1=w3396:i32)
              }
              frame 17 {
                w3398 = T4."Final Values" ("State")
                w3404 = 0
                # "17 - all done"
              }
            }
          }
          frame "Reset Auto Mode" {
            w3408 = 0  # AutoMode
            w3416 = FALSE  # OFF/ON
            # "Reset Auto Mode"
            n723 = Index Array(array=w3432, index=4) -> (element=w3415:bool)
            n724 = local read "Swch Box"() -> (w3407:bool[])
            n725 = call "Switch Box Auto Mode Control.vi"("OFF/ON"=w3416, "Invert"=w3415, "ErrIn"=w3419, "SimOn"=w3417) -> ("ErrOut"=w3418:errorcluster)  [unwired: 11 in]
            n726 = Replace Array Subset(array=w3407, new element=FALSE ("new element/subarray"), index=w3408) -> (w3406:bool[])
            n727 = local write "Swch Box"(w3406) -> ()
            n728 = Unbundle By Name(w3418) -> ("status"=w3410:bool)
          }
          frame "Reset Cell Select Relays" {
            w3443 = 1  # CellSel
            w3453 = TRUE  # All OFF
            # "Reset Cell Select Relays"
            n729 = Array Subset(array=w3470, index=9, length=4) -> (w3452:bool[])
            n730 = local read "Swch Box"() -> (w3445:bool[])
            n731 = call "Switch Box Cell Select Control.vi"("Cell"=w3451, "All OFF"=w3453, "Dout Inv"=w3452, "ErrIn"=w3456, "SimOn"=w3454) -> ("ErrOut"=w3455:errorcluster)  [unwired: 10 in]
            n732 = Replace Array Subset(array=w3445, new element=FALSE ("new element/subarray"), index=w3443) -> (w3444:bool[])
            n733 = local write "Swch Box"(w3444) -> ()
            n734 = Unbundle By Name(w3455) -> ("status"=w3447:bool)
          }
          frame "Reset Resistor Select Relays" {
            w3487 = 2  # ResistSel
            w3496 = TRUE  # All OFF
            # "Reset Resistor Select Relays"
            n735 = Index Array(array=w3512, index #1=5 ("index"), index #2=7 ("length"), index #3=8 ("length")) -> (element #1=w3483:bool, element #2=w3482:bool, element #3=w3481:bool)
            n736 = Build Array(w3483, w3482, w3481) -> (w3480:bool[])
            n737 = local read "Swch Box"() -> (w3489:bool[])
            n738 = call "Switch Box Resistor Select Control.vi"("All OFF"=w3496, "Dout Inv"=w3480, "ErrIn"=w3499, "SimOn"=w3497) -> ("ErrOut"=w3498:errorcluster)  [unwired: 11 in]
            n739 = Replace Array Subset(array=w3489, new element=FALSE ("new element/subarray"), index=w3487) -> (w3488:bool[])
            n740 = local write "Swch Box"(w3488) -> ()
            n741 = Unbundle By Name(w3498) -> ("status"=w3491:bool)
          }
          frame "Reset Signal Select Relays" {
            w3523 = 3  # SignalSel
            w3533 = TRUE  # All OFF
            # "Reset Signal Select Relays"
            n742 = Array Subset(array=w3550, index=1, length=2) -> (w3532:bool[])
            n743 = local read "Swch Box"() -> (w3525:bool[])
            n744 = call "Switch Box Signal Select Control.vi"("All OFF"=w3533, "Dout Inv"=w3532, "ErrIn"=w3536, "SimOn"=w3534) -> ("ErrOut"=w3535:errorcluster)  [unwired: 11 in]
            n745 = Replace Array Subset(array=w3525, new element=FALSE ("new element/subarray"), index=w3523) -> (w3524:bool[])
            n746 = local write "Swch Box"(w3524) -> ()
            n747 = Unbundle By Name(w3535) -> ("status"=w3527:bool)
          }
          frame "Set Auto Mode" {
            w3561 = 0  # AutoMode
            w3571 = TRUE  # OFF/ON
            # "Set Auto Mode"
            n748 = Index Array(array=w3587, index=4) -> (element=w3570:bool)
            n749 = local read "Swch Box"() -> (w3563:bool[])
            n750 = call "Switch Box Auto Mode Control.vi"("OFF/ON"=w3571, "Invert"=w3570, "ErrIn"=w3574, "SimOn"=w3572) -> ("ErrOut"=w3573:errorcluster)  [unwired: 11 in]
            n751 = Replace Array Subset(array=w3563, new element=TRUE ("new element/subarray"), index=w3561) -> (w3562:bool[])
            n752 = local write "Swch Box"(w3562) -> ()
            n753 = Unbundle By Name(w3573) -> ("status"=w3565:bool)
          }
          frame "Set Cell Select Relays" {
            w3598 = 1  # CellSel
            # "Set Cell Select Relays"
            n754 = Array Subset(array=w3624, index=9, length=4) -> (w3607:bool[])
            n755 = local read "Swch Box"() -> (w3600:bool[])
            n756 = call "Switch Box Cell Select Control.vi"("Cell"=w3606, "Dout Inv"=w3607, "ErrIn"=w3609, "SimOn"=w3610) -> ("ErrOut"=w3608:errorcluster)  [unwired: 11 in]
            n757 = Replace Array Subset(array=w3600, new element=TRUE ("new element/subarray"), index=w3598) -> (w3599:bool[])
            n758 = local write "Swch Box"(w3599) -> ()
            n759 = Unbundle By Name(w3608) -> ("status"=w3602:bool)
          }
          frame "Set Freq & Ampltd" {
            # "Set Generator Frequency\nand Amplitude"
            n760 = case shown="False" w3640 {
              tunnel: w3660 -> [w3672 w3673]
              tunnel: w3659 -> [w3671 w3674]
              tunnel: [w3670 w3674] -> w3658
              tunnel: [w3669 w3673] -> w3654
              tunnel: w3653 -> [w3668 _]
              frame False {
                w3666 = u16 1 items=["DC"=0, "Sine"=1, "Square"=2, "Triangle"=3, "Ramp"=4, "Pulse"=6, "Noise"=7, "Sinc"=8, "Neg. Ramp"=9, "Exp. Rise"=10, "Exp. Fall"=11, "Cardiac"=12, "Volatile"=13, "User Def. Wfm"=14] ("Waveform Shape (1: Sine)")
                w3667 = u16 1 items=["Vpp", "Vrms", "dB"] ("Unit (0: Vpp)")
                n761 = Unbundle By Name(w3668) -> ("Frequency"=w3665:dbl, "Amplitude"=w3664:dbl)
                n762 = call "ag33xxx - Config Waveform.vi"("VISA session"=w3671, "Waveform Shape (1: Sine)"=w3666, "Frequency (1000 Hz)"=w3665, "Amplitude (0.1 Vpp)"=w3664, "error in (no error)"=w3672, "Unit (0: Vpp)"=w3667) -> ("dup VISA session"=w3670:refnum<visa-resource-name>, "error out"=w3669:errorcluster)  [unwired: 8 in]
              }
              frame True {
                # "Sim"
              }
            }
            n763 = Unbundle By Name(w3654) -> ("status"=w3635:bool)
          }
          frame "Set Resistor Select Relays" {
            w3684 = 2  # ResistSel
            # "Set Resistor Select Relays"
            n764 = Index Array(array=w3676, index #1=5 ("index"), index #2=7 ("length"), index #3=8 ("length")) -> (element #1=w3679:bool, element #2=w3678:bool, element #3=w3677:bool)
            n765 = Build Array(w3679, w3678, w3677) -> (w3675:bool[])
            n766 = local read "Swch Box"() -> (w3686:bool[])
            n767 = Unbundle By Name(w3708) -> ("Last Resistor"=w3693:T1)
            n768 = call "Switch Box Resistor Select Control.vi"("Resistor"=w3693, "Dout Inv"=w3675, "ErrIn"=w3696, "SimOn"=w3694) -> ("ErrOut"=w3695:errorcluster)  [unwired: 11 in]
            n769 = Replace Array Subset(array=w3686, new element=TRUE ("new element/subarray"), index=w3684) -> (w3685:bool[])
            n770 = local write "Swch Box"(w3685) -> ()
            n771 = Unbundle By Name(w3695) -> ("status"=w3688:bool)
          }
          frame "Set Signal Select Relays" {
            w3718 = 3  # SignalSel
            # "Set Signal Select Relays"
            n772 = Array Subset(array=w3744, index=1, length=2) -> (w3727:bool[])
            n773 = local read "Swch Box"() -> (w3720:bool[])
            n774 = call "Switch Box Signal Select Control.vi"("Signal"=w3731, "Dout Inv"=w3727, "ErrIn"=w3729, "SimOn"=w3730) -> ("ErrOut"=w3728:errorcluster)  [unwired: 11 in]
            n775 = Replace Array Subset(array=w3720, new element=TRUE ("new element/subarray"), index=w3718) -> (w3719:bool[])
            n776 = local write "Swch Box"(w3719) -> ()
            n777 = Unbundle By Name(w3728) -> ("status"=w3722:bool)
          }
          frame "Stop" {
            w3790 = 0 ("Samps/Chl")
            # "Stop -  main program terminated"
            n778 = case shown="6" w3792 {
              selector: w3792 -> [w3801 w3812 w3831 w3847 w3863 w3878 w3890 _ w3915]
              tunnel: [w3800 w3805 w3830 w3846 w3862 w3877 w3889 w3900 w3915] -> w3791
              tunnel: [FALSE FALSE FALSE FALSE FALSE FALSE FALSE FALSE TRUE] -> w3785
              tunnel: w3779 -> [w3798 w3807 w3829 w3835 w3851 w3876 w3888 w3904 w3919]
              tunnel: [T4."Generator OFF" ("State") T4."Wait x Secs" ("State") T4."Wait x Secs" ("State") w3835 w3851 w3876 w3888 w3904 w3919] -> w3778
              tunnel: [w3798 w3807 w3829 w3835 w3851 w3876 w3888 w3904 w3919] -> w3777
              tunnel: [w3798 w3807 w3829 w3835 w3851 w3876 w3888 w3904 w3919] -> w3776
              tunnel: [w3797 w3811 w3816 w3834 w3850 w3875 w3885 w3902 w3917] -> w3769
              tunnel: w3768 -> [_ w3810 w3817 _ _ _ _ _ _]
              tunnel: w3767 -> [w3797 _ _ w3834 w3850 w3875 w3885 w3902 w3917]
              tunnel: w3766 -> [w3796 w3806 w3828 w3845 w3861 w3874 w3886 w3903 w3918]
              tunnel: [w3796 w3806 w3827 w3844 w3860 w3873 w3886 w3903 w3918] -> w3765
              tunnel: w3764 -> [_ _ w3826 w3843 w3859 w3872 _ _ _]
              tunnel: w3763 -> [_ _ w3822 w3839 w3855 w3869 _ _ _]
              tunnel: w3762 -> [w3794 w3803 w3814 w3833 w3849 w3865 w3884 w3897 w3913]
              tunnel: w3761 -> [_ _ _ _ _ _ w3883 _ _]
              tunnel: w3760 -> [w3793 w3802 w3813 w3832 w3848 w3864 w3879 w3906 w3912]
              tunnel: w3759 -> [_ _ _ _ _ _ _ w3905 _]
              tunnel: w3757 -> [_ _ _ _ _ _ w3881 w3898 _]
              tunnel: [w3794 w3803 w3814 w3833 w3849 w3865 w3880 w3897 w3913] -> w3756
              tunnel: [w3793 w3802 w3813 w3832 w3848 w3864 w3879 w3896 w3912] -> w3755
              frame 0, Default {
                # "0 - Generator OFF"
                n779 = Increment(x=w3801) -> (x+1=w3800:i32)
              }
              frame 1 {
                w3808 = 0.5  # 0.5-sec
                # "1 - small delay"
                n780 = Add(x=w3808, y=w3810) -> (x+y=w3811:dbl)
                n781 = Increment(x=w3812) -> (x+1=w3805:i32)
              }
              frame 2 {
                w3818 = 0.3  # 0.3-sec
                w3820 = TRUE  # All OFF
                w3825 = TRUE  # Stop
                # "2 - Cell Select OFF"
                n782 = Array Subset(array=w3822, index=8, length=4) -> (w3821:bool[])
                n783 = call "Switch Box Cell Select Control.vi"("All OFF"=w3820, "Dout Inv"=w3821, "ErrIn"=w3828, "SimOn"=w3826, "Stop"=w3825) -> ("ErrOut"=w3827:errorcluster)  [unwired: 10 in]
                n784 = Add(x=w3818, y=w3817) -> (x+y=w3816:dbl)
                n785 = Increment(x=w3831) -> (x+1=w3830:i32)
              }
              frame 3 {
                w3837 = TRUE  # All OFF
                w3842 = TRUE  # Stop
                # "3 - Resistor Select OFF"
                n786 = Array Subset(array=w3839, index=5, length=3) -> (w3838:bool[])
                n787 = call "Switch Box Resistor Select Control.vi"("All OFF"=w3837, "Dout Inv"=w3838, "ErrIn"=w3845, "SimOn"=w3843, "Stop"=w3842) -> ("ErrOut"=w3844:errorcluster)  [unwired: 10 in]
                n788 = Increment(x=w3847) -> (x+1=w3846:i32)
              }
              frame 4 {
                w3853 = TRUE  # All OFF
                w3858 = TRUE  # Stop
                # "4 - Signal Select OFF"
                n789 = Array Subset(array=w3855, index=1, length=2) -> (w3854:bool[])
                n790 = call "Switch Box Signal Select Control.vi"("All OFF"=w3853, "Dout Inv"=w3854, "ErrIn"=w3861, "SimOn"=w3859, "Stop"=w3858) -> ("ErrOut"=w3860:errorcluster)  [unwired: 10 in]
                n791 = Increment(x=w3863) -> (x+1=w3862:i32)
              }
              frame 5 {
                w3867 = FALSE  # Auto OFF
                w3871 = TRUE  # Stop
                # "5 - Auto Mode OFF"
                n792 = Index Array(array=w3869, index=4) -> (element=w3868:bool)
                n793 = call "Switch Box Auto Mode Control.vi"("OFF/ON"=w3867, "Invert"=w3868, "ErrIn"=w3874, "SimOn"=w3872, "Stop"=w3871) -> ("ErrOut"=w3873:errorcluster)  [unwired: 10 in]
                n794 = Increment(x=w3878) -> (x+1=w3877:i32)
              }
              frame 6 {
                # "6 - Agilent close"
                n795 = case shown="True" w3881 {
                  tunnel: w3884 -> [w3891 w3894]
                  tunnel: w3883 -> [_ w3893]
                  tunnel: [w3891 refnum<visa-resource-name> refnum ("dup VISA session")] -> w3880
                  frame False {
                  }
                  frame True {
                    n796 = case shown="False" w3893 {
                      tunnel: w3894 -> [w3895 _]
                      frame False {
                        n797 = call "ag33xxx - Close.vi"("VISA session"=w3895) -> ()  [unwired: 10 in, 1 out]
                      }
                      frame True {
                        # "Sim"
                      }
                    }
                  }
                }
                n798 = global write "Global ER2007.vi" "GCD Prog"(bool[] [FALSE, FALSE, FALSE, FALSE, TRUE, FALSE] ("GCD Prog")) -> ()
                n799 = Increment(x=w3890) -> (x+1=w3889:i32)
              }
              frame 7 {
                w3900 = 15  # Done
                # "7 - close NAII"
                n800 = case shown="False" w3898 {
                  tunnel: w3906 -> [w3907 w3910]
                  tunnel: w3905 -> [_ w3909]
                  tunnel: [w3907 refnum<visa-resource-name> refnum ("instrument handle out")] -> w3896
                  frame False {
                  }
                  frame True {
                    n801 = case shown="False" w3909 {
                      tunnel: w3910 -> [w3911 _]
                      frame False {
                        n802 = VISA Close(VISA resource name=w3911) -> ()  [unwired: 1 in, 1 out]
                      }
                      frame True {
                      }
                    }
                  }
                }
                n803 = global write "Global ER2007.vi" "GCD Prog"(bool[] [FALSE, FALSE, FALSE, FALSE, FALSE, TRUE] ("GCD Prog")) -> ()
              }
              frame 15 {
                # "15 - all done"
                n804 = global write "Global ER2007.vi" "GCD Prog"(bool[] [FALSE, FALSE, FALSE, FALSE, FALSE, FALSE] ("GCD Prog")) -> ()
              }
            }
          }
          frame "Wait x Secs" {
            # "Wait x Secs"
            n805 = Greater?(x=w3937, y=w3947) -> (0:w3946:bool)
            n806 = case shown="\"Abort\", Default" w3924 {
              tunnel: w3923 -> [w3954 _]
              tunnel: [w3954 FALSE] -> w3922
              frame "Abort", Default {
              }
              frame "Stop" {
              }
            }
            n807 = case shown="True" w3946 {
              tunnel: w3943 -> [w3957 w3959]
              tunnel: w3942 -> [_ _]
              tunnel: w3924 -> [w3956 w3958]
              tunnel: [w3956 w3958] -> w3941
              tunnel: [w3957 w3959] -> w3940
              tunnel: [w3957 w3958] -> w3939
              frame False {
              }
              frame True {
              }
            }
          }
        }
        "Resistivity Data" <- w178
        "State" <- w155
        "PriPh" <- w176
        "SecPh" <- w177
        "B 3" <- w174
        "NAI Errcnt" <- w164
        n808 = case shown="False" w174 {
          tunnel: w155 -> [w221 _]
          tunnel: [w221 T4."Abort" ("State")] -> w203
          tunnel: [w222 w226] -> w202
          tunnel: [w223 w225] -> w201
          tunnel: w200 -> [w223 w225]
          tunnel: w199 -> [w222 w226]
          frame False {
          }
          frame True {
          }
        }
      }
      n809 = node-c288(w126) -> ()  [unwired: 1 out]
    }
    frame #2 {
      # "Cleanup and shutdown"
      n810 = stacked-sequence {
        tunnel: w3964 -> [_ _]
        tunnel: w3963 -> [_ _]
        frame #0 {
        }
        frame #1 {
          w3965 = FALSE ("GCD Run")
          n811 = global write "Global ER2007.vi" "GCD Run"(w3965) -> ()
          n812 = global write "Global ER2007.vi" "GCD Busy"(w3965) -> ()
          n813 = global write "Global ER2007.vi" "GCD Stop"(w3965) -> ()
          n814 = local write "Stop"(w3965) -> ()
        }
      }
    }
  }
